vi "User Manual.vi"() -> ()   [LabVIEW 2020, in "Exaprom PDF.lvlib"]
uses:
  <userlib>/labview-PDF-writer-master/Exaprom PDF.lvlib
  <userlib>/labview-PDF-writer-master/Controls/Page Controls/Page setup.ctl
  <userlib>/labview-PDF-writer-master/Controls/Page Controls/Page size.ctl
  <userlib>/labview-PDF-writer-master/Controls/Page Controls/Page Orientation.ctl
  <userlib>/labview-PDF-writer-master/Controls/Page Controls/Page Layout Custom.ctl
  <userlib>/labview-PDF-writer-master/Controls/Page Controls/Page margins.ctl
  <userlib>/labview-PDF-writer-master/Controls/Font Controls/Font complete cluster.ctl
  <userlib>/labview-PDF-writer-master/Controls/Font Controls/Font size.ctl
  <userlib>/labview-PDF-writer-master/Controls/Font Controls/Font color.ctl
  <userlib>/labview-PDF-writer-master/Controls/Font Controls/Type and encoding.ctl
  <userlib>/labview-PDF-writer-master/Controls/Text Controls/Unicode/Type and run direction.ctl
  <userlib>/labview-PDF-writer-master/Controls/Initialization Controls/Defaut Paragraphe and Line Spacing.ctl
  <userlib>/labview-PDF-writer-master/Controls/Text Controls/Texte alignement.ctl
  <userlib>/labview-PDF-writer-master/Controls/Text Controls/Line spacing.ctl
  <userlib>/labview-PDF-writer-master/Controls/Table Controls/Table properties.ctl
  <userlib>/labview-PDF-writer-master/Controls/Table Controls/Table position.ctl
  <userlib>/labview-PDF-writer-master/Controls/Initialization Controls/PDF Details.ctl
  <userlib>/labview-PDF-writer-master/Controls/Header, Footer and Watermark Controls/Header or Footer  Image cluster.ctl
  <userlib>/labview-PDF-writer-master/Controls/Table Controls/Cell Alignment 20px.ctl
  <userlib>/labview-PDF-writer-master/Controls/Header, Footer and Watermark Controls/Header or Footer  Page # cluster.ctl
  <userlib>/labview-PDF-writer-master/Controls/Header, Footer and Watermark Controls/Page number.ctl
  <userlib>/labview-PDF-writer-master/Controls/Font Controls/Font complete cluster horizontal.ctl
  <userlib>/labview-PDF-writer-master/Controls/Header, Footer and Watermark Controls/Header or Footer Line cluster.ctl
  <userlib>/labview-PDF-writer-master/Controls/Header, Footer and Watermark Controls/Header Footer Line.ctl
  <userlib>/labview-PDF-writer-master/Controls/Header, Footer and Watermark Controls/Header or Footer  Text cluster.ctl
  <userlib>/labview-PDF-writer-master/Controls/Initialization Controls/Captions.ctl
  <userlib>/labview-PDF-writer-master/Controls/Initialization Controls/Image or Table Caption.ctl
  <userlib>/labview-PDF-writer-master/Controls/Initialization Controls/Unit.ctl
  <userlib>/labview-PDF-writer-master/Controls/Text Controls/Text and hyperlink [ ].ctl
  <userlib>/labview-PDF-writer-master/Controls/Text Controls/Text from String of File and hyperlink.ctl
  <userlib>/labview-PDF-writer-master/Controls/Text Controls/Paragraph indentation.ctl
  <userlib>/labview-PDF-writer-master/Controls/Image Controls/Image alignment and position.ctl
  <userlib>/labview-PDF-writer-master/Controls/Image Controls/Image aligment.ctl
  <userlib>/labview-PDF-writer-master/Controls/Image Controls/Image border.ctl
  <userlib>/labview-PDF-writer-master/Controls/Table Controls/Row Predefined borders cluster.ctl
  <userlib>/labview-PDF-writer-master/Controls/Table Controls/Row Predefined borders.ctl
  <userlib>/labview-PDF-writer-master/Controls/Image Controls/Image Scale.ctl
  <userlib>/labview-PDF-writer-master/Controls/Table Controls/Cell Font, type, Alignment and LS V2.ctl
  <userlib>/labview-PDF-writer-master/Controls/Table Controls/Cell Type, Alignment and LS.ctl
  <userlib>/labview-PDF-writer-master/Controls/Table Controls/Text vertical arrangement.ctl
  <userlib>/labview-PDF-writer-master/Controls/Table Controls/Row Back Ground color Datas.ctl
  <userlib>/labview-PDF-writer-master/Controls/Header, Footer and Watermark Controls/Watermark Text Cluster.ctl
  <userlib>/labview-PDF-writer-master/Controls/Header, Footer and Watermark Controls/Watermark Position.ctl
  <userlib>/labview-PDF-writer-master/Controls/Header, Footer and Watermark Controls/Header footer horiz alignment.ctl
  <userlib>/labview-PDF-writer-master/Controls/Header, Footer and Watermark Controls/Watermark Image Cluster.ctl
  <userlib>/labview-PDF-writer-master/Controls/Table Controls/Simplified Table Row Borders [ ].ctl
  <userlib>/labview-PDF-writer-master/Controls/Table Controls/Simplified Table Row Borders.ctl
  <userlib>/labview-PDF-writer-master/Controls/Table Controls/Border and BG Color [ ].ctl
  <userlib>/labview-PDF-writer-master/Controls/Table Controls/Border and BG Color.ctl
  <userlib>/labview-PDF-writer-master/Controls/Table Controls/Cell Border 20 px.ctl
  <userlib>/labview-PDF-writer-master/Controls/Concatenate Controls/PDF file to concatenate.ctl
  <userlib>/labview-PDF-writer-master/Controls/Table Controls/Table Appearance and Font Row [ ].ctl
  <userlib>/labview-PDF-writer-master/Controls/Table Controls/One Row Appearance.ctl
  <userlib>/labview-PDF-writer-master/Controls/Table Controls/Row from to.ctl
  <userlib>/labview-PDF-writer-master/Controls/Table Controls/Cell, Alignment, LS and Font - hide Vmerge.ctl
  <userlib>/labview-PDF-writer-master/Controls/Table Controls/Cell Appearance.ctl
  <userlib>/labview-PDF-writer-master/Controls/Table Controls/Merge Horizontal.ctl
  <userlib>/labview-PDF-writer-master/Controls/Table Controls/Merge Vertical.ctl
  <userlib>/labview-PDF-writer-master/Controls/Initialization Controls/File Permission Parameters.ctl
  <userlib>/labview-PDF-writer-master/Controls/Initialization Controls/At the opening.ctl
  <vilib>/Utility/miscctls.llb/LVPointTypeDef.ctl
  <userlib>/labview-PDF-writer-master/Controls/Header, Footer and Watermark Controls/Header or Footer.ctl
  <userlib>/labview-PDF-writer-master/Controls/Chapter Controls/Chapter.ctl
  <userlib>/labview-PDF-writer-master/Controls/Image Controls/Image Size Block Diagram.ctl
  <userlib>/labview-PDF-writer-master/VIs/Low level/Header, Footer and Watermark Low level/Append Text HF.vi
  <userlib>/labview-PDF-writer-master/VIs/Low level/Header, Footer and Watermark Low level/AppendLine seperator.vi
  <userlib>/labview-PDF-writer-master/VIs/Low level/Header, Footer and Watermark Low level/Append Image HF.vi
  <userlib>/labview-PDF-writer-master/VIs/Low level/Header, Footer and Watermark Low level/Append Page number HF.vi
  <userlib>/labview-PDF-writer-master/VIs/Low level/Header, Footer and Watermark Low level/Append Watermark Image.vi
  <userlib>/labview-PDF-writer-master/VIs/Low level/Header, Footer and Watermark Low level/Append Watermark Text.vi
  <userlib>/labview-PDF-writer-master/VIs/Text/Append Paragraph with Link [ ].vi
  <userlib>/labview-PDF-writer-master/VIs/Text/Append Paragraph.vi
  <userlib>/labview-PDF-writer-master/VIs/Text/Append Phrase.vi
  <userlib>/labview-PDF-writer-master/LV Class/PDF Report Class/PDF Report Class.lvclass
panel:
  out "Tab Control":T1(tab)=enum."Table 5"
  in  "Page Setup":T2={"Page Size"=1, "Orientation"=enum."Portrait", "Custom Size"={"Width"=0.0, "Height"=0.0}, "Margins"={"Left"=1.0, "Right"=1.0, "Top"=1.0, "Bottom"=1.0}} caption="页面设置" {"Page Size" items=["Custom", "LETTER", "NOTE", "LEGAL", "TABLOID", "EXECUTIVE", "POSTCARD", "A0", "A1", "A2", "A3", "A4", "A5", "A6", "A7", "A8", "A9", "A10", "B0", "B1", "B2", "B3", "B4", "B5", "B6", "B7", "B8", "B9", "B10", "ARCH_E", "ARCH_D", "ARCH_C", "ARCH_B", "ARCH_A", "FLSA", "FLSE", "HALFLETTER", "_11X17", "ID_1", "ID_2", "ID_3", "LEDGER", "CROWN_QUARTO", "LARGE_CROWN_QUARTO", "DEMY_QUARTO", "ROYAL_QUARTO", "CROWN_OCTAVO", "LARGE_CROWN_OCTAVO", "DEMY_OCTAVO", "ROYAL_OCTAVO", "SMALL_PAPERBACK", "PENGUIN_SMALL_PAPERBACK", "PENGUIN_LARGE_PAPERBACK"]}
  in  "Default Paragraph":T7={" Aligment"=enum."JUSTIFY", "Line spacing"=enum."1.0"} caption="默认段落"
  out "error out":errorcluster
  in  "PDF Details":T10={"Title"="Exaprom PDF 2.0的用户手册", "Author"="三多", "Subject"="这个示例展示了如何使用工具箱Exaprom PDF 2.0创建PDF报告。", "Keywords"="关键词.", "Creator"="Exaprom PDF 2.0"} caption="PDF 详情"
  in  "File or Directory path":path=path "C:/Users/10643/Desktop/123.pdf"
  out "PDF 输出路径":path=path "C:/Users/10643/Desktop/123_22112416.pdf"
  in  "默认字体":T11={"Name"="Arial", "Size"=12.0, "Color"=0, "Style"={"Bold"=FALSE, "Italic"=FALSE, "Underline"=FALSE, "Strikeout"=FALSE}, "Type"={"Type&direction"=enum."ASCII", "Embedded"=FALSE, "Encoding"="gb2312"}}
  in  "Captions":T16={"Figure"={"Caption"="Figure ", "Separator"=":  ", "Position"=enum."Below"}, "Table"={"Caption"="Table ", "Separator"=":  ", "Position"=enum."Above"}, "Font"={"Name"="", "Size"=-1.0, "Color"=0, "Style"={"Bold"=FALSE, "Italic"=FALSE, "Underline"=FALSE, "Strikeout"=FALSE}, "Type"={"Type&direction"=enum."Select", "Embedded"=FALSE, "Encoding"=""}}} caption="标题"
  in  "Unit (默认 = 英寸)":T18 caption="单位 (默认 = 英寸)"
  in  "Overwrite?":bool=TRUE
  out "Progress":u8(slide)=20 scale=0.0..20.0
  in  "Permissions":T19={"User Password"="", "Owner Password"="", "Printing"=enum."Don't Allow Printing", "Allow Modify Contents"=FALSE, "Allow Copy"=FALSE, "Allow Modify Annotations"=FALSE, "Allow Fill In "=FALSE, "Allow Screen Readers"=FALSE, "Allow Assembly"=FALSE} caption="权限"
  in  "At the opening":T20={"Page"=0, "Show Bookmarks"=TRUE} caption="PDF显示方式(自动适应 高，宽显示)" {"Page" items=["Single Page - Fit Page"=1, "Single Page - Fit Width"=0]}
  out "秒":u32=2
  in  "Watermark":enum16{"none", "Image", "Text"}(ring) caption="选择水印方式"
  in  "Footer Page #":T21={"Start at page"=3, "Start with #"=1, "Cell Alignment"=6, "Page #"={"Text 1"="页", "Text 2"="到", "Text 3"="页"}, "Font"={"Name"="Arial", "Size"=10.0, "Color"=0, "Style"={"Bold"=FALSE, "Italic"=FALSE, "Underline"=FALSE, "Strikeout"=FALSE}, "Type"={"Type&direction"=enum."ASCII", "Embedded"=FALSE, "Encoding"=""}}} caption="页码 #"
  in  "Footer Line":T25={"H/F Line"=enum."Horizontal line", "Thickness (point)"=0.75, " Colour"=7171459} caption="页脚线"
  in  "Header Line":T25={"H/F Line"=enum."Horizontal line", "Thickness (point)"=0.75, " Colour"=7171459} caption="页眉线"
  in  "Header Text":T27={"Start at page"=3, "Cell Alignment"=5, "Line spacing"=enum."Select", "Text"="Exaprom PDF 2.0 LabVIEW工具箱\n(with <a>iTextSharp</a> 4.1.6)", "Font complete"={"Name"="", "Size"=14.0, "Color"=0, "Style"={"Bold"=TRUE, "Italic"=FALSE, "Underline"=FALSE, "Strikeout"=FALSE}, "Type"={"Type&direction"=enum."Select", "Embedded"=FALSE, "Encoding"=""}}, "Link"="http://"} caption="标题内容"
  in  "Footer Text":T27={"Start at page"=3, "Cell Alignment"=4, "Line spacing"=enum."Select", "Text"="WWW.OK.SHOW", "Font complete"={"Name"="Segoe Script", "Size"=8.0, "Color"=16711680, "Style"={"Bold"=TRUE, "Italic"=TRUE, "Underline"=FALSE, "Strikeout"=FALSE}, "Type"={"Type&direction"=enum."Select", "Embedded"=FALSE, "Encoding"=""}}, "Link"="http://WWW.OK.SHOW"} caption="页脚文本"
  in  "Watermark Image":T28={"Image path"=path "C:/Program Files (x86)/National Instruments/LabVIEW 2020/user.lib/labview-PDF-writer-master/Examples/Images/Logo Exaprom.jpg", "Opacity (%)"=10.0, "Postion"={"Position"=enum."Center (text section)", "X"=0.0, "Y"=0.0}, "Automatic"=TRUE, "Scale(%)"=100.0, "Rotate(°)"=0.0} caption="水印图像"
  in  "Watermark Text":T30={"Text "="WWW.OK.SHOW", "Opacity (%)"=5.0, "Position"={"Position"=enum."Center (text section)", "X"=0.0, "Y"=0.0}, "Automatic"=TRUE, "Font"={"Font Name"="", "Size"=-1.0, "Color"=0}, "Alignment"=enum."Center", "Rotate(°)"=0.0} caption="水印文本"
  in  "Footer Image":T32={"Start at page"=3, "Cell Alignment"=5, "Path"=path "C:/Program Files (x86)/National Instruments/LabVIEW 2020/user.lib/labview-PDF-writer-master/Examples/Images/Logo Exaprom.jpg", "Image (%)"=15.0, "Link"="http://WWW.OK.SHOW"} caption="页脚图像"
  in  "Text FP1 [ ]":T33=[{"Text"={"Text"="\nExaprom PDF 2.0工具包  \n\n \n\n用户手册 \n\n", "Path"=path "", "Font complete"={"Name"="Arial", "Size"=32.0, "Color"=0, "Style"={"Bold"=TRUE, "Italic"=FALSE, "Underline"=FALSE, "Strikeout"=FALSE}, "Type"={"Type&direction"=enum."ASCII", "Embedded"=FALSE, "Encoding"=""}}}, "Link"={"Hyperlink"="", "Font complete"={"Name"="", "Size"=-1.0, "Color"=255, "Style"={"Bold"=FALSE, "Italic"=TRUE, "Underline"=FALSE, "Strikeout"=FALSE}, "Type"={"Type&direction"=enum."Select", "Embedded"=FALSE, "Encoding"=""}}}, "Paragraphe"={" Aligment"=enum."CENTER", "Line spacing"=enum."Select"}, "Indentation"={"Left"=0.0, "Right"=0.0}}, {"Text"={"Text"="\nPDF Report with iTextSharp 4.1.6\nfor LabVIEW", "Path"=path "", "Font complete"={"Name"="Arial", "Size"=24.0, "Color"=0, "Style"={"Bold"=TRUE, "Italic"=FALSE, "Underline"=FALSE, "Strikeout"=FALSE}, "Type"={"Type&direction"=enum."Select", "Embedded"=FALSE, "Encoding"=""}}}, "Link"={"Hyperlink"="", "Font complete"={"Name"="", "Size"=-1.0, "Color"=255, "Style"={"Bold"=FALSE, "Italic"=TRUE, "Underline"=FALSE, "Strikeout"=FALSE}, "Type"={"Type&direction"=enum."Select", "Embedded"=FALSE, "Encoding"=""}}}, "Paragraphe"={" Aligment"=enum."CENTER", "Line spacing"=enum."Select"}, "Indentation"={"Left"=0.0, "Right"=0.0}}, {"Text"={"Text"="\n\n\n\nby\n\nJean-Marc Simard \n三多（修复汉化)\nQQ：1064331064\n\n\n\n七月-08日-二〇二二年", "Path"=path "", "Font complete"={"Name"="Arial", "Size"=24.0, "Color"=0, "Style"={"Bold"=FALSE, "Italic"=FALSE, "Underline"=FALSE, "Strikeout"=FALSE}, "Type"={"Type&direction"=enum."Select", "Embedded"=FALSE, "Encoding"=""}}}, "Link"={"Hyperlink"="", "Font complete"={"Name"="", "Size"=-1.0, "Color"=255, "Style"={"Bold"=FALSE, "Italic"=TRUE, "Underline"=FALSE, "Strikeout"=FALSE}, "Type"={"Type&direction"=enum."Select", "Embedded"=FALSE, "Encoding"=""}}}, "Paragraphe"={" Aligment"=enum."CENTER", "Line spacing"=enum."Select"}, "Indentation"={"Left"=0.0, "Right"=0.0}}]
  in  "Image FP1":path=path "C:/Program Files/National Instruments/LabVIEW 2009/vi.lib/Exaprom PDF/Examples/Images/Logo Exaprom.jpg"
  in  "TOC Title":string="\n目录\n\n\n"
  in  "TOC Title Font":T11={"Name"="", "Size"=14.0, "Color"=0, "Style"={"Bold"=TRUE, "Italic"=FALSE, "Underline"=FALSE, "Strikeout"=FALSE}, "Type"={"Type&direction"=enum."ASCII", "Embedded"=FALSE, "Encoding"=""}} caption="TOC标题字体"
  in  "TOC Chapter and section Font":T11={"Name"="", "Size"=-1.0, "Color"=0, "Style"={"Bold"=FALSE, "Italic"=FALSE, "Underline"=FALSE, "Strikeout"=FALSE}, "Type"={"Type&direction"=enum."ASCII", "Embedded"=FALSE, "Encoding"=""}} caption="TOC章和节字体"
  in  "Text C8":string="\n虽然这个工具包并没有打算取代文字处理程序，但是作为一个例子，我们使用这个PDF工具包制作了这个文档。VI“用户手册”。vi”在面板“Exaprom PDF 2.0”中可用。"
  in  "Texte C2 [ ]":T33=[{"Text"={"Text"="\n我开发了这个PDF报告生成工具包，因为我希望能够在LabVIEW上生成PDF报告，而不需要购买许可证。 最终的选择是开源的iTextSharp 4.1.6库(<a>Mozilla Public License Version 1.1</a>)。 我开发了一系列VIs，使我可以直接生成PDF报告，而不需要购买商业产品。 选择的许可: \n", "Path"=path "", "Font complete"={"Name"="", "Size"=-1.0, "Color"=0, "Style"={"Bold"=FALSE, "Italic"=FALSE, "Underline"=FALSE, "Strikeout"=FALSE}, "Type"={"Type&direction"=enum."Select", "Embedded"=FALSE, "Encoding"=""}}}, "Link"={"Hyperlink"="http://www.mozilla.org/MPL/MPL-1.1.html", "Font complete"={"Name"="", "Size"=-1.0, "Color"=255, "Style"={"Bold"=FALSE, "Italic"=TRUE, "Underline"=FALSE, "Strikeout"=FALSE}, "Type"={"Type&direction"=enum."Select", "Embedded"=FALSE, "Encoding"=""}}}, "Paragraphe"={" Aligment"=enum."Select", "Line spacing"=enum."Select"}, "Indentation"={"Left"=0.0, "Right"=0.0}}, {"Text"={"Text"="\n<a>BSD(伯克利软件发布许可)</a>允许专有使用，并且对于在该许可下发布的软件可以并入专有产品。 基于该软件作品可以在专有许可下发布或作为封闭源代码软件。”\n", "Path"=path "", "Font complete"={"Name"="", "Size"=-1.0, "Color"=0, "Style"={"Bold"=FALSE, "Italic"=FALSE, "Underline"=FALSE, "Strikeout"=FALSE}, "Type"={"Type&direction"=enum."Select", "Embedded"=FALSE, "Encoding"=""}}}, "Link"={"Hyperlink"="http://fr.wikipedia.org/wiki/Licence_BSD", "Font complete"={"Name"="", "Size"=-1.0, "Color"=255, "Style"={"Bold"=FALSE, "Italic"=TRUE, "Underline"=FALSE, "Strikeout"=FALSE}, "Type"={"Type&direction"=enum."Select", "Embedded"=FALSE, "Encoding"=""}}}, "Paragraphe"={" Aligment"=enum."Select", "Line spacing"=enum."Select"}, "Indentation"={"Left"=0.5, "Right"=0.5}}, {"Text"={"Text"="\n简单地说，你可以对这些VIs做你想做的。\n\n更新的版本，<a>iTextSharp 5。X<a>，在Affero通用公共许可证下，在不披露您自己的应用程序源代码的情况下，涉及iText软件的活动是不免费的。\n\n\n", "Path"=path "", "Font complete"={"Name"="", "Size"=-1.0, "Color"=0, "Style"={"Bold"=FALSE, "Italic"=FALSE, "Underline"=FALSE, "Strikeout"=FALSE}, "Type"={"Type&direction"=enum."Select", "Embedded"=FALSE, "Encoding"=""}}}, "Link"={"Hyperlink"="http://itextpdf.com/terms-of-use/", "Font complete"={"Name"="", "Size"=-1.0, "Color"=255, "Style"={"Bold"=FALSE, "Italic"=TRUE, "Underline"=FALSE, "Strikeout"=FALSE}, "Type"={"Type&direction"=enum."Select", "Embedded"=FALSE, "Encoding"=""}}}, "Paragraphe"={" Aligment"=enum."Select", "Line spacing"=enum."Select"}, "Indentation"={"Left"=0.0, "Right"=0.0}}]
  in  "Texte D2 [ ]":T33=[{"Text"={"Text"="\n\nPDF报告的制作可分为四个步骤:\n\n1)创建报告(PDF文件和默认参数)\n2)添加页眉、页脚和水印(全部可选)\n3)撰写PDF报告，包括添加文本元素、图片(文件、\n控制和前面板)和桌子;\n4)关闭PDF报告\n\n在第5章中，我们回顾了创建PDF报告所需的不同VI。\n\n", "Path"=path "", "Font complete"={"Name"="", "Size"=-1.0, "Color"=0, "Style"={"Bold"=FALSE, "Italic"=FALSE, "Underline"=FALSE, "Strikeout"=FALSE}, "Type"={"Type&direction"=enum."Select", "Embedded"=FALSE, "Encoding"=""}}}, "Link"={"Hyperlink"="", "Font complete"={"Name"="", "Size"=-1.0, "Color"=255, "Style"={"Bold"=FALSE, "Italic"=TRUE, "Underline"=FALSE, "Strikeout"=FALSE}, "Type"={"Type&direction"=enum."Select", "Embedded"=FALSE, "Encoding"=""}}}, "Paragraphe"={" Aligment"=enum."Select", "Line spacing"=enum."Select"}, "Indentation"={"Left"=0.0, "Right"=0.0}}]
  in  "Text C6":string="重启LabVIEW后，面板“Exaprom PDF 2.0”将出现。\n\n"
  in  "Text C1":string="产品介绍"
  in  "Text C3":string="产品介绍"
  in  "Texte C4 [ ]":T33=[{"Text"={"Text"="\n解压“ExapromPDF2.0.ZIP”之后，您将得到一个文件夹和一个文件\n\n     1)\tExaprom PDF文件夹;\n     2)\t还有exaprompdf.mnu文件。\n\n\n", "Path"=path "", "Font complete"={"Name"="", "Size"=-1.0, "Color"=0, "Style"={"Bold"=FALSE, "Italic"=FALSE, "Underline"=FALSE, "Strikeout"=FALSE}, "Type"={"Type&direction"=enum."Select", "Embedded"=FALSE, "Encoding"=""}}}, "Link"={"Hyperlink"="", "Font complete"={"Name"="", "Size"=-1.0, "Color"=16777222, "Style"={"Bold"=TRUE, "Italic"=FALSE, "Underline"=FALSE, "Strikeout"=FALSE}, "Type"={"Type&direction"=enum."Select", "Embedded"=FALSE, "Encoding"=""}}}, "Paragraphe"={" Aligment"=enum."LEFT", "Line spacing"=enum."Select"}, "Indentation"={"Left"=0.0, "Right"=0.0}}]
  in  "Text C5":string="\n\n“Exaprom PDF”文件夹必须放在(参见图2):\n\nC:\\Program Files\\National Instruments\\LabVIEW Version\\vi.lib\\\n\n"
  in  "Text C7":string="\nexaprompdf文件”.Mnu \"必须放在(见图3):\n\nC:\\Program Files\\National Instruments\\LabVIEW Version\\\n                                                                                     menus\\Categories\\Programming\\"
  in  "Text D1":string="PDF报告(简化)"
  in  "Texte E2 [ ]":T33=[{"Text"={"Text"="\n\n用于生成PDF报告的库是iTextSharp。\n\n本库使用点(72点= 1英寸= 25.4毫米)，但您将使用您选择的单位(英寸或毫米-章节5.4)，除非单位“点”被明确指出。字体是个例外:单位就是点。\n\n页面的原点在左下角(见下图)。\n\n文本框是减去页边距(下图中的蓝色矩形)的页面。\n\n\n", "Path"=path "", "Font complete"={"Name"="", "Size"=-1.0, "Color"=0, "Style"={"Bold"=FALSE, "Italic"=FALSE, "Underline"=FALSE, "Strikeout"=FALSE}, "Type"={"Type&direction"=enum."Select", "Embedded"=FALSE, "Encoding"=""}}}, "Link"={"Hyperlink"="", "Font complete"={"Name"="", "Size"=-1.0, "Color"=255, "Style"={"Bold"=FALSE, "Italic"=TRUE, "Underline"=FALSE, "Strikeout"=FALSE}, "Type"={"Type&direction"=enum."Select", "Embedded"=FALSE, "Encoding"=""}}}, "Paragraphe"={" Aligment"=enum."Select", "Line spacing"=enum."Select"}, "Indentation"={"Left"=0.0, "Right"=0.0}}]
  in  "Text E1":string="一般"
  in  "Text F2":string="“文本”面板"
  in  "Text F1":string="不同的调色板"
  in  "Texte F3 [ ]":T33=[{"Text"={"Text"="\n\n您可以访问目录中包含的字体C: \\ Windows \\ Fonts (你应该检查版权). 此外，你还有iTextSharp自动提供的字体:Courier, Helvetica, Symbol, Times-Roman和ZapfDingbats。\n\n当创建PDF报告时，我们指定默认字体为Arial 12点(粗体、斜体、下划线和删除线= F)，类型和方向= ASCII，字符编码= CP1252(拉丁字母)。该信息存储在LV类“PDF报告”中。文本面板中所有VI的字体参数为:\n\n- Name =空字符串;\n- Size = -1;\n-粗体，斜体，下划线和删除线= F;\n-类型&方向=选择;\n- E(内嵌)= F;\n- Encoding =空字符串。\n\n当字体名称为空时，将使用默认字体的名称。当字体大小的值为-1时，则使用默认的字体大小。当Type&direction的值设置为Select时，将使用默认字体的Type&direction。当Encoding的值为空时，将使用默认字体的Encoding。\n", "Path"=path "", "Font complete"={"Name"="", "Size"=-1.0, "Color"=0, "Style"={"Bold"=FALSE, "Italic"=FALSE, "Underline"=FALSE, "Strikeout"=FALSE}, "Type"={"Type&direction"=enum."Select", "Embedded"=FALSE, "Encoding"=""}}}, "Link"={"Hyperlink"="", "Font complete"={"Name"="", "Size"=-1.0, "Color"=255, "Style"={"Bold"=FALSE, "Italic"=TRUE, "Underline"=FALSE, "Strikeout"=FALSE}, "Type"={"Type&direction"=enum."Select", "Embedded"=FALSE, "Encoding"=""}}}, "Paragraphe"={" Aligment"=enum."Select", "Line spacing"=enum."Select"}, "Indentation"={"Left"=0.0, "Right"=0.0}}]
  in  "Text F6":string="在创建PDF报告时，我们指定默认对齐方式为“JUSTIFY”，默认行间距为1.0。该信息也存储在LV类“PDF报告”中。\n\n当对齐方式设置为“选择”时，将使用默认对齐方式。当间距保留为“选择”时，使用默认的行间距。\n\n"
  in  "Text F8 [ ]":T33=[{"Text"={"Text"="此标签允许您像 <img src=\"Arrow\"/> 一样插入图像“Arrow.jpg”。 要插入带有链接 <a><img src=\"Logo\"/></a> 的图像“Logo E.jpg”，您应该使用“Append Paragraph & Link [ ].vi”。 所有这些段落都以换行符自动终止。\n\n", "Path"=path "", "Font complete"={"Name"="", "Size"=-1.0, "Color"=0, "Style"={"Bold"=FALSE, "Italic"=FALSE, "Underline"=FALSE, "Strikeout"=FALSE}, "Type"={"Type&direction"=enum."Select", "Embedded"=FALSE, "Encoding"=""}}}, "Link"={"Hyperlink"="http://www.exaprom.com/", "Font complete"={"Name"="", "Size"=-1.0, "Color"=255, "Style"={"Bold"=FALSE, "Italic"=TRUE, "Underline"=FALSE, "Strikeout"=FALSE}, "Type"={"Type&direction"=enum."Select", "Embedded"=FALSE, "Encoding"=""}}}, "Paragraphe"={" Aligment"=enum."Select", "Line spacing"=enum."Select"}, "Indentation"={"Left"=0.0, "Right"=0.0}}, {"Text"={"Text"="第三个，“Append Phrase.vi”（数字“4”），添加了一个短语，但没有换行符和左对齐。 此外，除了“Append Phrase.vi”之外，还可以有段落缩进（左右）。\n", "Path"=path "", "Font complete"={"Name"="", "Size"=-1.0, "Color"=0, "Style"={"Bold"=FALSE, "Italic"=FALSE, "Underline"=FALSE, "Strikeout"=FALSE}, "Type"={"Type&direction"=enum."Select", "Embedded"=FALSE, "Encoding"=""}}}, "Link"={"Hyperlink"="", "Font complete"={"Name"="", "Size"=-1.0, "Color"=255, "Style"={"Bold"=FALSE, "Italic"=TRUE, "Underline"=FALSE, "Strikeout"=FALSE}, "Type"={"Type&direction"=enum."Select", "Embedded"=FALSE, "Encoding"=""}}}, "Paragraphe"={" Aligment"=enum."Select", "Line spacing"=enum."Select"}, "Indentation"={"Left"=0.0, "Right"=0.0}}]
  in  "Text F7":string="有三个VIs添加文本，他们被分组在VI“追加文本多态”。Vi”(上图中的数字“1”)。\n\n第一个是“附加段落”。Vi“(数字“2”)，可以将文本添加为段落，文本将自动以换行结束。\n\n第二个或“附加段落&链接[]”。Vi\"(数字\"3\")，添加了一个段落序列，该序列具有特殊性，可以将链接(http://www.mywebsite.com/ ou mailto:name@example.com)与文本关联，放置在标签< a> </ a>之间。 \n\n此外，\"Append Paragraph. vi”和Append Paragraph & Link [ ].  Vi\"以在带有标签的段落中插入图像 <img src=\"Image name\"/>.\n"
  in  "Text F5":string="\n字符编码可以是ASCII或Unicode (UTF-16)。写入方向(仅适用于Unicode)为:\n\n- UTF-16 \"UTF-16字符，从左到右书写\";\n——utf - 16(默认)“使用默认运行方向”;\nutf - 16 (LTR)使用从左到右的双向重新排序\n运行方向”;\nutf - 16 (RTL)“使用从右到左优先级的双向重新排序\n运行方向”。\n\n"
  in  "Text F4":string="集群字体可以是垂直的，也可以是水平的。\n"
  in  "Text G4":string="\n可用的选择是：\n1) 绝对值 (X, Y)，单位为 mm；\n2) 左;\n3) 中心；\n4) 对；\n5) 左 (TextWrap)\n6) 右 (TextWrap)。\n“左（TextWrap）”表示图像放在左边，文本放在右边。 “右（TextWrap）”表示图片放在右边，文字放在左边。 缩进仅适用于“TextWrap”，它是我们在图像和文本之间留下的水平空间。 我们也可以选择给图片加边框。\n"
  in  "Texte G3 [ ]":T33=[{"Text"={"Text"="\n图像调色板有 4 个 VI：\n\n          1）“附加控制图像.vi”；\n          2）“附加前面板Image.vi”。\n          3）“附加框图Image.vi”；\n          4）“附加图像文件.vi”。\n\n下图我们有图片属性的控件（这个图片已经添加了“Append Control Image.vi）。我们可以缩小或放大图片的大小（比例百分比）。如果图片大于 文本区域（页面大小减去边距），大小将自动调整以适应。", "Path"=path "", "Font complete"={"Name"="", "Size"=-1.0, "Color"=0, "Style"={"Bold"=FALSE, "Italic"=FALSE, "Underline"=FALSE, "Strikeout"=FALSE}, "Type"={"Type&direction"=enum."Select", "Embedded"=FALSE, "Encoding"=""}}}, "Link"={"Hyperlink"="", "Font complete"={"Name"="", "Size"=-1.0, "Color"=255, "Style"={"Bold"=FALSE, "Italic"=TRUE, "Underline"=FALSE, "Strikeout"=FALSE}, "Type"={"Type&direction"=enum."Select", "Embedded"=FALSE, "Encoding"=""}}}, "Paragraphe"={" Aligment"=enum."Select", "Line spacing"=enum."Select"}, "Indentation"={"Left"=0.0, "Right"=0.0}}, {"Text"={"Text"="\n我们可以选择图像的水平位置，只要我们没有添加标题，因为在这种情况下，它总是水平居中。", "Path"=path "", "Font complete"={"Name"="", "Size"=-1.0, "Color"=0, "Style"={"Bold"=FALSE, "Italic"=FALSE, "Underline"=FALSE, "Strikeout"=FALSE}, "Type"={"Type&direction"=enum."Select", "Embedded"=FALSE, "Encoding"=""}}}, "Link"={"Hyperlink"="", "Font complete"={"Name"="", "Size"=-1.0, "Color"=255, "Style"={"Bold"=FALSE, "Italic"=TRUE, "Underline"=FALSE, "Strikeout"=FALSE}, "Type"={"Type&direction"=enum."Select", "Embedded"=FALSE, "Encoding"=""}}}, "Paragraphe"={" Aligment"=enum."Select", "Line spacing"=enum."Select"}, "Indentation"={"Left"=0.0, "Right"=0.0}}]
  in  "Texte G2 [ ]":T33=[{"Text"={"Text"="\n放置在 PDF 中的图像可以缩小或放大，但这只是一个视图问题：它们将始终占据 PDF 文件中的相同空间。\n", "Path"=path "", "Font complete"={"Name"="", "Size"=-1.0, "Color"=0, "Style"={"Bold"=FALSE, "Italic"=FALSE, "Underline"=FALSE, "Strikeout"=FALSE}, "Type"={"Type&direction"=enum."Select", "Embedded"=FALSE, "Encoding"=""}}}, "Link"={"Hyperlink"="", "Font complete"={"Name"="", "Size"=-1.0, "Color"=255, "Style"={"Bold"=FALSE, "Italic"=TRUE, "Underline"=FALSE, "Strikeout"=FALSE}, "Type"={"Type&direction"=enum."Select", "Embedded"=FALSE, "Encoding"=""}}}, "Paragraphe"={" Aligment"=enum."Select", "Line spacing"=enum."Select"}, "Indentation"={"Left"=0.0, "Right"=0.0}}]
  in  "Text G1":string="“图像”调色板"
  in  "Text H3":string="要创建一个表，有六个变量，包括五个可选：\n\n               1）表格columnWidth [ ]（可选）；\n               2）重复标题列（可选）\n               3) 列标题 2D [ ]（可选）；\n               4) 行标题 1D [ ]（可选）；\n               5) 文本数据 2D [ ]（必填）；\n               6) 要添加的图像 [ ]（可选）。\n\n第一个指定每列的宽度。如果表格有多个页面，则第二个提供了在每个新页面上重复列标题的可能性。第三是列标题。第四个是行标题。第五个是文本数据，最后一个允许您在表格单元格中插入图像。应该注意的是，一个单元格可以包含文本或图像，但不能同时包含两者。\n\n列数由“Column Headers 2D [ ]”、“Row Headers 1D”和“Text Data 2D [ ]”连接后的列数定义。\n\n如果变量“Table columnWidht [ ]”未连接，则每列的宽度将相同，等于页面宽度（减去边距）除以列数（表 2 与第 21 页的表 3 ）。如果变量“Table columnWidht []”的元素多于列数，则仅使用第一个元素。如果变量“Table columnWidht [ ]”的元素少于列数，则将添加 25 mm 的列。\n\n如果表格的总宽度大于文本区域的宽度，则每列的宽度将按比例缩小，使表格的宽度等于文本区域的宽度。\n\n和图片一样，如果我们没有添加任何标题，我们可以选择水平位置，因为在这种情况下，表格总是水平居中的。"
  in  "Texte H2 [ ]":T33=[{"Text"={"Text"="\n添加表格分两步完成：首先，使用“Create Table.vi”创建表格，然后使用“Append Table.vi”或“Append Customized Table.vi”添加表格。\n\n", "Path"=path "", "Font complete"={"Name"="", "Size"=-1.0, "Color"=0, "Style"={"Bold"=FALSE, "Italic"=FALSE, "Underline"=FALSE, "Strikeout"=FALSE}, "Type"={"Type&direction"=enum."Select", "Embedded"=FALSE, "Encoding"=""}}}, "Link"={"Hyperlink"="", "Font complete"={"Name"="", "Size"=-1.0, "Color"=255, "Style"={"Bold"=FALSE, "Italic"=TRUE, "Underline"=FALSE, "Strikeout"=FALSE}, "Type"={"Type&direction"=enum."Select", "Embedded"=FALSE, "Encoding"=""}}}, "Paragraphe"={" Aligment"=enum."Select", "Line spacing"=enum."Select"}, "Indentation"={"Left"=0.0, "Right"=0.0}}]
  in  "Text H7 [ ]":T33=[{"Text"={"Text"="变量“Costum Borders”逐列定义每个单元格的边框类型。 在 iTextSharp 中，有 16 个选项，从没有线到四边都有线。 我们还可以定义每个单元格的背景颜色。\n\n变量 <img src=\"Row1\"/> 用于逐行格式化表格。 值 -2 表示倒数第二行。 例如，<img src=\"Row2\"/> i 表示将格式应用于第 0 行到倒数第二行。 值 -1 表示最后一行。 例如，<img src=\"Row3\"/> 表示格式应用于最后一行。\n\n", "Path"=path "", "Font complete"={"Name"="", "Size"=-1.0, "Color"=0, "Style"={"Bold"=FALSE, "Italic"=FALSE, "Underline"=FALSE, "Strikeout"=FALSE}, "Type"={"Type&direction"=enum."Select", "Embedded"=FALSE, "Encoding"=""}}}, "Link"={"Hyperlink"="", "Font complete"={"Name"="", "Size"=-1.0, "Color"=255, "Style"={"Bold"=FALSE, "Italic"=TRUE, "Underline"=FALSE, "Strikeout"=FALSE}, "Type"={"Type&direction"=enum."Select", "Embedded"=FALSE, "Encoding"=""}}}, "Paragraphe"={" Aligment"=enum."Select", "Line spacing"=enum."Select"}, "Indentation"={"Left"=0.0, "Right"=0.0}}]
  in  "Texte H4 [ ]":T33=[{"Text"={"Text"="\n如果表格的总宽度大于文本区域的宽度，则每列的宽度将按比例缩小，使表格的宽度等于文本区域的宽度。\n\n和图片一样，如果我们没有添加任何标题，我们可以选择水平位置，因为在这种情况下，表格总是水平居中的。\n", "Path"=path "", "Font complete"={"Name"="", "Size"=-1.0, "Color"=0, "Style"={"Bold"=FALSE, "Italic"=FALSE, "Underline"=FALSE, "Strikeout"=FALSE}, "Type"={"Type&direction"=enum."Select", "Embedded"=FALSE, "Encoding"=""}}}, "Link"={"Hyperlink"="", "Font complete"={"Name"="", "Size"=-1.0, "Color"=255, "Style"={"Bold"=FALSE, "Italic"=TRUE, "Underline"=FALSE, "Strikeout"=FALSE}, "Type"={"Type&direction"=enum."Select", "Embedded"=FALSE, "Encoding"=""}}}, "Paragraphe"={" Aligment"=enum."Select", "Line spacing"=enum."Select"}, "Indentation"={"Left"=0.0, "Right"=0.0}}, {"Text"={"Text"="\n使用“Column Headers 2D [ ]”、“Row Headers 1D [ ]”和“Text Data 2D [ ]”生成的最终表格如下图所示。\n\n", "Path"=path "", "Font complete"={"Name"="", "Size"=-1.0, "Color"=0, "Style"={"Bold"=FALSE, "Italic"=FALSE, "Underline"=FALSE, "Strikeout"=FALSE}, "Type"={"Type&direction"=enum."Select", "Embedded"=FALSE, "Encoding"=""}}}, "Link"={"Hyperlink"="", "Font complete"={"Name"="", "Size"=-1.0, "Color"=255, "Style"={"Bold"=FALSE, "Italic"=TRUE, "Underline"=FALSE, "Strikeout"=FALSE}, "Type"={"Type&direction"=enum."Select", "Embedded"=FALSE, "Encoding"=""}}}, "Paragraphe"={" Aligment"=enum."Select", "Line spacing"=enum."Select"}, "Indentation"={"Left"=0.0, "Right"=0.0}}]
  in  "Text H8":string="我们还可以使用“Append Customized Table.vi”附加一个表格。 它不是很直观，但您有更多的灵活性，例如水平合并（见表 5）。\n"
  in  "Text H5":string="当我们使用“Append Table.vi”将表格添加到文档中时，如果我们排除“PDF Table”，则有八个变量（都是可选的）：\n                1) 行背景颜色\n                2) 预定义边界；\n                3) 列标题格式；\n                4) 表属性；\n                5) 字幕；\n                6) 行头格式；\n                7) 数据格式；\n                8) 自定义表格边框。\n\n第一个提供了在每个 X 行添加背景颜色的可能性。 第二个提供了可用边框类型的选择：预定义和自定义。 如果选择自定义类型，则必须使用变量“自定义表格边框”来定义表格单元格的边框。\n\n"
  in  "Text H6":string="第三，第六和第七分别是列标题，行标题和数据的单元格格式。"
  in  "Text H1":string="“表”调色板"
  in  "Texte I6 [ ]":T33=[{"Text"={"Text"="\nix) 打开生成的PDF文件\n\nPDF 文件的打开方式。\n\n", "Path"=path "", "Font complete"={"Name"="", "Size"=-1.0, "Color"=0, "Style"={"Bold"=FALSE, "Italic"=FALSE, "Underline"=FALSE, "Strikeout"=FALSE}, "Type"={"Type&direction"=enum."Select", "Embedded"=FALSE, "Encoding"=""}}}, "Link"={"Hyperlink"="", "Font complete"={"Name"="", "Size"=-1.0, "Color"=255, "Style"={"Bold"=FALSE, "Italic"=TRUE, "Underline"=FALSE, "Strikeout"=FALSE}, "Type"={"Type&direction"=enum."Select", "Embedded"=FALSE, "Encoding"=""}}}, "Paragraphe"={" Aligment"=enum."Select", "Line spacing"=enum."Select"}, "Indentation"={"Left"=0.0, "Right"=0.0}}, {"Text"={"Text"="b) 使用“Close PDF.vi”关闭 PDF 报告", "Path"=path "", "Font complete"={"Name"="", "Size"=-1.0, "Color"=0, "Style"={"Bold"=TRUE, "Italic"=FALSE, "Underline"=FALSE, "Strikeout"=FALSE}, "Type"={"Type&direction"=enum."Select", "Embedded"=FALSE, "Encoding"=""}}}, "Link"={"Hyperlink"="", "Font complete"={"Name"="", "Size"=-1.0, "Color"=255, "Style"={"Bold"=FALSE, "Italic"=TRUE, "Underline"=FALSE, "Strikeout"=FALSE}, "Type"={"Type&direction"=enum."Select", "Embedded"=FALSE, "Encoding"=""}}}, "Paragraphe"={" Aligment"=enum."Select", "Line spacing"=enum."Select"}, "Indentation"={"Left"=0.0, "Right"=0.0}}, {"Text"={"Text"="\n该VI用于完成报告PDF的编写。 他关闭了编写 PDF 文件所需的各种参考，它会写入页眉、页脚和水印（如果需要）并关闭 PDF。\n\n", "Path"=path "", "Font complete"={"Name"="", "Size"=-1.0, "Color"=0, "Style"={"Bold"=FALSE, "Italic"=FALSE, "Underline"=FALSE, "Strikeout"=FALSE}, "Type"={"Type&direction"=enum."Select", "Embedded"=FALSE, "Encoding"=""}}}, "Link"={"Hyperlink"="", "Font complete"={"Name"="", "Size"=-1.0, "Color"=255, "Style"={"Bold"=FALSE, "Italic"=TRUE, "Underline"=FALSE, "Strikeout"=FALSE}, "Type"={"Type&direction"=enum."Select", "Embedded"=FALSE, "Encoding"=""}}}, "Paragraphe"={" Aligment"=enum."Select", "Line spacing"=enum."Select"}, "Indentation"={"Left"=0.0, "Right"=0.0}}, {"Text"={"Text"="c) 使用“Append New Page.vi”添加分页符", "Path"=path "", "Font complete"={"Name"="", "Size"=-1.0, "Color"=0, "Style"={"Bold"=TRUE, "Italic"=FALSE, "Underline"=FALSE, "Strikeout"=FALSE}, "Type"={"Type&direction"=enum."Select", "Embedded"=FALSE, "Encoding"=""}}}, "Link"={"Hyperlink"="", "Font complete"={"Name"="", "Size"=-1.0, "Color"=255, "Style"={"Bold"=FALSE, "Italic"=TRUE, "Underline"=FALSE, "Strikeout"=FALSE}, "Type"={"Type&direction"=enum."Select", "Embedded"=FALSE, "Encoding"=""}}}, "Paragraphe"={" Aligment"=enum."Select", "Line spacing"=enum."Select"}, "Indentation"={"Left"=0.0, "Right"=0.0}}, {"Text"={"Text"="\n该 VI 在 PDF 文档中添加分页符。\n\n", "Path"=path "", "Font complete"={"Name"="", "Size"=-1.0, "Color"=0, "Style"={"Bold"=FALSE, "Italic"=FALSE, "Underline"=FALSE, "Strikeout"=FALSE}, "Type"={"Type&direction"=enum."Select", "Embedded"=FALSE, "Encoding"=""}}}, "Link"={"Hyperlink"="", "Font complete"={"Name"="", "Size"=-1.0, "Color"=255, "Style"={"Bold"=FALSE, "Italic"=TRUE, "Underline"=FALSE, "Strikeout"=FALSE}, "Type"={"Type&direction"=enum."Select", "Embedded"=FALSE, "Encoding"=""}}}, "Paragraphe"={" Aligment"=enum."Select", "Line spacing"=enum."Select"}, "Indentation"={"Left"=0.0, "Right"=0.0}}, {"Text"={"Text"="d) 通过使用“Page Set Size.vi”更改页面属性来添加分节符（新页面）", "Path"=path "", "Font complete"={"Name"="", "Size"=-1.0, "Color"=0, "Style"={"Bold"=TRUE, "Italic"=FALSE, "Underline"=FALSE, "Strikeout"=FALSE}, "Type"={"Type&direction"=enum."Select", "Embedded"=FALSE, "Encoding"=""}}}, "Link"={"Hyperlink"="", "Font complete"={"Name"="", "Size"=-1.0, "Color"=255, "Style"={"Bold"=FALSE, "Italic"=TRUE, "Underline"=FALSE, "Strikeout"=FALSE}, "Type"={"Type&direction"=enum."Select", "Embedded"=FALSE, "Encoding"=""}}}, "Paragraphe"={" Aligment"=enum."Select", "Line spacing"=enum."Select"}, "Indentation"={"Left"=0.0, "Right"=0.0}}, {"Text"={"Text"="\n该 VI 在 PDF 文档中添加分页符，并可以更改新页面的属性。 只要您不使用“Set Page Size.vi”，这些新属性就适用于所有新页面。\n\n", "Path"=path "", "Font complete"={"Name"="", "Size"=-1.0, "Color"=0, "Style"={"Bold"=FALSE, "Italic"=FALSE, "Underline"=FALSE, "Strikeout"=FALSE}, "Type"={"Type&direction"=enum."Select", "Embedded"=FALSE, "Encoding"=""}}}, "Link"={"Hyperlink"="", "Font complete"={"Name"="", "Size"=-1.0, "Color"=255, "Style"={"Bold"=FALSE, "Italic"=TRUE, "Underline"=FALSE, "Strikeout"=FALSE}, "Type"={"Type&direction"=enum."Select", "Embedded"=FALSE, "Encoding"=""}}}, "Paragraphe"={" Aligment"=enum."Select", "Line spacing"=enum."Select"}, "Indentation"={"Left"=0.0, "Right"=0.0}}, {"Text"={"Text"="e) 使用“Set Default Font.vi”更改默认字体", "Path"=path "", "Font complete"={"Name"="", "Size"=-1.0, "Color"=0, "Style"={"Bold"=TRUE, "Italic"=FALSE, "Underline"=FALSE, "Strikeout"=FALSE}, "Type"={"Type&direction"=enum."Select", "Embedded"=FALSE, "Encoding"=""}}}, "Link"={"Hyperlink"="", "Font complete"={"Name"="", "Size"=-1.0, "Color"=255, "Style"={"Bold"=FALSE, "Italic"=TRUE, "Underline"=FALSE, "Strikeout"=FALSE}, "Type"={"Type&direction"=enum."Select", "Embedded"=FALSE, "Encoding"=""}}}, "Paragraphe"={" Aligment"=enum."Select", "Line spacing"=enum."Select"}, "Indentation"={"Left"=0.0, "Right"=0.0}}, {"Text"={"Text"="\n该 VI 更改默认字体。\n\n", "Path"=path "", "Font complete"={"Name"="", "Size"=-1.0, "Color"=0, "Style"={"Bold"=FALSE, "Italic"=FALSE, "Underline"=FALSE, "Strikeout"=FALSE}, "Type"={"Type&direction"=enum."Select", "Embedded"=FALSE, "Encoding"=""}}}, "Link"={"Hyperlink"="", "Font complete"={"Name"="", "Size"=-1.0, "Color"=255, "Style"={"Bold"=FALSE, "Italic"=TRUE, "Underline"=FALSE, "Strikeout"=FALSE}, "Type"={"Type&direction"=enum."Select", "Embedded"=FALSE, "Encoding"=""}}}, "Paragraphe"={" Aligment"=enum."Select", "Line spacing"=enum."Select"}, "Indentation"={"Left"=0.0, "Right"=0.0}}, {"Text"={"Text"="f) 使用“Print PDF.vi”打印 PDF 报告", "Path"=path "", "Font complete"={"Name"="", "Size"=-1.0, "Color"=0, "Style"={"Bold"=TRUE, "Italic"=FALSE, "Underline"=FALSE, "Strikeout"=FALSE}, "Type"={"Type&direction"=enum."Select", "Embedded"=FALSE, "Encoding"=""}}}, "Link"={"Hyperlink"="", "Font complete"={"Name"="", "Size"=-1.0, "Color"=255, "Style"={"Bold"=FALSE, "Italic"=TRUE, "Underline"=FALSE, "Strikeout"=FALSE}, "Type"={"Type&direction"=enum."Select", "Embedded"=FALSE, "Encoding"=""}}}, "Paragraphe"={" Aligment"=enum."Select", "Line spacing"=enum."Select"}, "Indentation"={"Left"=0.0, "Right"=0.0}}, {"Text"={"Text"="\n该 VI 不基于 iTextSharp 库。\n", "Path"=path "", "Font complete"={"Name"="", "Size"=-1.0, "Color"=0, "Style"={"Bold"=FALSE, "Italic"=FALSE, "Underline"=FALSE, "Strikeout"=FALSE}, "Type"={"Type&direction"=enum."Select", "Embedded"=FALSE, "Encoding"=""}}}, "Link"={"Hyperlink"="", "Font complete"={"Name"="", "Size"=-1.0, "Color"=255, "Style"={"Bold"=FALSE, "Italic"=TRUE, "Underline"=FALSE, "Strikeout"=FALSE}, "Type"={"Type&direction"=enum."Select", "Embedded"=FALSE, "Encoding"=""}}}, "Paragraphe"={" Aligment"=enum."Select", "Line spacing"=enum."Select"}, "Indentation"={"Left"=0.0, "Right"=0.0}}]
  in  "Texte I4":string="\n\ni) 字幕的通用名称\n\n您可以为图形标题和表格指定通用名称。如果您在 Figure.Caption \"Figure\" 和 Figure.Separator \":\" 中写入，那么对于您添加标题的每张（或多张图片），它将被写入 PDF 文档：“图 1：图 1 的标题” 、“图2：图2的说明文字”等。编号是自动的。\nii) 单位（默认 = mm）\n\nPDF 报告中使用的基本单位（毫米或英寸）\n\niii) 文件路径或目录\n\n如果只指定目录，程序运行时会出现一个对话框，询问要使用的文件名。\n\niv) 默认字体\n\n这是在未指定其他字体时文档中使用的字体（名称、颜色、大小和样式）。字体名称是一个字符串。可用的字体是那些出现在目录“C:\\Windows\\Fonts”中的字体。如果您指定的字体不可用或拼写错误，则将替换为“Helvetica”字体。\n\nv) 行距和文本对齐\n \n您可以选择行距 1.0、1.5 和 2.0。文本对齐方式可以是：居中、两端对齐、左对齐或右对齐。\n\nvi) 页面设置\n\n您可以选择页面大小（默认或非默认）、方向和边距。如果选择的格式是“自定义”，那么您必须指定宽度 X（毫米或英寸）和高度 Y（毫米或英寸）。此格式将在文档中使用，因为您不会更改页面大小。\n\nvii) PDF 的元数据（PDF 详细信息）\n\n这是您在查看您创建的 PDF 文件中的属性时看到的元数据（文件>>属性和描述选项卡）。\n\n"
  in  "Texte I3 [ ]":T33=[{"Text"={"Text"="a) 使用“New PDF.vi”创建新的 PDF 报告", "Path"=path "", "Font complete"={"Name"="", "Size"=-1.0, "Color"=0, "Style"={"Bold"=TRUE, "Italic"=FALSE, "Underline"=FALSE, "Strikeout"=FALSE}, "Type"={"Type&direction"=enum."Select", "Embedded"=FALSE, "Encoding"=""}}}, "Link"={"Hyperlink"="", "Font complete"={"Name"="", "Size"=-1.0, "Color"=255, "Style"={"Bold"=FALSE, "Italic"=TRUE, "Underline"=FALSE, "Strikeout"=FALSE}, "Type"={"Type&direction"=enum."Select", "Embedded"=FALSE, "Encoding"=""}}}, "Paragraphe"={" Aligment"=enum."Select", "Line spacing"=enum."Select"}, "Indentation"={"Left"=0.0, "Right"=0.0}}, {"Text"={"Text"="\n第一步是创建一个新的 PDF 报告。 PDF 报告中的变量是：\n\n           i) 图表标题的通用名称；\n           ii) 使用的单位；\n           iii) 要使用的目录或文件名（完整路径）；\n           iv) 文档的默认字体；\n           v) 文档的行距和默认对齐方式；\n           vi) 页面的格式；\n           vii) 有关创建的 PDF 文件的元数据；\n           viii) 文件权限；\n           ix) 打开生成的PDF文件\n", "Path"=path "", "Font complete"={"Name"="", "Size"=-1.0, "Color"=0, "Style"={"Bold"=FALSE, "Italic"=FALSE, "Underline"=FALSE, "Strikeout"=FALSE}, "Type"={"Type&direction"=enum."Select", "Embedded"=FALSE, "Encoding"=""}}}, "Link"={"Hyperlink"="", "Font complete"={"Name"="", "Size"=-1.0, "Color"=255, "Style"={"Bold"=FALSE, "Italic"=TRUE, "Underline"=FALSE, "Strikeout"=FALSE}, "Type"={"Type&direction"=enum."Select", "Embedded"=FALSE, "Encoding"=""}}}, "Paragraphe"={" Aligment"=enum."Select", "Line spacing"=enum."Select"}, "Indentation"={"Left"=0.0, "Right"=0.0}}]
  in  "Texte I2 [ ]":T33=[{"Text"={"Text"="\n文档调色板由 6 个 VI 组成：\n\na) 新的 PDF.vi；\nb) 关闭 PDF.vi；\nc) 追加新页面.vi；\nd) 设置页面大小.vi；\ne) 设置默认字体.vi；\nf) 打印 PDF.vi。", "Path"=path "", "Font complete"={"Name"="", "Size"=-1.0, "Color"=0, "Style"={"Bold"=FALSE, "Italic"=FALSE, "Underline"=FALSE, "Strikeout"=FALSE}, "Type"={"Type&direction"=enum."Select", "Embedded"=FALSE, "Encoding"=""}}}, "Link"={"Hyperlink"="", "Font complete"={"Name"="", "Size"=-1.0, "Color"=255, "Style"={"Bold"=FALSE, "Italic"=TRUE, "Underline"=FALSE, "Strikeout"=FALSE}, "Type"={"Type&direction"=enum."Select", "Embedded"=FALSE, "Encoding"=""}}}, "Paragraphe"={" Aligment"=enum."Select", "Line spacing"=enum."Select"}, "Indentation"={"Left"=0.0, "Right"=0.0}}]
  in  "Texte I5":string="viii) 文件权限\n\n在下表中，您拥有可以使用所有者密码设置的文件权限。 用户密码用于打开文件。\n\n"
  in  "Text I1":string="“文档”调色板"
  in  "Texte J2 [ ]":T33=[{"Text"={"Text"="\n页眉、页脚和水印可以在创建报告期间的任何位置添加，因为它们在末尾写有“关闭 PDF.vi”。 为清楚起见，我们在创建新 PDF 报告后立即放置它们。\n\n页眉或页脚是一行最多三列等宽的表格。 添加到页眉或页脚（文本、图像或页码）的元素数量给出了表格的列数。\n\n页眉（或页脚）的总宽度是文本区域（页面宽度减去左边距和右边距）。 页眉（或页脚）的高度是页边距（顶部或底部）减去 10 毫米 (0.394\")。页眉或页脚垂直居中。", "Path"=path "", "Font complete"={"Name"="", "Size"=-1.0, "Color"=0, "Style"={"Bold"=FALSE, "Italic"=FALSE, "Underline"=FALSE, "Strikeout"=FALSE}, "Type"={"Type&direction"=enum."Select", "Embedded"=FALSE, "Encoding"=""}}}, "Link"={"Hyperlink"="", "Font complete"={"Name"="", "Size"=-1.0, "Color"=255, "Style"={"Bold"=FALSE, "Italic"=TRUE, "Underline"=FALSE, "Strikeout"=FALSE}, "Type"={"Type&direction"=enum."Select", "Embedded"=FALSE, "Encoding"=""}}}, "Paragraphe"={" Aligment"=enum."Select", "Line spacing"=enum."Select"}, "Indentation"={"Left"=0.0, "Right"=0.0}}]
  in  "Texte J4 [ ]":T33=[{"Text"={"Text"="标头", "Path"=path "", "Font complete"={"Name"="", "Size"=-1.0, "Color"=0, "Style"={"Bold"=TRUE, "Italic"=FALSE, "Underline"=FALSE, "Strikeout"=FALSE}, "Type"={"Type&direction"=enum."Select", "Embedded"=FALSE, "Encoding"=""}}}, "Link"={"Hyperlink"="", "Font complete"={"Name"="", "Size"=-1.0, "Color"=255, "Style"={"Bold"=FALSE, "Italic"=TRUE, "Underline"=FALSE, "Strikeout"=FALSE}, "Type"={"Type&direction"=enum."Select", "Embedded"=FALSE, "Encoding"=""}}}, "Paragraphe"={" Aligment"=enum."Select", "Line spacing"=enum."Select"}, "Indentation"={"Left"=0.0, "Right"=0.0}}, {"Text"={"Text"="\n在上图中，我们看到我们向标头添加了一个块。 因此，我们将有一个由单列组成的表。 如果我们查看控件“Header Text”，我们可以看到变量如下：\n    \n     - 首页;\n     - 文本（相关文本：LabVIEW 的 PDF 报告生成工具包...）；\n     - 链接（超链接可选 - http://itextpdf.com/）；\n     - 垂直和水平对齐（选择“CENTER-top”）；\n     - 字体（Arial，14 磅粗体）。\n\n此外，我们可以添加一条水平线将页眉或页脚与文本分开。\n\n", "Path"=path "", "Font complete"={"Name"="", "Size"=-1.0, "Color"=0, "Style"={"Bold"=FALSE, "Italic"=FALSE, "Underline"=FALSE, "Strikeout"=FALSE}, "Type"={"Type&direction"=enum."Select", "Embedded"=FALSE, "Encoding"=""}}}, "Link"={"Hyperlink"="", "Font complete"={"Name"="", "Size"=-1.0, "Color"=255, "Style"={"Bold"=FALSE, "Italic"=TRUE, "Underline"=FALSE, "Strikeout"=FALSE}, "Type"={"Type&direction"=enum."Select", "Embedded"=FALSE, "Encoding"=""}}}, "Paragraphe"={" Aligment"=enum."Select", "Line spacing"=enum."Select"}, "Indentation"={"Left"=0.0, "Right"=0.0}}]
  in  "Texte J5 [ ]":T33=[{"Text"={"Text"=" \n页脚Footer", "Path"=path "", "Font complete"={"Name"="", "Size"=-1.0, "Color"=0, "Style"={"Bold"=TRUE, "Italic"=FALSE, "Underline"=FALSE, "Strikeout"=FALSE}, "Type"={"Type&direction"=enum."Select", "Embedded"=FALSE, "Encoding"=""}}}, "Link"={"Hyperlink"="", "Font complete"={"Name"="", "Size"=-1.0, "Color"=255, "Style"={"Bold"=FALSE, "Italic"=TRUE, "Underline"=FALSE, "Strikeout"=FALSE}, "Type"={"Type&direction"=enum."Select", "Embedded"=FALSE, "Encoding"=""}}}, "Paragraphe"={" Aligment"=enum."Select", "Line spacing"=enum."Select"}, "Indentation"={"Left"=0.0, "Right"=0.0}}, {"Text"={"Text"="\n我们在页脚中添加了三个块。 因此，我们将有一个由三列组成的表。 块的添加是从左到右完成的：\n\n     - 第一个块，“文本”块位于左侧；\n     - 第二块，块“图像”位于中心；\n     - 最后一个块，“Page #”块位于右侧。\n\n在所有情况下，我们都需要指定此块在哪个页面开始出现（以及垂直和水平对齐方式）。 超链接始终是可选的。 如果图像太大而无法容纳提供的空间，则会自动缩小尺寸。\n\n", "Path"=path "", "Font complete"={"Name"="", "Size"=-1.0, "Color"=0, "Style"={"Bold"=FALSE, "Italic"=FALSE, "Underline"=FALSE, "Strikeout"=FALSE}, "Type"={"Type&direction"=enum."Select", "Embedded"=FALSE, "Encoding"=""}}}, "Link"={"Hyperlink"="", "Font complete"={"Name"="", "Size"=-1.0, "Color"=255, "Style"={"Bold"=FALSE, "Italic"=TRUE, "Underline"=FALSE, "Strikeout"=FALSE}, "Type"={"Type&direction"=enum."Select", "Embedded"=FALSE, "Encoding"=""}}}, "Paragraphe"={" Aligment"=enum."Select", "Line spacing"=enum."Select"}, "Indentation"={"Left"=0.0, "Right"=0.0}}]
  in  "Texte J6 [ ]":T33=[{"Text"={"Text"=" \n水印\n\n", "Path"=path "", "Font complete"={"Name"="", "Size"=-1.0, "Color"=0, "Style"={"Bold"=TRUE, "Italic"=FALSE, "Underline"=FALSE, "Strikeout"=FALSE}, "Type"={"Type&direction"=enum."Select", "Embedded"=FALSE, "Encoding"=""}}}, "Link"={"Hyperlink"="", "Font complete"={"Name"="", "Size"=-1.0, "Color"=255, "Style"={"Bold"=FALSE, "Italic"=TRUE, "Underline"=FALSE, "Strikeout"=FALSE}, "Type"={"Type&direction"=enum."Select", "Embedded"=FALSE, "Encoding"=""}}}, "Paragraphe"={" Aligment"=enum."Select", "Line spacing"=enum."Select"}, "Indentation"={"Left"=0.0, "Right"=0.0}}, {"Text"={"Text"="\n集群水印中的第一个元素是集群名称“General”，它包括：\n\n    - 类型（文本、文本自动和图像）；\n     - 不透明度 (%)；\n     - 旋转角度（旋转（？）\n     - 位置（绝对、页面中心和文本部分中心）；\n     - 绝对位置（X（毫米或英寸）和 Y（毫米或英寸））。\n\n\n该类型定义了我们添加的元素（文本、自动文本和图像）。 在“文本自动”的情况下，自动计算旋转角度，使文本位于区域（整个页面或文本区域）的对角线上，字体大小最大化。\n\n由于水印位于前景中，因此您必须指定其不透明度。 当您选择“文本”或“图片”时，我们可以指定文本框或图像的旋转。\n\n“绝对”位置仅适用于“文本”或“图片”类型。 选择此位置后，点 (0,0) 就是页面的左下角。\n\n\n", "Path"=path "", "Font complete"={"Name"="", "Size"=-1.0, "Color"=0, "Style"={"Bold"=FALSE, "Italic"=FALSE, "Underline"=FALSE, "Strikeout"=FALSE}, "Type"={"Type&direction"=enum."Select", "Embedded"=FALSE, "Encoding"=""}}}, "Link"={"Hyperlink"="", "Font complete"={"Name"="", "Size"=-1.0, "Color"=255, "Style"={"Bold"=FALSE, "Italic"=TRUE, "Underline"=FALSE, "Strikeout"=FALSE}, "Type"={"Type&direction"=enum."Select", "Embedded"=FALSE, "Encoding"=""}}}, "Paragraphe"={" Aligment"=enum."Select", "Line spacing"=enum."Select"}, "Indentation"={"Left"=0.0, "Right"=0.0}}]
  in  "Texte J3":string="\n\n页眉或页脚块使用“Header or Footer polymorphic.vi”添加，水印使用“Append Watermark.vi”添加。\n"
  in  "TexteJ7":string="\n对于水印，无法更改字体样式（粗体、斜体、下划线和删除线），并且 水印（Watermark） 仅支持 ASCII 字符。\n"
  in  "Text J1":string="The \"Header, Footer and Watermark\" palette"
  in  "Texte K2 [ ]":T33=[{"Text"={"Text"="\n\n您可以使用“将 PDF 文件附加到 PDF Report.vi”在 PDF 报告中附加 PDF 文件。 您必须注意报告是否有页眉或页脚，因为它是作为精确副本添加的（页脚和页眉可能会覆盖您添加的文本的一部分）。 该 VI 添加了本手册的最后一页。 我还包括一个独立的 VI 来连接 PDF 文件。\n\n", "Path"=path "", "Font complete"={"Name"="", "Size"=-1.0, "Color"=0, "Style"={"Bold"=FALSE, "Italic"=FALSE, "Underline"=FALSE, "Strikeout"=FALSE}, "Type"={"Type&direction"=enum."Select", "Embedded"=FALSE, "Encoding"=""}}}, "Link"={"Hyperlink"="", "Font complete"={"Name"="", "Size"=-1.0, "Color"=255, "Style"={"Bold"=FALSE, "Italic"=TRUE, "Underline"=FALSE, "Strikeout"=FALSE}, "Type"={"Type&direction"=enum."Select", "Embedded"=FALSE, "Encoding"=""}}}, "Paragraphe"={" Aligment"=enum."Select", "Line spacing"=enum."Select"}, "Indentation"={"Left"=0.0, "Right"=0.0}}]
  in  "Texte K3 [ ]":T33=[{"Text"={"Text"="使用的范围的一般语法如下所示：[!][o][odd][e][even]start-end。 您可以使用逗号分隔多个页面范围。 这 ！ 修饰符从已选择的页面中删除页面。 范围变化是递增的——数字在范围出现时被添加或删除。 开头或结尾可以省略。 如果两者都省略，则至少需要 o（奇数；选择所有奇数页）或 e（偶数；选择所有偶数页）：\n\n", "Path"=path "", "Font complete"={"Name"="", "Size"=-1.0, "Color"=0, "Style"={"Bold"=FALSE, "Italic"=FALSE, "Underline"=FALSE, "Strikeout"=FALSE}, "Type"={"Type&direction"=enum."Select", "Embedded"=FALSE, "Encoding"=""}}}, "Link"={"Hyperlink"="", "Font complete"={"Name"="", "Size"=-1.0, "Color"=255, "Style"={"Bold"=FALSE, "Italic"=TRUE, "Underline"=FALSE, "Strikeout"=FALSE}, "Type"={"Type&direction"=enum."Select", "Embedded"=FALSE, "Encoding"=""}}}, "Paragraphe"={" Aligment"=enum."Select", "Line spacing"=enum."Select"}, "Indentation"={"Left"=0.0, "Right"=0.0}}, {"Text"={"Text"="\"all\" : 完整的 PDF 文档\n“o”：选择所有奇数页\n“e”：选择所有偶数页\n“1-4、6-8、!7”：选择第 1、2、3、4、6 和 8 页（“！”排除第 7 页）\n\n", "Path"=path "", "Font complete"={"Name"="", "Size"=-1.0, "Color"=0, "Style"={"Bold"=FALSE, "Italic"=FALSE, "Underline"=FALSE, "Strikeout"=FALSE}, "Type"={"Type&direction"=enum."Select", "Embedded"=FALSE, "Encoding"=""}}}, "Link"={"Hyperlink"="", "Font complete"={"Name"="", "Size"=-1.0, "Color"=255, "Style"={"Bold"=FALSE, "Italic"=TRUE, "Underline"=FALSE, "Strikeout"=FALSE}, "Type"={"Type&direction"=enum."Select", "Embedded"=FALSE, "Encoding"=""}}}, "Paragraphe"={" Aligment"=enum."Select", "Line spacing"=enum."Select"}, "Indentation"={"Left"=1.0, "Right"=0.0}}, {"Text"={"Text"="如果 PDF 文件未受保护，则密码 = 空字符串。 如果 PDF 文件受保护，您需要提供：\n\n", "Path"=path "", "Font complete"={"Name"="", "Size"=-1.0, "Color"=0, "Style"={"Bold"=FALSE, "Italic"=FALSE, "Underline"=FALSE, "Strikeout"=FALSE}, "Type"={"Type&direction"=enum."Select", "Embedded"=FALSE, "Encoding"=""}}}, "Link"={"Hyperlink"="", "Font complete"={"Name"="", "Size"=-1.0, "Color"=255, "Style"={"Bold"=FALSE, "Italic"=TRUE, "Underline"=FALSE, "Strikeout"=FALSE}, "Type"={"Type&direction"=enum."Select", "Embedded"=FALSE, "Encoding"=""}}}, "Paragraphe"={" Aligment"=enum."Select", "Line spacing"=enum."Select"}, "Indentation"={"Left"=0.0, "Right"=0.0}}, {"Text"={"Text"="- 所有者密码（如果受用户和所有者密码保护）；\n- 所有者密码（如果仅使用所有者密码进行保护）；\n- 用户密码（如果仅使用用户密码进行保护）。\n", "Path"=path "", "Font complete"={"Name"="", "Size"=-1.0, "Color"=0, "Style"={"Bold"=FALSE, "Italic"=FALSE, "Underline"=FALSE, "Strikeout"=FALSE}, "Type"={"Type&direction"=enum."Select", "Embedded"=FALSE, "Encoding"=""}}}, "Link"={"Hyperlink"="", "Font complete"={"Name"="", "Size"=-1.0, "Color"=255, "Style"={"Bold"=FALSE, "Italic"=TRUE, "Underline"=FALSE, "Strikeout"=FALSE}, "Type"={"Type&direction"=enum."Select", "Embedded"=FALSE, "Encoding"=""}}}, "Paragraphe"={" Aligment"=enum."Select", "Line spacing"=enum."Select"}, "Indentation"={"Left"=1.0, "Right"=0.0}}]
  in  "Text k1":string="“连接”调色板"
  in  "Text L1":string="“目录”调色板"
  in  "Text L2":string="\n您可以添加自动编号书签 (Append Chapter bookmark.vi)，也可以添加目录 (Append a Table of Contents.vi)。\n"
  in  "Text L3":string="\n\nAppend Chapter bookmark.vi 使用 UTF-16 字符，就像您在本手册中看到的那样。\n"
  in  "Text L4":string="\n您还可以使用“Append a Table of Contents.vi”添加目录。 然后使用您设置的书签（使用“Append Chapter bookmark.vi”）生成目录。 如果您左键单击目录的文本，您将跳转到 ASCII 文本的相应部分，但不会跳转到 UTF-16 文本。\n"
  in  "Text M1":string="“工具”面板"
  in  "Text M2":string="这个调色板中的所有VIs都是独立的。\n\n前两个VIs(“读取Unicode文件。vi\"和\"Get Available Font Encoding [].vi\")将在下一节讨论。\n\n第三个VI“更改AcroField值(字符串)。vi\"允许更改PDF表单的AcroField(字符串)的值。\n\n第四VI“阅读AcroFields。vi\"允许读取PDF表单中的AcroFields列表。\n\n\n"
  in  "Texte N4 [ ]":T33=[{"Text"={"Text"="\n你可以访问字符U+0000到U+FFFF(在Windows的“字符映射”中是什么)。我知道两个方法来写Unicode文本在LabVIEW字符串:\n\n", "Path"=path "", "Font complete"={"Name"="", "Size"=-1.0, "Color"=0, "Style"={"Bold"=FALSE, "Italic"=FALSE, "Underline"=FALSE, "Strikeout"=FALSE}, "Type"={"Type&direction"=enum."Select", "Embedded"=FALSE, "Encoding"=""}}}, "Link"={"Hyperlink"="", "Font complete"={"Name"="", "Size"=-1.0, "Color"=255, "Style"={"Bold"=FALSE, "Italic"=TRUE, "Underline"=FALSE, "Strikeout"=FALSE}, "Type"={"Type&direction"=enum."Select", "Embedded"=FALSE, "Encoding"=""}}}, "Paragraphe"={" Aligment"=enum."Select", "Line spacing"=enum."Select"}, "Indentation"={"Left"=0.0, "Right"=0.0}}, {"Text"={"Text"="1) 通过在 LabVIEW.ini 中添加以下设置“UseUnicode=True”启用 Unicode 支持（参见“<a>在 LabVIEW 中使用 Unicode 的技巧和工具列表</a>”）并直接在字符串控件中写入 .\n2) 读取一个 Unicode 文本文件并将其复制到一个字符串中。", "Path"=path "", "Font complete"={"Name"="", "Size"=-1.0, "Color"=0, "Style"={"Bold"=FALSE, "Italic"=FALSE, "Underline"=FALSE, "Strikeout"=FALSE}, "Type"={"Type&direction"=enum."Select", "Embedded"=FALSE, "Encoding"=""}}}, "Link"={"Hyperlink"="https://decibel.ni.com/content/docs/DOC-10153", "Font complete"={"Name"="", "Size"=-1.0, "Color"=255, "Style"={"Bold"=FALSE, "Italic"=TRUE, "Underline"=FALSE, "Strikeout"=FALSE}, "Type"={"Type&direction"=enum."Select", "Embedded"=FALSE, "Encoding"=""}}}, "Paragraphe"={" Aligment"=enum."Select", "Line spacing"=enum."Select"}, "Indentation"={"Left"=0.75, "Right"=0.0}}, {"Text"={"Text"="\n我不再使用第一种方法，因为我经常遇到意外的 LabVIEW 崩溃或发生奇怪的事情（如 JackDunaway 在 <a>post 657</a> 中报告的）。 如果我想使用 Unicode，我会在记事本中编写文本，然后使用编码 Unicode 保存。\n", "Path"=path "", "Font complete"={"Name"="", "Size"=-1.0, "Color"=0, "Style"={"Bold"=FALSE, "Italic"=FALSE, "Underline"=FALSE, "Strikeout"=FALSE}, "Type"={"Type&direction"=enum."Select", "Embedded"=FALSE, "Encoding"=""}}}, "Link"={"Hyperlink"="http://forums.ni.com/t5/BreakPoint/Rube-Goldberg-Code/m-p/1106596#M11877", "Font complete"={"Name"="", "Size"=-1.0, "Color"=255, "Style"={"Bold"=FALSE, "Italic"=TRUE, "Underline"=FALSE, "Strikeout"=FALSE}, "Type"={"Type&direction"=enum."Select", "Embedded"=FALSE, "Encoding"=""}}}, "Paragraphe"={" Aligment"=enum."Select", "Line spacing"=enum."Select"}, "Indentation"={"Left"=0.0, "Right"=0.0}}]
  in  "Text N1":string="U\u0000n\u0000i\u0000c\u0000o\u0000d\u0000e\u0000 \u0000U\u0000T\u0000F\u0000-\u00001\u00006\u0000 \u0000(\u0000B\u0000a\u0000s\u0000i\u0000c\u0000 \u0000M\u0000u\u0000l\u0000t\u0000i\u0000l\u0000i\u0000n\u0000g\u0000u\u0000a\u0000l\u0000 \u0000P\u0000l\u0000a\u0000n\u0000e\u0000)\u0000 \u0000i\u0000n\u0000 \u0000P\u0000D\u0000F\u0000 \u0000R\u0000e\u0000p\u0000o\u0000r\u0000t\u0000 \u0000(\u0000.\u0004=\u00048\u0004:\u0004>\u00044\u0004)\u0000"
  in  "Font N1":T11={"Name"="Arial Unicode MS", "Size"=-1.0, "Color"=0, "Style"={"Bold"=TRUE, "Italic"=FALSE, "Underline"=FALSE, "Strikeout"=FALSE}, "Type"={"Type&direction"=enum."UTF-16", "Embedded"=FALSE, "Encoding"="CP1251"}}
  in  "Text N10":string="\n如果您想知道字体支持的不同编码，可以使用“Get Available font encoding[]”。Vi”(您至少需要知道一种受支持的编码)。\n\n"
  in  "Text N8":string="\n以下是PDF报告中的字符串，字体= \"Arial Unicode MS\"，粗体= True，编码= CP1251(西里尔字母)和类型= Unicode:\n"
  in  "Text N6":string="这是保存在记事本(作为Unicode)的原始文本。\n"
  in  "Text N5":string="然后我用“读取Unicode文件”读取文件。vi\"(在工具面板)和我复制文本从“复制从这个字符串”在PDF报告的字符串。\n\n因为我们没有启用Unicode支持，而且我们不想激活这种支持，那么您在正常显示中看到的显示是不正确的，但字符串中的六边形值是正确的。"
  in  "Text N9":string
  in  "Text N7":string="\n以下是PDF报告字符串中复制的文本。\n"
  in  "Text N3":string="如何写Unicode文本在一个字符串"
  in  "Text N11":string="哪个VIs支持Unicode"
  in  "Text N2":string="\n警告:LabVIEW官方不支持Unicode。\n\n"
  in  "Text O2 [ ]":T33=[{"Text"={"Text"="\n\n\nError 1172\n\n", "Path"=path "", "Font complete"={"Name"="", "Size"=-1.0, "Color"=0, "Style"={"Bold"=TRUE, "Italic"=FALSE, "Underline"=FALSE, "Strikeout"=FALSE}, "Type"={"Type&direction"=enum."Select", "Embedded"=FALSE, "Encoding"=""}}}, "Link"={"Hyperlink"="", "Font complete"={"Name"="", "Size"=-1.0, "Color"=255, "Style"={"Bold"=FALSE, "Italic"=TRUE, "Underline"=FALSE, "Strikeout"=FALSE}, "Type"={"Type&direction"=enum."Select", "Embedded"=FALSE, "Encoding"=""}}}, "Paragraphe"={" Aligment"=enum."Select", "Line spacing"=enum."Select"}, "Indentation"={"Left"=0.0, "Right"=0.0}}, {"Text"={"Text"="如果构建的应用程序在网络驱动器上运行，请查看:<a>运行LabVIEW VIs或从网络驱动器使用。net程序集的可执行文件</a>这段文字在手册的下一页。", "Path"=path "", "Font complete"={"Name"="", "Size"=-1.0, "Color"=0, "Style"={"Bold"=FALSE, "Italic"=FALSE, "Underline"=FALSE, "Strikeout"=FALSE}, "Type"={"Type&direction"=enum."Select", "Embedded"=FALSE, "Encoding"=""}}}, "Link"={"Hyperlink"="http://digital.ni.com/public.nsf/allkb/F326A891E72073B486256EEC0006E019", "Font complete"={"Name"="", "Size"=-1.0, "Color"=255, "Style"={"Bold"=FALSE, "Italic"=TRUE, "Underline"=FALSE, "Strikeout"=FALSE}, "Type"={"Type&direction"=enum."Select", "Embedded"=FALSE, "Encoding"=""}}}, "Paragraphe"={" Aligment"=enum."Select", "Line spacing"=enum."Select"}, "Indentation"={"Left"=0.0, "Right"=0.0}}, {"Text"={"Text"="\n\n\n对于构建的应用程序：\n\n", "Path"=path "", "Font complete"={"Name"="", "Size"=-1.0, "Color"=0, "Style"={"Bold"=TRUE, "Italic"=FALSE, "Underline"=FALSE, "Strikeout"=FALSE}, "Type"={"Type&direction"=enum."Select", "Embedded"=FALSE, "Encoding"=""}}}, "Link"={"Hyperlink"="", "Font complete"={"Name"="", "Size"=-1.0, "Color"=255, "Style"={"Bold"=FALSE, "Italic"=TRUE, "Underline"=FALSE, "Strikeout"=FALSE}, "Type"={"Type&direction"=enum."Select", "Embedded"=FALSE, "Encoding"=""}}}, "Paragraphe"={" Aligment"=enum."Select", "Line spacing"=enum."Select"}, "Indentation"={"Left"=0.0, "Right"=0.0}}, {"Text"={"Text"="“Properties>>Source Files>>Always included” add “itextsharp.dll”\n\niTextSharp.dll Î»ÓÚ£º\n\nC:\\Program Files\\National Instruments\\LabVIEW XXXX\\vi.lib\\Exaprom PDF\\DLL\\itextsharp.dll", "Path"=path "", "Font complete"={"Name"="", "Size"=-1.0, "Color"=0, "Style"={"Bold"=FALSE, "Italic"=FALSE, "Underline"=FALSE, "Strikeout"=FALSE}, "Type"={"Type&direction"=enum."Select", "Embedded"=FALSE, "Encoding"=""}}}, "Link"={"Hyperlink"="", "Font complete"={"Name"="", "Size"=-1.0, "Color"=255, "Style"={"Bold"=FALSE, "Italic"=TRUE, "Underline"=FALSE, "Strikeout"=FALSE}, "Type"={"Type&direction"=enum."Select", "Embedded"=FALSE, "Encoding"=""}}}, "Paragraphe"={" Aligment"=enum."LEFT", "Line spacing"=enum."Select"}, "Indentation"={"Left"=0.0, "Right"=0.0}}]
  in  "PDF Files  to concatenate and pages":T36={"Path"=path "C:/Program Files (x86)/National Instruments/LabVIEW 2020/user.lib/labview-PDF-writer-master/Examples/Images/Running LabVIEW VIs or Executables That Use .NET Assemblies From a Network Drive.pdf", "Pages"="all", "Password"=""}
  in  "Text O1":string="编译应用程序时出错1172"
  in  "Image F4":cluster{"Nom":path, "Légende":string}={"Nom"=path "C:/Program Files/National Instruments/LabVIEW 2009/vi.lib/Exaprom PDF/Examples/Images/Palette Text/Palette Text.jpg", "Légende"="Text palette and the VI \"Append Text polymorphic.vi\""}
  in  "Image H8":cluster{"Nom":path, "Légende":string}={"Nom"=path "C:/Program Files/National Instruments/LabVIEW 2009/vi.lib/Exaprom PDF/Examples/Images/Palette Table/Custom Borders.jpg", "Légende"="Custom borders"}
  in  "Image C2":cluster{"Nom":path, "Légende":string}={"Nom"=path "C:/Program Files/National Instruments/LabVIEW 2009/vi.lib/Exaprom PDF/Examples/Images/Installation/Folder programming.jpg", "Légende"="Folder \"Exaprom PDF\""}
  in  "Image F5":cluster{"Nom":path, "Légende":string}={"Nom"=path "C:/Program Files/National Instruments/LabVIEW 2009/vi.lib/Exaprom PDF/Examples/Images/Palette Text/Controls Text poly.jpg", "Légende"="The main variables for the different VIs of \"Append Text polymorphic.vi\""}
  in  "Image G1":cluster{"Nom":path, "Légende":string}={"Nom"=path "C:/Program Files/National Instruments/LabVIEW 2009/vi.lib/Exaprom PDF/Examples/Images/Palette Images/Palette Image.jpg", "Légende"="The VIs to insert images in PDF documents (this image was\nadded with \"Append Image.vi\")"}
  in  "Image H1":cluster{"Nom":path, "Légende":string}={"Nom"=path "C:/Program Files/National Instruments/LabVIEW 2009/vi.lib/Exaprom PDF/Examples/Images/Palette Table/Palette Table.jpg", "Légende"="The three VIs to create a table"}
  in  "Image H2":cluster{"Nom":path, "Légende":string}={"Nom"=path "C:/Program Files/National Instruments/LabVIEW 2009/vi.lib/Exaprom PDF/Examples/Images/Palette Table/Create table B.jpg", "Légende"="Table creation"}
  in  "Image H3":cluster{"Nom":path, "Légende":string}={"Nom"=path "C:/Program Files/National Instruments/LabVIEW 2009/vi.lib/Exaprom PDF/Examples/Images/Palette Table/Create Table VI.jpg", "Légende"="Create Table.vi and default values"}
  in  "Image D1":cluster{"Nom":path, "Légende":string}={"Nom"=path "C:/Program Files/National Instruments/LabVIEW 2009/vi.lib/Exaprom PDF/Examples/Images/Simplified Report block diagram V2.jpg", "Légende"="\"Bloc Diagram\" of a simplified PDF Report"}
  in  "Image E1":cluster{"Nom":path, "Légende":string}={"Nom"=path "C:/Program Files/National Instruments/LabVIEW 2009/vi.lib/Exaprom PDF/Examples/Images/Page Layout V2.jpg", "Légende"="Text zone and origin"}
  in  "Image G2":string="Font Panel Image (this image was added with  \"Append Front Panel Image.vi\")"
  in  "Image H6":cluster{"Nom":path, "Légende":string}={"Nom"=path "C:/Program Files/National Instruments/LabVIEW 2009/vi.lib/Exaprom PDF/Examples/Images/Palette Table/Predefined borders.jpg", "Légende"="Choice of table borders (the default is framed)."}
  in  "Image H5":cluster{"Nom":path, "Légende":string}={"Nom"=path "C:/Program Files/National Instruments/LabVIEW 2009/vi.lib/Exaprom PDF/Examples/Images/Palette Table/Append Table VI.jpg", "Légende"="Append Table.vi and default values"}
  in  "Image G3":string="Block Diagram Image (this image was added with \"Append Block Diagram Image.vi\")"
  in  "Add block diagram":bool=TRUE caption="Add block \ndiagram image"
  in  "Image C3":cluster{"Nom":path, "Légende":string}={"Nom"=path "C:/Program Files/National Instruments/LabVIEW 2009/vi.lib/Exaprom PDF/Examples/Images/Installation/Folder menu.jpg", "Légende"="File \"exaprompdf.mnu\""}
  in  "Image C4":cluster{"Nom":path, "Légende":string}={"Nom"=path "C:/Program Files/National Instruments/LabVIEW 2009/vi.lib/Exaprom PDF/Examples/Images/Installation/Palette Exaprom.jpg", "Légende"="Palette \"PDF Exaprom\""}
  in  "Image F2":cluster{"Nom":path, "Légende":string}={"Nom"=path "C:/Program Files/National Instruments/LabVIEW 2009/vi.lib/Exaprom PDF/Examples/Images/Palette Text/Controls Text Types.jpg", "Légende"="Text Types (ASCII or Unicode) and writing directions"}
  in  "Image H7":cluster{"Nom":path, "Légende":string}={"Nom"=path "C:/Program Files/National Instruments/LabVIEW 2009/vi.lib/Exaprom PDF/Examples/Images/Palette Table/Table Standard Format.jpg", "Légende"="Cell format for the column headers, the row headers and the data "}
  in  "Image H9":cluster{"Nom":path, "Légende":string}={"Nom"=path "C:/Program Files/National Instruments/LabVIEW 2009/vi.lib/Exaprom PDF/Examples/Images/Palette Table/Append Customized VI.jpg", "Légende"="Append Customized Table.vi and default values"}
  in  "Image H10":cluster{"Nom":path, "Légende":string}={"Nom"=path "C:/Program Files/National Instruments/LabVIEW 2009/vi.lib/Exaprom PDF/Examples/Images/Palette Table/Control for Append Customized Table VI.jpg", "Légende"="Specific control for \"Append Customized Table.vi\" at the right bottom"}
  in  "Cluster of images controls":T40={"Scale (%)"=55.0, "Position"={"Alignment"=enum."Left (textwrap)", "X "=0.0, "Y"=0.0, "Indentation"=0.1}, "Border"={"Show?"=TRUE, "Thickness (point)"=5.0, "Color"=3418879}}
  in  "Image H11":cluster{"Nom":path, "Légende":string}={"Nom"=path "C:/Program Files/National Instruments/LabVIEW 2009/vi.lib/Exaprom PDF/Examples/Images/Palette Table/Block Diagram Tableaux 2 et 3.jpg", "Légende"="Block diagram for table 2 and 3"}
  in  "Image H12":cluster{"Nom":path, "Légende":string}={"Nom"=path "C:/Program Files/National Instruments/LabVIEW 2009/vi.lib/Exaprom PDF/Examples/Images/Palette Table/Block Diagram Tableau 4.jpg", "Légende"="Block diagram for table 4"}
  in  "Image H13":cluster{"Nom":path, "Légende":string}={"Nom"=path "C:/Program Files/National Instruments/LabVIEW 2009/vi.lib/Exaprom PDF/Examples/Images/Palette Table/Block Diagram Tableau 5.jpg", "Légende"="Block diagram for table 5"}
  in  "Image C1":cluster{"Nom":path, "Légende":string}={"Nom"=path "C:/Program Files/National Instruments/LabVIEW 2009/vi.lib/Exaprom PDF/Examples/Images/Installation/Unzip ExapromPDF 2.jpg", "Légende"="Folder \"Exaprom PD2.0\" unzipped"}
  in  "Image F3":cluster{"Nom":path, "Légende":string}={"Nom"=path "C:/Program Files/National Instruments/LabVIEW 2009/vi.lib/Exaprom PDF/Examples/Images/Palette Text/Default Paragraph.jpg", "Légende"="Alignment and line spacing"}
  in  "Image F1":cluster{"Nom":path, "Légende":string}={"Nom"=path "C:/Program Files/National Instruments/LabVIEW 2009/vi.lib/Exaprom PDF/Examples/Images/Palette Text/Font V and H clusters.jpg", "Légende"="Vertical and horizontal cluster font"}
  in  "Image H4":cluster{"Nom":path, "Légende":string}={"Nom"=path "C:/Program Files/National Instruments/LabVIEW 2009/vi.lib/Exaprom PDF/Examples/Images/Palette Table/Final table.jpg", "Légende"="Final table generated"}
  in  "Image L1":cluster{"Nom":path, "Légende":string}={"Nom"=path "C:/Program Files/National Instruments/LabVIEW 2009/vi.lib/Exaprom PDF/Examples/Images/TOC Palette/TOC palette.jpg", "Légende"="VIs of \"Table of Contents\" palette"}
  in  "Image J10":string="Text Watermark control"
  in  "Image J9":string="Image Watermark control"
  in  "Image J4":cluster{"Nom":path, "Légende":string}={"Nom"=path "C:/Program Files/National Instruments/LabVIEW 2009/vi.lib/Exaprom PDF/Examples/Images/Palette Header Footer Watermark/Header2.jpg", "Légende"="Horizontal line and block Text of the Header"}
  in  "Image J3":cluster{"Nom":path, "Légende":string}={"Nom"=path "C:/Program Files/National Instruments/LabVIEW 2009/vi.lib/Exaprom PDF/Examples/Images/Palette Header Footer Watermark/Block Diagram H F and W.jpg", "Légende"="Block Diagram for Header, Footer and Watermark"}
  in  "Image J2":cluster{"Nom":path, "Légende":string}={"Nom"=path "C:/Program Files/National Instruments/LabVIEW 2009/vi.lib/Exaprom PDF/Examples/Images/Palette Header Footer Watermark/Palette Header, Footer et Watermark.jpg", "Légende"="Header, Footer and Watermark palette"}
  in  "Image J1":cluster{"Nom":path, "Légende":string}={"Nom"=path "C:/Program Files/National Instruments/LabVIEW 2009/vi.lib/Exaprom PDF/Examples/Images/Palette Header Footer Watermark/Header footer V2.jpg", "Légende"="Header and footer"}
  in  "Image I2":cluster{"Nom":path, "Légende":string}={"Nom"=path "C:/Program Files/National Instruments/LabVIEW 2009/vi.lib/Exaprom PDF/Examples/Images/Palette Document/New PDF VI variables.jpg", "Légende"="Variables for a new PDF report"}
  in  "Image I3":cluster{"Nom":path, "Légende":string}={"Nom"=path "C:/Program Files/National Instruments/LabVIEW 2009/vi.lib/Exaprom PDF/Examples/Images/Palette Document/New PDF VI.jpg", "Légende"="New PDF.vi and his default values"}
  in  "Image I4":cluster{"Nom":path, "Légende":string}={"Nom"=path "C:/Program Files/National Instruments/LabVIEW 2009/vi.lib/Exaprom PDF/Examples/Images/Palette Document/Metadatas.jpg", "Légende"="Metada (PDF Details)"}
  in  "Image I1":cluster{"Nom":path, "Légende":string}={"Nom"=path "C:/Program Files/National Instruments/LabVIEW 2009/vi.lib/Exaprom PDF/Examples/Images/Palette Document/Palette Document.jpg", "Légende"="VIs of \"Document\" palette"}
  in  "Image J5":cluster{"Nom":path, "Légende":string}={"Nom"=path "C:/Program Files/National Instruments/LabVIEW 2009/vi.lib/Exaprom PDF/Examples/Images/Palette Header Footer Watermark/Footer Text.jpg", "Légende"="Footer Text block"}
  in  "Image J6":cluster{"Nom":path, "Légende":string}={"Nom"=path "C:/Program Files/National Instruments/LabVIEW 2009/vi.lib/Exaprom PDF/Examples/Images/Palette Header Footer Watermark/Footer Image.jpg", "Légende"="Footer Image block"}
  in  "Image J7":cluster{"Nom":path, "Légende":string}={"Nom"=path "C:/Program Files/National Instruments/LabVIEW 2009/vi.lib/Exaprom PDF/Examples/Images/Palette Header Footer Watermark/Footer Page#.jpg", "Légende"="Footer Page number block"}
  in  "Image J8":cluster{"Nom":path, "Légende":string}={"Nom"=path "C:/Program Files/National Instruments/LabVIEW 2009/vi.lib/Exaprom PDF/Examples/Images/Palette Header Footer Watermark/Two footers.jpg", "Légende"="Change the order of VIs"}
  in  "Image K1":cluster{"Nom":path, "Légende":string}={"Nom"=path "C:/Program Files/National Instruments/LabVIEW 2009/vi.lib/Exaprom PDF/Examples/Images/Palette Concatenate/Palette Concatenate.jpg", "Légende"="VIs of \"Concatenate\" palette"}
  in  "Image N1":cluster{"Nom":path, "Légende":string}={"Nom"=path "C:/Program Files/National Instruments/LabVIEW 2009/vi.lib/Exaprom PDF/Examples/Images/Unicode/Cyrillic 0410 to 042F.jpg", "Légende"="Notepad and Unicode"}
  in  "Image N2":cluster{"Nom":path, "Légende":string}={"Nom"=path "C:/Program Files/National Instruments/LabVIEW 2009/vi.lib/Exaprom PDF/Examples/Images/Unicode/Read Unicode File VI.jpg", "Légende"="Copy the text from \"Read Unicode File.vi\" and paste in  the string of the PDF Report"}
  in  "Image N3":cluster{"Nom":path, "Légende":string}={"Nom"=path "C:/Program Files/National Instruments/LabVIEW 2009/vi.lib/Exaprom PDF/Examples/Images/Unicode/Unicode string in Notepad.jpg", "Légende"="Original text in Notepad"}
  in  "Image N4":string="String in the PDF Report (not shown correctly, but the hexagonal values from the string are correct)"
  in  "Image N5":cluster{"Nom":path, "Légende":string}={"Nom"=path "C:/Program Files/National Instruments/LabVIEW 2009/vi.lib/Exaprom PDF/Examples/Images/Unicode/Get Available Font Encoding VI.jpg", "Légende"="Get Availaible Font Encoding [ ].vi for \"Arial Unicode MS\" (ARIALUNI.TTF)"}
  in  "Image K2":string="Variable of \"Append PDF file to PDF Report .vi\""
  in  "Image M1":cluster{"Nom":path, "Légende":string}={"Nom"=path "C:/Program Files/National Instruments/LabVIEW 2009/vi.lib/Exaprom PDF/Examples/Images/Tools palette/Tools palette.jpg", "Légende"="VIs of \"Tools\" palette"}
  in  "Image L2":cluster{"Nom":path, "Légende":string}={"Nom"=path "C:/Program Files/National Instruments/LabVIEW 2009/vi.lib/Exaprom PDF/Examples/Images/TOC Palette/Append Bookmark VI.jpg", "Légende"="Append Chapter bookmark.vi"}
  in  "Image L3":cluster{"Nom":path, "Légende":string}={"Nom"=path "C:/Program Files/National Instruments/LabVIEW 2009/vi.lib/Exaprom PDF/Examples/Images/TOC Palette/User Manual Bookmark.jpg", "Légende"="Bookmarks ot this User Manual"}
  in  "Image L4":cluster{"Nom":path, "Légende":string}={"Nom"=path "C:/Program Files/National Instruments/LabVIEW 2009/vi.lib/Exaprom PDF/Examples/Images/TOC Palette/Append TOC VI.jpg", "Légende"="Append a Table of Contents.vi"}
  in  "Predefined Borders Table 1":T41={"Borders"=4, "Header"={"Thickness"=1.0, "Line"=0, "Background "=16777215}, "Data"={"Thickness"=0.5, "Line"=0, "Background "=16777215}}
  in  "Image to Add [ ]":T44(array[cluster])=[{"Image name"="Arrow", "Path"=path "C:/Program Files/National Instruments/LabVIEW 2009/vi.lib/Exaprom PDF/Examples/Images/Arrow.jpg", "Scale"=7.0}, {"Image name"="Default", "Path"=path "C:/Program Files/National Instruments/LabVIEW 2009/vi.lib/Exaprom PDF/Examples/Images/Palette Text/Default font.jpg", "Scale"=100.0}, {"Image name"="A", "Path"=path "C:/Program Files/National Instruments/LabVIEW 2009/vi.lib/Exaprom PDF/Examples/Images/Palette Text/Font A.jpg", "Scale"=100.0}, {"Image name"="B", "Path"=path "C:/Program Files/National Instruments/LabVIEW 2009/vi.lib/Exaprom PDF/Examples/Images/Palette Text/Font B.jpg", "Scale"=100.0}, {"Image name"="B1", "Path"=path "C:/Program Files/National Instruments/LabVIEW 2009/vi.lib/Exaprom PDF/Examples/Images/Palette Text/Font B1.jpg", "Scale"=100.0}, {"Image name"="C", "Path"=path "C:/Program Files/National Instruments/LabVIEW 2009/vi.lib/Exaprom PDF/Examples/Images/Palette Text/Font C.jpg", "Scale"=100.0}, {"Image name"="C1", "Path"=path "C:/Program Files/National Instruments/LabVIEW 2009/vi.lib/Exaprom PDF/Examples/Images/Palette Text/Font C1.jpg", "Scale"=100.0}, {"Image name"="D", "Path"=path "C:/Program Files/National Instruments/LabVIEW 2009/vi.lib/Exaprom PDF/Examples/Images/Palette Text/Font D.jpg", "Scale"=100.0}, {"Image name"="D1", "Path"=path "C:/Program Files/National Instruments/LabVIEW 2009/vi.lib/Exaprom PDF/Examples/Images/Palette Text/Font D1.jpg", "Scale"=100.0}, {"Image name"="E", "Path"=path "C:/Program Files/National Instruments/LabVIEW 2009/vi.lib/Exaprom PDF/Examples/Images/Palette Text/Font E.jpg", "Scale"=100.0}, {"Image name"="E1", "Path"=path "C:/Program Files/National Instruments/LabVIEW 2009/vi.lib/Exaprom PDF/Examples/Images/Palette Text/Font E1.jpg", "Scale"=100.0}, {"Image name"="Logo", "Path"=path "C:/Program Files/National Instruments/LabVIEW 2009/vi.lib/Exaprom PDF/Examples/Images/Logo Exaprom.jpg", "Scale"=15.0}, {"Image name"="Row1", "Path"=path "C:/Program Files/National Instruments/LabVIEW 2009/vi.lib/Exaprom PDF/Examples/Images/Palette Table/Row1.jpg", "Scale"=37.0}, {"Image name"="Row2", "Path"=path "C:/Program Files/National Instruments/LabVIEW 2009/vi.lib/Exaprom PDF/Examples/Images/Palette Table/Row2.jpg", "Scale"=37.0}, {"Image name"="Row3", "Path"=path "C:/Program Files/National Instruments/LabVIEW 2009/vi.lib/Exaprom PDF/Examples/Images/Palette Table/Row3.jpg", "Scale"=37.0}] {"Scale" format="%#_g %"}
  in  "Caption 1":string="如果“默认字体”是Arial 12点(粗体，下划线，斜体和删除线= false)，类型和方向= ASCII，嵌入式= F和编码= CP1252。"
  in  "Datas properties 1":T45={"Cell Type, Alignment and LS"={"Cell Alignment"=5, "Text rotation"=enum."None", "Line spacing"=enum."Select"}, "Font"={"Name"="", "Size"=0.0, "Color"=0, "Style"={"Bold"=FALSE, "Italic"=FALSE, "Underline"=FALSE, "Strikeout"=FALSE}, "Type"={"Type&direction"=enum."Select", "Embedded"=FALSE, "Encoding"=""}}}
  in  "Column Headers 2D [ ] - Table 1":string[][](array[string])=[["Wired to terminal", "", "在\nPDF报告", " ", "Wired to terminal", " ", "In the\nPDF Report"]]
  in  "Table columnWidth [ ] - Table 1":sgl[](array[numeric])=[1.0, 0.6, 1.0, 0.4, 1.0, 0.6, 1.0]
  in  "Table properties 1)":T48={"Table position"=1, "SpacingBefore (points)"=12.0, "SpacingAfter (points)"=12.0} {"Table position" items=["LEFT", "CENTER", "RIGHT"]}
  in  "Text Data 2D [ ] - Table 1":string[][](array[string])=[["nothing", "Arrow", "Default", "", "C", "Arrow", "C1"], ["A", "Arrow", "Default", "", "D", "Arrow", "D1"], ["B", "Arrow", "B1", "", "E", "Arrow", "E1"]]
  in  "Custom Table Borders 1":T50=[{"Row"={"#"=0, "to #"=0}, "Line"={"Thickness"=1.5, "Color"=0}, "Column Borders [ ]"=[{"Cell Border"=8, "BG"=16776704}, {"Cell Border"=4, "BG"=16776704}, {"Cell Border"=18, "BG"=16776704}, {"Cell Border"=0, "BG"=16777225}, {"Cell Border"=8, "BG"=16776704}, {"Cell Border"=4, "BG"=16776704}, {"Cell Border"=18, "BG"=16776704}]}, {"Row"={"#"=1, "to #"=-1}, "Line"={"Thickness"=0.75, "Color"=0}, "Column Borders [ ]"=[{"Cell Border"=2, "BG"=16777225}, {"Cell Border"=1, "BG"=16777225}, {"Cell Border"=17, "BG"=16777225}, {"Cell Border"=0, "BG"=16777225}, {"Cell Border"=2, "BG"=16777225}, {"Cell Border"=1, "BG"=16777225}, {"Cell Border"=17, "BG"=16777225}]}]
  in  "Table columnWidth [ ]  - Tables 3 and 4":sgl[](array[numeric])=[1.0, 1.4, 1.4, 1.4]
  in  "Column Headers 2D [ ] - Tables 2 to 4":string[][](array[string])=[["Time", "热电偶 1(℃)", "热电偶 2(℃)", "热电偶 3(℃)"]]
  in  "Text Data 2D [ ]  - Tables 2 to 4":string[][](array[string])=[["09:59:42", "214.8", "212.3", "216.1"], ["09:59:52", "215.0", "212.4", "217.8"], ["10:00:02", "215.0", "212.0", "217.7"], ["10:00:12", "214.1", "211.6", "217.2"], ["10:00:22", "214.2", "212.6", "217.3"], ["10:00:32", "214.6", "212.5", "217.8"], ["10:00:42", "214.6", "212.5", "217.8"], ["10:00:52", "214.8", "212.5", "216.3"], ["10:01:02", "215.6", "211.7", "216.7"], ["10:01:12", "214.6", "211.1", "218.0"]]
  in  "Table properties  - Tables 2 to 4":T48={"Table position"=1, "SpacingBefore (points)"=12.0, "SpacingAfter (points)"=12.0} {"Table position" items=["LEFT", "CENTER", "RIGHT"]}
  in  "Caption - Table 2":string="变量columnWidth[] \"未连接的表示例"
  in  "Caption - Table 3":string="使用变量columnWidth[] \"连线的表的示例"
  in  "Caption - Table 4":string="示例行背景颜色"
  in  "Row background color - Table 4":T55={"color"=14606046, "at each"=3}
  in  "Predefined Borders - Table 4":T41={"Borders"=2, "Header"={"Thickness"=1.0, "Line"=0, "Background "=15990711}, "Data"={"Thickness"=0.5, "Line"=0, "Background "=16777215}}
  in  "Datas format - Table 4":T45={"Cell Type, Alignment and LS"={"Cell Alignment"=5, "Text rotation"=enum."None", "Line spacing"=enum."Select"}, "Font"={"Name"="", "Size"=0.0, "Color"=0, "Style"={"Bold"=FALSE, "Italic"=FALSE, "Underline"=FALSE, "Strikeout"=FALSE}, "Type"={"Type&direction"=enum."Select", "Embedded"=FALSE, "Encoding"=""}}}
  in  "Column Header format - Table 4":T45={"Cell Type, Alignment and LS"={"Cell Alignment"=5, "Text rotation"=enum."None", "Line spacing"=enum."Select"}, "Font"={"Name"="", "Size"=0.0, "Color"=0, "Style"={"Bold"=FALSE, "Italic"=FALSE, "Underline"=FALSE, "Strikeout"=FALSE}, "Type"={"Type&direction"=enum."Select", "Embedded"=FALSE, "Encoding"=""}}}
  in  "Table columnWidth [ ] - Table 5":sgl[](array[numeric])=[0.75, 0.6, 0.6, 0.6, 0.6, 0.6, 0.6]
  in  "Column Headers 2D [ ] - Table 5":string[][](array[string])=[["", "熔炉 (℃)", "", "", "坩埚(℃)", "", ""], ["", "热电偶 1", "热电偶  2", "热电偶  3", "热电偶  4", "热电偶 5", "热电偶  6"]]
  in  "Text Data 2D [ ] - Table 5":string[][](array[string])=[["722.2", "753.0", "714.6", "647.7", "649.3", "644.9"], ["722.9", "751.2", "711.4", "646.4", "652.7", "646.9"], ["721.8", "753.0", "713.0", "645.3", "652.5", "645.4"], ["724.2", "750.9", "711.6", "648.9", "651.1", "644.0"], ["723.7", "752.4", "710.7", "648.4", "650.6", "645.3"], ["723.9", "753.8", "712.2", "645.3", "648.9", "646.8"], ["722.6", "754.1", "710.5", "645.7", "651.0", "645.8"], ["724.6", "751.2", "713.8", "648.8", "648.6", "644.4"], ["722.9", "750.7", "710.8", "645.7", "649.7", "647.2"], ["721.8", "755.0", "713.7", "646.8", "652.2", "644.5"], ["723.1", "752.5", "712.2", "646.9", "650.7", "645.5"]]
  in  "Table properties - Table 5":T48={"Table position"=1, "SpacingBefore (points)"=12.0, "SpacingAfter (points)"=12.0} {"Table position" items=["LEFT", "CENTER", "RIGHT"]}
  in  "Caption - Table 5":string="合并单元格示例"
  in  "Row Headers 1D [ ] - Table 5":string[](array[string])=["Test 1", "Test 2", "Test 3", "Test 4", "Test 5", "Test 6", "Test 7", "Test 8", "Test 9", "Test 10", "Mean"]
  in  "Row  [ ] - Table 5":T56=[{"Row"={"From #"=0, "to #"=0}, "Cell [ ]"=[{"Text"={"Cell Alignment"=5, "Text rotation"=enum."None", "Line spacing"=enum."Select"}, "Cell Appearance"={"Border"=0, "Thickness"=0.5, "Color"=0, "BG"=16777225}, "HMerge"={"From"=-1, "to"=-1}, "VMerge"={"From"=-1, "to"=-1}, "Font"={"Name"="Arial", "Size"=-1.0, "Color"=0, "Style"={"Bold"=FALSE, "Italic"=FALSE, "Underline"=FALSE, "Strikeout"=FALSE}, "Type"={"Type&direction"=enum."ASCII", "Embedded"=FALSE, "Encoding"=""}}}, {"Text"={"Cell Alignment"=5, "Text rotation"=enum."None", "Line spacing"=enum."Select"}, "Cell Appearance"={"Border"=8, "Thickness"=1.0, "Color"=0, "BG"=16777225}, "HMerge"={"From"=1, "to"=3}, "VMerge"={"From"=-1, "to"=-1}, "Font"={"Name"="Arial", "Size"=0.0, "Color"=0, "Style"={"Bold"=TRUE, "Italic"=FALSE, "Underline"=FALSE, "Strikeout"=FALSE}, "Type"={"Type&direction"=enum."ASCII", "Embedded"=FALSE, "Encoding"=""}}}, {"Text"={"Cell Alignment"=5, "Text rotation"=enum."None", "Line spacing"=enum."Select"}, "Cell Appearance"={"Border"=5, "Thickness"=1.0, "Color"=0, "BG"=16777225}, "HMerge"={"From"=4, "to"=6}, "VMerge"={"From"=-1, "to"=-1}, "Font"={"Name"="Arial", "Size"=0.0, "Color"=0, "Style"={"Bold"=TRUE, "Italic"=FALSE, "Underline"=FALSE, "Strikeout"=FALSE}, "Type"={"Type&direction"=enum."ASCII", "Embedded"=FALSE, "Encoding"=""}}}]}, {"Row"={"From #"=1, "to #"=1}, "Cell [ ]"=[{"Text"={"Cell Alignment"=5, "Text rotation"=enum."None", "Line spacing"=enum."Select"}, "Cell Appearance"={"Border"=0, "Thickness"=1.0, "Color"=0, "BG"=16777225}, "HMerge"={"From"=-1, "to"=-1}, "VMerge"={"From"=-1, "to"=-1}, "Font"={"Name"="Arial", "Size"=-1.0, "Color"=0, "Style"={"Bold"=FALSE, "Italic"=FALSE, "Underline"=FALSE, "Strikeout"=FALSE}, "Type"={"Type&direction"=enum."Select", "Embedded"=FALSE, "Encoding"=""}}}, {"Text"={"Cell Alignment"=5, "Text rotation"=enum."Clockwise", "Line spacing"=enum."Select"}, "Cell Appearance"={"Border"=2, "Thickness"=1.0, "Color"=0, "BG"=16777225}, "HMerge"={"From"=-1, "to"=-1}, "VMerge"={"From"=-1, "to"=-1}, "Font"={"Name"="Arial", "Size"=0.0, "Color"=0, "Style"={"Bold"=TRUE, "Italic"=FALSE, "Underline"=FALSE, "Strikeout"=FALSE}, "Type"={"Type&direction"=enum."Select", "Embedded"=FALSE, "Encoding"=""}}}, {"Text"={"Cell Alignment"=5, "Text rotation"=enum."Clockwise", "Line spacing"=enum."Select"}, "Cell Appearance"={"Border"=2, "Thickness"=1.0, "Color"=0, "BG"=16777225}, "HMerge"={"From"=-1, "to"=-1}, "VMerge"={"From"=-1, "to"=-1}, "Font"={"Name"="Arial", "Size"=0.0, "Color"=0, "Style"={"Bold"=TRUE, "Italic"=FALSE, "Underline"=FALSE, "Strikeout"=FALSE}, "Type"={"Type&direction"=enum."Select", "Embedded"=FALSE, "Encoding"=""}}}, {"Text"={"Cell Alignment"=5, "Text rotation"=enum."Clockwise", "Line spacing"=enum."Select"}, "Cell Appearance"={"Border"=2, "Thickness"=1.0, "Color"=0, "BG"=16777225}, "HMerge"={"From"=-1, "to"=-1}, "VMerge"={"From"=-1, "to"=-1}, "Font"={"Name"="Arial", "Size"=0.0, "Color"=0, "Style"={"Bold"=TRUE, "Italic"=FALSE, "Underline"=FALSE, "Strikeout"=FALSE}, "Type"={"Type&direction"=enum."Select", "Embedded"=FALSE, "Encoding"=""}}}, {"Text"={"Cell Alignment"=5, "Text rotation"=enum."Clockwise", "Line spacing"=enum."Select"}, "Cell Appearance"={"Border"=2, "Thickness"=1.0, "Color"=0, "BG"=16777225}, "HMerge"={"From"=-1, "to"=-1}, "VMerge"={"From"=-1, "to"=-1}, "Font"={"Name"="Arial", "Size"=0.0, "Color"=0, "Style"={"Bold"=TRUE, "Italic"=FALSE, "Underline"=FALSE, "Strikeout"=FALSE}, "Type"={"Type&direction"=enum."Select", "Embedded"=FALSE, "Encoding"=""}}}, {"Text"={"Cell Alignment"=5, "Text rotation"=enum."Clockwise", "Line spacing"=enum."Select"}, "Cell Appearance"={"Border"=2, "Thickness"=1.0, "Color"=0, "BG"=16777225}, "HMerge"={"From"=-1, "to"=-1}, "VMerge"={"From"=-1, "to"=-1}, "Font"={"Name"="Arial", "Size"=0.0, "Color"=0, "Style"={"Bold"=TRUE, "Italic"=FALSE, "Underline"=FALSE, "Strikeout"=FALSE}, "Type"={"Type&direction"=enum."Select", "Embedded"=FALSE, "Encoding"=""}}}, {"Text"={"Cell Alignment"=5, "Text rotation"=enum."Clockwise", "Line spacing"=enum."Select"}, "Cell Appearance"={"Border"=3, "Thickness"=1.0, "Color"=0, "BG"=16777225}, "HMerge"={"From"=-1, "to"=-1}, "VMerge"={"From"=-1, "to"=-1}, "Font"={"Name"="Arial", "Size"=0.0, "Color"=0, "Style"={"Bold"=TRUE, "Italic"=FALSE, "Underline"=FALSE, "Strikeout"=FALSE}, "Type"={"Type&direction"=enum."Select", "Embedded"=FALSE, "Encoding"=""}}}]}, {"Row"={"From #"=2, "to #"=-2}, "Cell [ ]"=[{"Text"={"Cell Alignment"=4, "Text rotation"=enum."None", "Line spacing"=enum."Select"}, "Cell Appearance"={"Border"=5, "Thickness"=0.5, "Color"=0, "BG"=16777225}, "HMerge"={"From"=-1, "to"=-1}, "VMerge"={"From"=-1, "to"=-1}, "Font"={"Name"="", "Size"=-1.0, "Color"=16777222, "Style"={"Bold"=FALSE, "Italic"=FALSE, "Underline"=FALSE, "Strikeout"=FALSE}, "Type"={"Type&direction"=enum."Select", "Embedded"=FALSE, "Encoding"=""}}}, {"Text"={"Cell Alignment"=1, "Text rotation"=enum."None", "Line spacing"=enum."Select"}, "Cell Appearance"={"Border"=17, "Thickness"=0.5, "Color"=0, "BG"=16777225}, "HMerge"={"From"=-1, "to"=-1}, "VMerge"={"From"=-1, "to"=-1}, "Font"={"Name"="", "Size"=0.0, "Color"=0, "Style"={"Bold"=FALSE, "Italic"=FALSE, "Underline"=FALSE, "Strikeout"=FALSE}, "Type"={"Type&direction"=enum."Select", "Embedded"=FALSE, "Encoding"=""}}}, {"Text"={"Cell Alignment"=5, "Text rotation"=enum."None", "Line spacing"=enum."Select"}, "Cell Appearance"={"Border"=17, "Thickness"=0.5, "Color"=0, "BG"=16777225}, "HMerge"={"From"=-1, "to"=-1}, "VMerge"={"From"=-1, "to"=-1}, "Font"={"Name"="", "Size"=0.0, "Color"=0, "Style"={"Bold"=FALSE, "Italic"=FALSE, "Underline"=FALSE, "Strikeout"=FALSE}, "Type"={"Type&direction"=enum."Select", "Embedded"=FALSE, "Encoding"=""}}}, {"Text"={"Cell Alignment"=9, "Text rotation"=enum."None", "Line spacing"=enum."Select"}, "Cell Appearance"={"Border"=17, "Thickness"=0.5, "Color"=0, "BG"=16777225}, "HMerge"={"From"=-1, "to"=-1}, "VMerge"={"From"=-1, "to"=-1}, "Font"={"Name"="", "Size"=0.0, "Color"=0, "Style"={"Bold"=FALSE, "Italic"=FALSE, "Underline"=FALSE, "Strikeout"=FALSE}, "Type"={"Type&direction"=enum."Select", "Embedded"=FALSE, "Encoding"=""}}}, {"Text"={"Cell Alignment"=5, "Text rotation"=enum."None", "Line spacing"=enum."Select"}, "Cell Appearance"={"Border"=17, "Thickness"=0.5, "Color"=0, "BG"=16777225}, "HMerge"={"From"=-1, "to"=-1}, "VMerge"={"From"=-1, "to"=-1}, "Font"={"Name"="", "Size"=0.0, "Color"=0, "Style"={"Bold"=FALSE, "Italic"=FALSE, "Underline"=FALSE, "Strikeout"=FALSE}, "Type"={"Type&direction"=enum."Select", "Embedded"=FALSE, "Encoding"=""}}}, {"Text"={"Cell Alignment"=5, "Text rotation"=enum."None", "Line spacing"=enum."Select"}, "Cell Appearance"={"Border"=17, "Thickness"=0.5, "Color"=0, "BG"=16777225}, "HMerge"={"From"=-1, "to"=-1}, "VMerge"={"From"=-1, "to"=-1}, "Font"={"Name"="", "Size"=0.0, "Color"=0, "Style"={"Bold"=FALSE, "Italic"=FALSE, "Underline"=FALSE, "Strikeout"=FALSE}, "Type"={"Type&direction"=enum."Select", "Embedded"=FALSE, "Encoding"=""}}}, {"Text"={"Cell Alignment"=5, "Text rotation"=enum."None", "Line spacing"=enum."Select"}, "Cell Appearance"={"Border"=17, "Thickness"=0.5, "Color"=0, "BG"=16777225}, "HMerge"={"From"=-1, "to"=-1}, "VMerge"={"From"=-1, "to"=-1}, "Font"={"Name"="", "Size"=0.0, "Color"=0, "Style"={"Bold"=FALSE, "Italic"=FALSE, "Underline"=FALSE, "Strikeout"=FALSE}, "Type"={"Type&direction"=enum."Select", "Embedded"=FALSE, "Encoding"=""}}}]}, {"Row"={"From #"=-1, "to #"=-1}, "Cell [ ]"=[{"Text"={"Cell Alignment"=5, "Text rotation"=enum."None", "Line spacing"=enum."Select"}, "Cell Appearance"={"Border"=5, "Thickness"=1.0, "Color"=0, "BG"=15000804}, "HMerge"={"From"=-1, "to"=-1}, "VMerge"={"From"=-1, "to"=-1}, "Font"={"Name"="", "Size"=-1.0, "Color"=16777222, "Style"={"Bold"=TRUE, "Italic"=FALSE, "Underline"=FALSE, "Strikeout"=FALSE}, "Type"={"Type&direction"=enum."Select", "Embedded"=FALSE, "Encoding"=""}}}, {"Text"={"Cell Alignment"=5, "Text rotation"=enum."None", "Line spacing"=enum."Select"}, "Cell Appearance"={"Border"=18, "Thickness"=1.0, "Color"=0, "BG"=15000804}, "HMerge"={"From"=-1, "to"=-1}, "VMerge"={"From"=-1, "to"=-1}, "Font"={"Name"="", "Size"=0.0, "Color"=0, "Style"={"Bold"=TRUE, "Italic"=FALSE, "Underline"=FALSE, "Strikeout"=FALSE}, "Type"={"Type&direction"=enum."Select", "Embedded"=FALSE, "Encoding"=""}}}, {"Text"={"Cell Alignment"=5, "Text rotation"=enum."None", "Line spacing"=enum."Select"}, "Cell Appearance"={"Border"=18, "Thickness"=1.0, "Color"=0, "BG"=15000804}, "HMerge"={"From"=-1, "to"=-1}, "VMerge"={"From"=-1, "to"=-1}, "Font"={"Name"="", "Size"=0.0, "Color"=0, "Style"={"Bold"=TRUE, "Italic"=FALSE, "Underline"=FALSE, "Strikeout"=FALSE}, "Type"={"Type&direction"=enum."Select", "Embedded"=FALSE, "Encoding"=""}}}, {"Text"={"Cell Alignment"=5, "Text rotation"=enum."None", "Line spacing"=enum."Select"}, "Cell Appearance"={"Border"=18, "Thickness"=1.0, "Color"=0, "BG"=15000804}, "HMerge"={"From"=-1, "to"=-1}, "VMerge"={"From"=-1, "to"=-1}, "Font"={"Name"="", "Size"=0.0, "Color"=0, "Style"={"Bold"=TRUE, "Italic"=FALSE, "Underline"=FALSE, "Strikeout"=FALSE}, "Type"={"Type&direction"=enum."Select", "Embedded"=FALSE, "Encoding"=""}}}, {"Text"={"Cell Alignment"=5, "Text rotation"=enum."None", "Line spacing"=enum."Select"}, "Cell Appearance"={"Border"=18, "Thickness"=1.0, "Color"=0, "BG"=15000804}, "HMerge"={"From"=-1, "to"=-1}, "VMerge"={"From"=-1, "to"=-1}, "Font"={"Name"="", "Size"=0.0, "Color"=0, "Style"={"Bold"=TRUE, "Italic"=FALSE, "Underline"=FALSE, "Strikeout"=FALSE}, "Type"={"Type&direction"=enum."Select", "Embedded"=FALSE, "Encoding"=""}}}, {"Text"={"Cell Alignment"=5, "Text rotation"=enum."None", "Line spacing"=enum."Select"}, "Cell Appearance"={"Border"=18, "Thickness"=1.0, "Color"=0, "BG"=15000804}, "HMerge"={"From"=-1, "to"=-1}, "VMerge"={"From"=-1, "to"=-1}, "Font"={"Name"="", "Size"=0.0, "Color"=0, "Style"={"Bold"=TRUE, "Italic"=FALSE, "Underline"=FALSE, "Strikeout"=FALSE}, "Type"={"Type&direction"=enum."Select", "Embedded"=FALSE, "Encoding"=""}}}, {"Text"={"Cell Alignment"=5, "Text rotation"=enum."None", "Line spacing"=enum."Select"}, "Cell Appearance"={"Border"=18, "Thickness"=1.0, "Color"=0, "BG"=15000804}, "HMerge"={"From"=-1, "to"=-1}, "VMerge"={"From"=-1, "to"=-1}, "Font"={"Name"="", "Size"=0.0, "Color"=0, "Style"={"Bold"=TRUE, "Italic"=FALSE, "Underline"=FALSE, "Strikeout"=FALSE}, "Type"={"Type&direction"=enum."Select", "Embedded"=FALSE, "Encoding"=""}}}]}]
  in  "Column Headers 2D [ ] - table 6":string[][](array[string])=[["Permission", "Bit position", "Meaning"]]
  in  "Text Data 2D [ ] - table 6":string[][](array[string])=[["3", "打印文档。 打印文档（可能不是最高质量级别，取决于是否也设置了第 12 位）。Print the document. Print the document (possibly not at the highest quality level, depending on whether bit 12 is also set). "], ["4", "通过第 6、9 和 11 位控制的操作以外的操作修改文档的内容。Modify the contents of the document by operations other than those controlled by bits 6, 9, and 11. "], ["5", "复制或以其他方式从文档中提取文本和图形，包括提取文本和图形（以支持残障用户的可访问性或用于其他目的）。 通过第 10 位控制之外的操作从文档中复制或提取文本和图形。Copy or otherwise extract text and graphics from the document, including extracting text and graphics (in support of accessibility to users with disabilities or for other purposes). Copy or otherwise extract text and graphics from the document by operations other than that controlled by bit 10. "], ["6", "添加或修改文本注释，填写交互式表单域，如果还设置了第 4 位，则创建或修改交互式表单域（包括签名域）。Add or modify text annotations, fill in interactive form fields, and, if bit 4 is also set, create or modify interactive form fields (including signature fields). "], ["9", "填写现有的交互式表单字段（包括签名字段），即使第 6 位已清除。Fill in existing interactive form fields (including signature fields), even if bit 6 is clear. "], ["10", "提取文本和图形（以支持残障用户的可访问性或用于其他目的）。Extract text and graphics (in support of accessibility to users with disabilities or for other purposes). "], ["11", "组合文档（插入、旋转或删除页面并创建书签或缩略图图像），即使位 4 已清除。Assemble the document (insert, rotate, or delete pages and create bookmarks or thumbnail images), even if bit 4 is clear. "], ["12", "将文档打印成可以生成 PDF 内容的忠实数字副本的表示形式。 当该位清零（且位 3 已设置）时，打印仅限于外观的低级表示，质量可能会下降。Print the document to a representation from which a faithful digital copy of the PDF content could be generated. When this bit is clear (and bit 3 is set), printing is limited to a low-level representation of the appearance, possibly of degraded quality. "]]
  in  "Row Headers 1D [ ] - table 6":string[](array[string])=["Allow Degradated Printing", "Allow Modify Contents", "Allow Copy", "Allow Modify Annotations", "Allow Fill In", "Allow Screen Readers", "Allow Assembly", "Allow Printing"]
  in  "Table columnWidth [ ] - table 6":sgl[](array[numeric])=[1.9, 0.7, 3.9]
  in  "Row  [ ] - table 6":T56=[{"Row"={"From #"=0, "to #"=0}, "Cell [ ]"=[{"Text"={"Cell Alignment"=5, "Text rotation"=enum."None", "Line spacing"=enum."Select"}, "Cell Appearance"={"Border"=5, "Thickness"=1.0, "Color"=0, "BG"=16777225}, "HMerge"={"From"=-1, "to"=-1}, "VMerge"={"From"=-1, "to"=-1}, "Font"={"Name"="", "Size"=0.0, "Color"=0, "Style"={"Bold"=FALSE, "Italic"=FALSE, "Underline"=FALSE, "Strikeout"=FALSE}, "Type"={"Type&direction"=enum."Select", "Embedded"=FALSE, "Encoding"=""}}}, {"Text"={"Cell Alignment"=5, "Text rotation"=enum."None", "Line spacing"=enum."Select"}, "Cell Appearance"={"Border"=18, "Thickness"=1.0, "Color"=0, "BG"=16777225}, "HMerge"={"From"=-1, "to"=-1}, "VMerge"={"From"=-1, "to"=-1}, "Font"={"Name"="", "Size"=0.0, "Color"=0, "Style"={"Bold"=FALSE, "Italic"=FALSE, "Underline"=FALSE, "Strikeout"=FALSE}, "Type"={"Type&direction"=enum."Select", "Embedded"=FALSE, "Encoding"=""}}}, {"Text"={"Cell Alignment"=5, "Text rotation"=enum."None", "Line spacing"=enum."Select"}, "Cell Appearance"={"Border"=18, "Thickness"=1.0, "Color"=0, "BG"=16777225}, "HMerge"={"From"=-1, "to"=-1}, "VMerge"={"From"=-1, "to"=-1}, "Font"={"Name"="", "Size"=0.0, "Color"=0, "Style"={"Bold"=FALSE, "Italic"=FALSE, "Underline"=FALSE, "Strikeout"=FALSE}, "Type"={"Type&direction"=enum."Select", "Embedded"=FALSE, "Encoding"=""}}}]}, {"Row"={"From #"=1, "to #"=-1}, "Cell [ ]"=[{"Text"={"Cell Alignment"=4, "Text rotation"=enum."None", "Line spacing"=enum."Select"}, "Cell Appearance"={"Border"=3, "Thickness"=0.5, "Color"=0, "BG"=16777225}, "HMerge"={"From"=-1, "to"=-1}, "VMerge"={"From"=-1, "to"=-1}, "Font"={"Name"="", "Size"=0.0, "Color"=0, "Style"={"Bold"=FALSE, "Italic"=FALSE, "Underline"=FALSE, "Strikeout"=FALSE}, "Type"={"Type&direction"=enum."Select", "Embedded"=FALSE, "Encoding"=""}}}, {"Text"={"Cell Alignment"=5, "Text rotation"=enum."None", "Line spacing"=enum."Select"}, "Cell Appearance"={"Border"=17, "Thickness"=0.5, "Color"=0, "BG"=16777225}, "HMerge"={"From"=-1, "to"=-1}, "VMerge"={"From"=-1, "to"=-1}, "Font"={"Name"="", "Size"=0.0, "Color"=0, "Style"={"Bold"=FALSE, "Italic"=FALSE, "Underline"=FALSE, "Strikeout"=FALSE}, "Type"={"Type&direction"=enum."Select", "Embedded"=FALSE, "Encoding"=""}}}, {"Text"={"Cell Alignment"=7, "Text rotation"=enum."None", "Line spacing"=enum."Select"}, "Cell Appearance"={"Border"=17, "Thickness"=0.5, "Color"=0, "BG"=16777225}, "HMerge"={"From"=-1, "to"=-1}, "VMerge"={"From"=-1, "to"=-1}, "Font"={"Name"="", "Size"=0.0, "Color"=0, "Style"={"Bold"=FALSE, "Italic"=FALSE, "Underline"=FALSE, "Strikeout"=FALSE}, "Type"={"Type&direction"=enum."Select", "Embedded"=FALSE, "Encoding"=""}}}]}]
  in  "Caption - table 6":string="来自“文档管理?便携文档格式?第1部分:PDF 1.7 (PDF 32000-1:2008，第61页)”的权限"
  in  "Row  [ ] - Table 7":T56
  in  "Table properties - Table 7":T48={"Table position"=1, "SpacingBefore (points)"=12.0, "SpacingAfter (points)"=12.0} {"Table position" items=["LEFT", "CENTER", "RIGHT"]}
  in  "Text Data 2D [ ] - Table 7":string[][](array[string])
  in  "Column Headers 2D [ ] - Table 7":string[][](array[string])=[["", "ASCII", "UTF-16", "UTF-16 (deault)", "UTF-16 (LTR)", "UTF-16 (RTL)"]]
  in  "Table columnWidth [ ] - Table 7":sgl[](array[numeric])=[3.0, 0.5, 0.5, 0.5, 0.5, 0.5]
  in  "Row Headers 1D [ ] - Table 7":string[](array[string])=["Text palette", "Append Phrase.vi", "Append Paragraph.vi", "Append Paragraph with Link [ ].vi", "Table palette", "Caption for table (not a VI)", "Append Table.vi", "Append Customized Table.vi", "Image palette", "Caption for image (not a VI)", "Header, Footer and Watermark palette", "Append Text HF.vi", "Append Page number HF.vi", "Append Watermark Text.vi", "Table of Contents palette", "Append Chapter bookmark.vi", "Append a Table of Contents.vi"]
  in  "Table properties - Table 8":T48={"Table position"=1, "SpacingBefore (points)"=12.0, "SpacingAfter (points)"=12.0} {"Table position" items=["LEFT", "CENTER", "RIGHT"]}
  in  "Text Data 2D [ ] - Table 8":string[][](array[string])=[["Not supported"], ["Not tested"], ["Tested"]]
  in  "Table columnWidth [ ] - Table 8":sgl[](array[numeric])=[0.5, 1.5]
  in  "Row  [ ] - Table 8":T56=[{"Row"={"From #"=0, "to #"=0}, "Cell [ ]"=[{"Text"={"Cell Alignment"=5, "Text rotation"=enum."None", "Line spacing"=enum."Select"}, "Cell Appearance"={"Border"=8, "Thickness"=0.5, "Color"=0, "BG"=15066597}, "HMerge"={"From"=-1, "to"=-1}, "VMerge"={"From"=-1, "to"=-1}, "Font"={"Name"="", "Size"=-1.0, "Color"=0, "Style"={"Bold"=FALSE, "Italic"=FALSE, "Underline"=FALSE, "Strikeout"=FALSE}, "Type"={"Type&direction"=enum."Select", "Embedded"=FALSE, "Encoding"=""}}}, {"Text"={"Cell Alignment"=4, "Text rotation"=enum."None", "Line spacing"=enum."Select"}, "Cell Appearance"={"Border"=5, "Thickness"=0.5, "Color"=0, "BG"=16777225}, "HMerge"={"From"=-1, "to"=-1}, "VMerge"={"From"=-1, "to"=-1}, "Font"={"Name"="", "Size"=-1.0, "Color"=0, "Style"={"Bold"=FALSE, "Italic"=FALSE, "Underline"=FALSE, "Strikeout"=FALSE}, "Type"={"Type&direction"=enum."Select", "Embedded"=FALSE, "Encoding"=""}}}]}, {"Row"={"From #"=1, "to #"=1}, "Cell [ ]"=[{"Text"={"Cell Alignment"=5, "Text rotation"=enum."None", "Line spacing"=enum."Select"}, "Cell Appearance"={"Border"=2, "Thickness"=0.5, "Color"=0, "BG"=10473471}, "HMerge"={"From"=-1, "to"=-1}, "VMerge"={"From"=-1, "to"=-1}, "Font"={"Name"="", "Size"=-1.0, "Color"=0, "Style"={"Bold"=FALSE, "Italic"=FALSE, "Underline"=FALSE, "Strikeout"=FALSE}, "Type"={"Type&direction"=enum."Select", "Embedded"=FALSE, "Encoding"=""}}}, {"Text"={"Cell Alignment"=4, "Text rotation"=enum."None", "Line spacing"=enum."Select"}, "Cell Appearance"={"Border"=3, "Thickness"=0.5, "Color"=0, "BG"=16777225}, "HMerge"={"From"=-1, "to"=-1}, "VMerge"={"From"=-1, "to"=-1}, "Font"={"Name"="", "Size"=-1.0, "Color"=0, "Style"={"Bold"=FALSE, "Italic"=FALSE, "Underline"=FALSE, "Strikeout"=FALSE}, "Type"={"Type&direction"=enum."Select", "Embedded"=FALSE, "Encoding"=""}}}]}, {"Row"={"From #"=2, "to #"=2}, "Cell [ ]"=[{"Text"={"Cell Alignment"=5, "Text rotation"=enum."None", "Line spacing"=enum."Select"}, "Cell Appearance"={"Border"=2, "Thickness"=0.5, "Color"=0, "BG"=16777224}, "HMerge"={"From"=-1, "to"=-1}, "VMerge"={"From"=-1, "to"=-1}, "Font"={"Name"="", "Size"=-1.0, "Color"=0, "Style"={"Bold"=FALSE, "Italic"=FALSE, "Underline"=FALSE, "Strikeout"=FALSE}, "Type"={"Type&direction"=enum."Select", "Embedded"=FALSE, "Encoding"=""}}}, {"Text"={"Cell Alignment"=4, "Text rotation"=enum."None", "Line spacing"=enum."Select"}, "Cell Appearance"={"Border"=3, "Thickness"=0.5, "Color"=0, "BG"=16777225}, "HMerge"={"From"=-1, "to"=-1}, "VMerge"={"From"=-1, "to"=-1}, "Font"={"Name"="", "Size"=-1.0, "Color"=0, "Style"={"Bold"=FALSE, "Italic"=FALSE, "Underline"=FALSE, "Strikeout"=FALSE}, "Type"={"Type&direction"=enum."Select", "Embedded"=FALSE, "Encoding"=""}}}]}]
  in  "Row Headers 1D [ ] - Table 8":string[](array[string])=[" ", "  ", " "]
  # "A"
  # "User Password(一般用户密码)"
  # "第二种，所有者密码（ownerpassword），是用来限制用户复制，编辑和打印PDF的密码。有了这种密码，别人虽然可以打开你的PDF，可是除了打开，就什么都不能做了"
  # "单页-适合页\n（推荐）单页-适合宽度"
  # "在运行时系统中不可用"
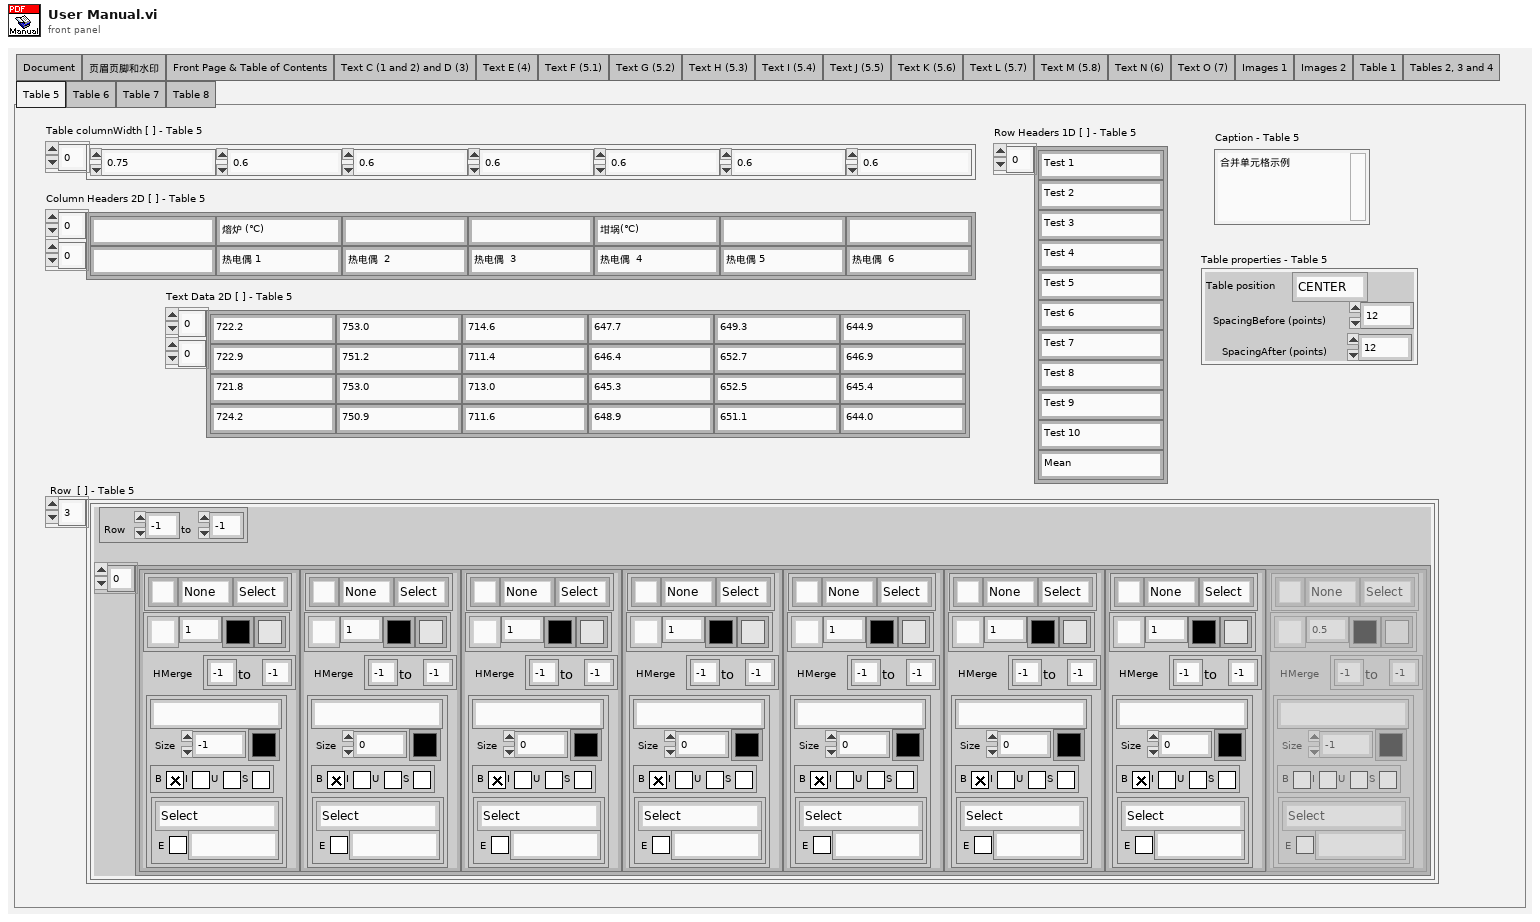
[diagram p1: front panel]
types:
  T1 = enum32{"Document", "页眉页脚和水印", "Front Page & Table of Contents", "Text C (1 and 2) and D (3)", "Text E (4)", "Text F (5.1)", "Text G (5.2)", "Text H (5.3)", "Text I (5.4)", "Text J (5.5)", "Text K (5.6)", "Text L (5.7)", "Text M (5.8)", "Text N (6)", "Text O (7)", "Images 1", "Images 2", "Table 1", "Tables 2, 3 and 4", "Table 5", "Table 6", "Table 7", "Table 8"}
  T2 = typedef "Exaprom PDF.lvlib/Page setup.ctl" = cluster{"Page Size":T3, "Orientation":T4, "Custom Size":T5, "Margins":T6}
  T3 = typedef "Exaprom PDF.lvlib/Page size.ctl" = i32
  T4 = typedef "Exaprom PDF.lvlib/Page Orientation.ctl" = enum16{"Portrait", "Landscape"}
  T5 = typedef "Exaprom PDF.lvlib/Page Layout Custom.ctl" = cluster{"Width":sgl, "Height":sgl}
  T6 = typedef "Exaprom PDF.lvlib/Page margins.ctl" = cluster{"Left":sgl, "Right":sgl, "Top":sgl, "Bottom":sgl}
  T7 = typedef "Exaprom PDF.lvlib/Defaut Paragraphe and Line Spacing.ctl" = cluster{" Aligment":T8, "Line spacing":T9}
  T8 = typedef "Exaprom PDF.lvlib/Texte alignement.ctl" = enum16{"Select", "CENTER", "JUSTIFY", "LEFT", "RIGHT"}
  T9 = typedef "Exaprom PDF.lvlib/Line spacing.ctl" = enum16{"Select", "1.0", "1.5", "2.0"}
  T10 = typedef "Exaprom PDF.lvlib/PDF Details.ctl" = cluster{"Title":string, "Author":string, "Subject":string, "Keywords":string, "Creator":string}
  T11 = typedef "Exaprom PDF.lvlib/Font complete cluster.ctl" = cluster{"Name":string, "Size":T12, "Color":T13, "Style":cluster{"Bold":bool, "Italic":bool, "Underline":bool, "Strikeout":bool}, "Type":T14}
  T12 = typedef "Exaprom PDF.lvlib/Font size.ctl" = sgl
  T13 = typedef "Exaprom PDF.lvlib/Font color.ctl" = u32
  T14 = typedef "Exaprom PDF.lvlib/Type and encoding.ctl" = cluster{"Type&direction":T15, "Embedded":bool, "Encoding":string}
  T15 = typedef "Exaprom PDF.lvlib/Type and run direction.ctl" = enum16{"Select", "ASCII", "UTF-16", "UTF-16 (default)", "UTF-16 (LTR)", "UTF-16 (RTL)"}
  T16 = typedef "Exaprom PDF.lvlib/Captions.ctl" = cluster{"Figure":T17, "Table":T17, "Font":T11}
  T17 = typedef "Exaprom PDF.lvlib/Image or Table Caption.ctl" = cluster{"Caption":string, "Separator":string, "Position":enum16{"Above", "Below"}}
  T18 = typedef "Exaprom PDF.lvlib/Unit.ctl" = enum16{"inch", "mm"}
  T19 = typedef "Exaprom PDF.lvlib/File Permission Parameters.ctl" = cluster{"User Password":string, "Owner Password":string, "Printing":enum16{"Allow Printing", "Allow Degraded Printing", "Don't Allow Printing"}, "Allow Modify Contents":bool, "Allow Copy":bool, "Allow Modify Annotations":bool, "Allow Fill In ":bool, "Allow Screen Readers":bool, "Allow Assembly":bool}
  T20 = typedef "Exaprom PDF.lvlib/At the opening.ctl" = cluster{"Page":u16, "Show Bookmarks":bool}
  T21 = typedef "Exaprom PDF.lvlib/Header or Footer  Page # cluster.ctl" = cluster{"Start at page":i32, "Start with #":i32, "Cell Alignment":T22, "Page #":T23, "Font":T24}
  T22 = typedef "Exaprom PDF.lvlib/Cell Alignment 20px.ctl" = u16
  T23 = typedef "Exaprom PDF.lvlib/Page number.ctl" = cluster{"Text 1":string, "Text 2":string, "Text 3":string}
  T24 = typedef "Exaprom PDF.lvlib/Font complete cluster horizontal.ctl" = cluster{"Name":string, "Size":T12, "Color":T13, "Style":cluster{"Bold":bool, "Italic":bool, "Underline":bool, "Strikeout":bool}, "Type":T14}
  T25 = typedef "Exaprom PDF.lvlib/Header or Footer Line cluster.ctl" = cluster{"H/F Line":T26, "Thickness (point)":sgl, " Colour":u32}
  T26 = typedef "Exaprom PDF.lvlib/Header Footer Line.ctl" = enum16{"No line", "Horizontal line"}
  T27 = typedef "Exaprom PDF.lvlib/Header or Footer  Text cluster.ctl" = cluster{"Start at page":i32, "Cell Alignment":T22, "Line spacing":T9, "Text":string, "Font complete":T24, "Link":string}
  T28 = typedef "Exaprom PDF.lvlib/Watermark Image Cluster.ctl" = cluster{"Image path":path, "Opacity (%)":sgl, "Postion":cluster{"Position":T29, "X":sgl, "Y":sgl}, "Automatic":bool, "Scale(%)":sgl, "Rotate(°)":sgl}
  T29 = typedef "Exaprom PDF.lvlib/Watermark Position.ctl" = enum16{"Absolute", "Center (page)", "Center (text section)"}
  T30 = typedef "Exaprom PDF.lvlib/Watermark Text Cluster.ctl" = cluster{"Text ":string, "Opacity (%)":sgl, "Position":cluster{"Position":T29, "X":sgl, "Y":sgl}, "Automatic":bool, "Font":cluster{"Font Name":string, "Size":T12, "Color":T13}, "Alignment":T31, "Rotate(°)":sgl}
  T31 = typedef "Exaprom PDF.lvlib/Header footer horiz alignment.ctl" = enum16{"Left", "Center", "Right"}
  T32 = typedef "Exaprom PDF.lvlib/Header or Footer  Image cluster.ctl" = cluster{"Start at page":i32, "Cell Alignment":T22, "Path":path, "Image (%)":sgl, "Link":string}
  T33 = typedef "Exaprom PDF.lvlib/Text and hyperlink [ ].ctl" = T34[]
  T34 = typedef "Exaprom PDF.lvlib/Text from String of File and hyperlink.ctl" = cluster{"Text":cluster{"Text":string, "Path":path, "Font complete":T24}, "Link":cluster{"Hyperlink":string, "Font complete":T24}, "Paragraphe":T7, "Indentation":T35}
  T35 = typedef "Exaprom PDF.lvlib/Paragraph indentation.ctl" = cluster{"Left":sgl, "Right":sgl}
  T36 = typedef "Exaprom PDF.lvlib/PDF file to concatenate.ctl" = cluster{"Path":path, "Pages":string, "Password":string}
  T37 = typedef "Exaprom PDF.lvlib/Image alignment and position.ctl" = cluster{"Alignment":T38, "X ":sgl, "Y":sgl, "Indentation":sgl}
  T38 = typedef "Exaprom PDF.lvlib/Image aligment.ctl" = enum16{"Absolute (X,Y)", "Left", "Center", "Right", "Left (textwrap)", "Right (textwrap)"}
  T39 = typedef "Exaprom PDF.lvlib/Image border.ctl" = cluster{"Show?":bool, "Thickness (point)":sgl, "Color":u32}
  T40 = cluster{"Scale (%)":sgl, "Position":T37, "Border":T39}
  T41 = typedef "Exaprom PDF.lvlib/Row Predefined borders cluster.ctl" = cluster{"Borders":T42, "Header":cluster{"Thickness":sgl, "Line":u32, "Background ":u32}, "Data":cluster{"Thickness":sgl, "Line":u32, "Background ":u32}}
  T42 = typedef "Exaprom PDF.lvlib/Row Predefined borders.ctl" = u16
  T43 = typedef "Exaprom PDF.lvlib/Image Scale.ctl" = sgl
  T44 = cluster{"Image name":string, "Path":path, "Scale":T43}[]
  T45 = typedef "Exaprom PDF.lvlib/Cell Font, type, Alignment and LS V2.ctl" = cluster{"Cell Type, Alignment and LS":T46, "Font":T11}
  T46 = typedef "Exaprom PDF.lvlib/Cell Type, Alignment and LS.ctl" = cluster{"Cell Alignment":T22, "Text rotation":T47, "Line spacing":T9}
  T47 = typedef "Exaprom PDF.lvlib/Text vertical arrangement.ctl" = enum16{"None", "Clockwise", "Counterclockwise"}
  T48 = typedef "Exaprom PDF.lvlib/Table properties.ctl" = cluster{"Table position":T49, "SpacingBefore (points)":sgl, "SpacingAfter (points)":sgl}
  T49 = typedef "Exaprom PDF.lvlib/Table position.ctl" = i32
  T50 = typedef "Exaprom PDF.lvlib/Simplified Table Row Borders [ ].ctl" = T51[]
  T51 = typedef "Exaprom PDF.lvlib/Simplified Table Row Borders.ctl" = cluster{"Row":cluster{"#":i16, "to #":i16}, "Line":cluster{"Thickness":sgl, "Color":u32}, "Column Borders [ ]":T52}
  T52 = typedef "Exaprom PDF.lvlib/Border and BG Color [ ].ctl" = T53[]
  T53 = typedef "Exaprom PDF.lvlib/Border and BG Color.ctl" = cluster{"Cell Border":T54, "BG":u32}
  T54 = typedef "Exaprom PDF.lvlib/Cell Border 20 px.ctl" = u16
  T55 = typedef "Exaprom PDF.lvlib/Row Back Ground color Datas.ctl" = cluster{"color":u32, "at each":i16}
  T56 = typedef "Exaprom PDF.lvlib/Table Appearance and Font Row [ ].ctl" = T57[]
  T57 = typedef "Exaprom PDF.lvlib/One Row Appearance.ctl" = cluster{"Row":T58, "Cell [ ]":T59[]}
  T58 = typedef "Exaprom PDF.lvlib/Row from to.ctl" = cluster{"From #":i16, "to #":i16}
  T59 = typedef "Exaprom PDF.lvlib/Cell, Alignment, LS and Font - hide Vmerge.ctl" = cluster{"Text":T46, "Cell Appearance":T60, "HMerge":T61, "VMerge":T62, "Font":T11}
  T60 = typedef "Exaprom PDF.lvlib/Cell Appearance.ctl" = cluster{"Border":T54, "Thickness":sgl, "Color":u32, "BG":u32}
  T61 = typedef "Exaprom PDF.lvlib/Merge Horizontal.ctl" = cluster{"From":i8, "to":i8}
  T62 = typedef "Exaprom PDF.lvlib/Merge Vertical.ctl" = cluster{"From":i8, "to":i8}
  T63 = typedef "LVPointTypeDef.ctl" = cluster{"Horizontal":i16, "Vertical":i16}
  T64 = enum16{"open", "replace", "create", "open or create", "replace or create", "replace or create with confirmation"}
  T65 = typedef "Exaprom PDF.lvlib/Chapter.ctl" = enum16{"Chapter - level 1", "Chapter - level 2", "Chapter - level 3", "Chapter - level 4"}
  T66 = typedef "Exaprom PDF.lvlib/Header or Footer.ctl" = enum16{"Header", "Footer"}
  T67 = typedef "Exaprom PDF.lvlib/Image Size Block Diagram.ctl" = cluster{"Maximum Width":i32, "Maximum Height":i32}
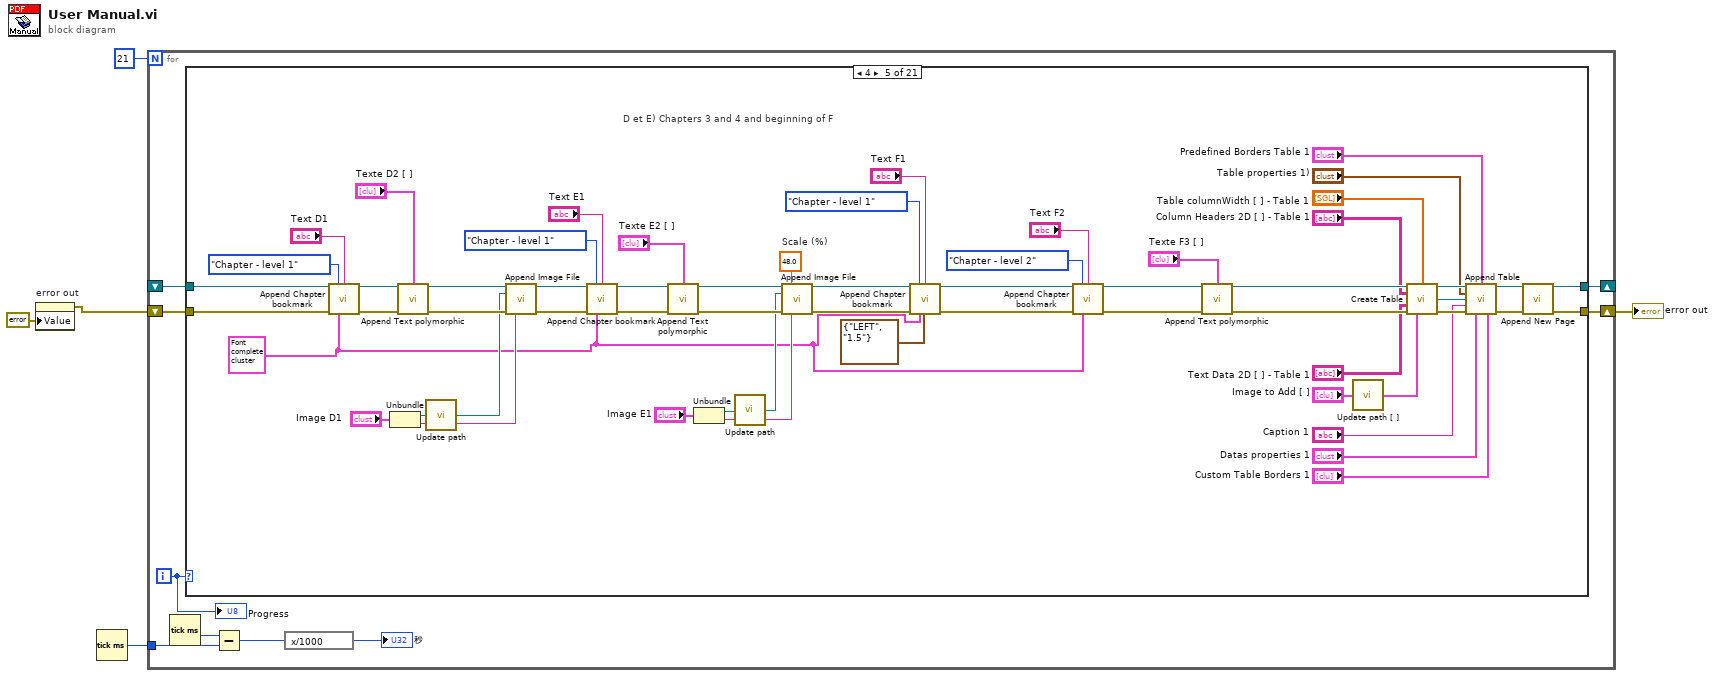
[diagram p0: block diagram]
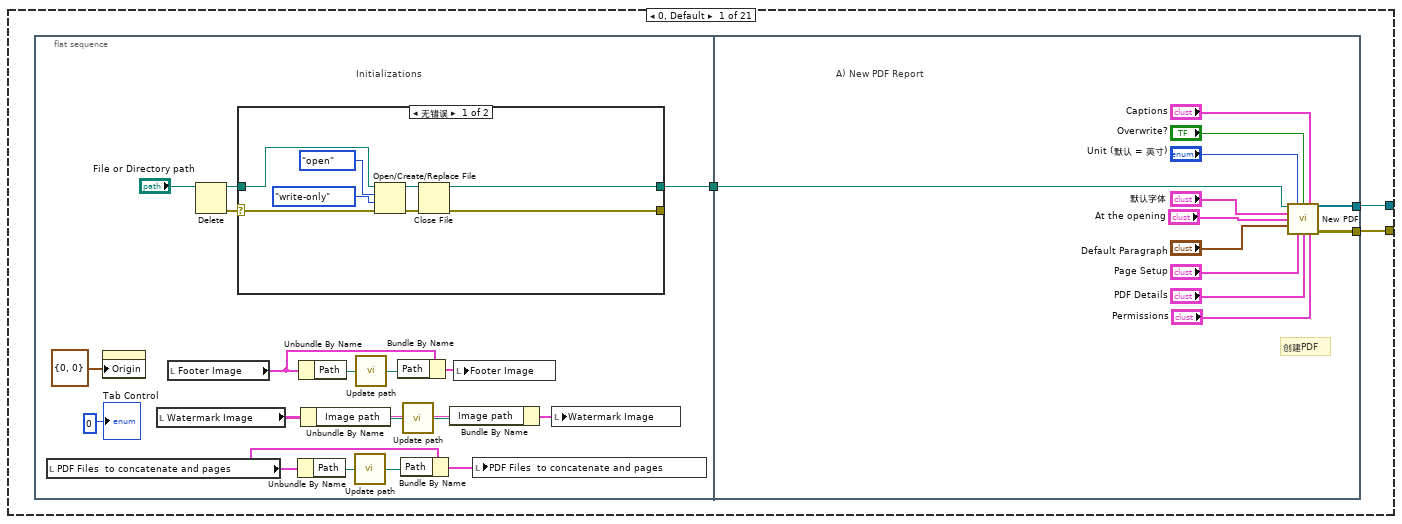
[diagram p2: hidden frame]
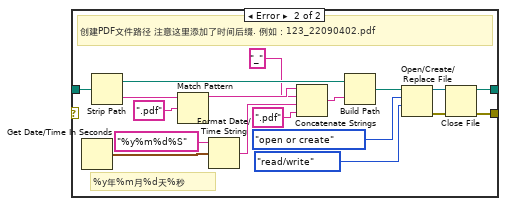
[diagram p3: hidden frame]
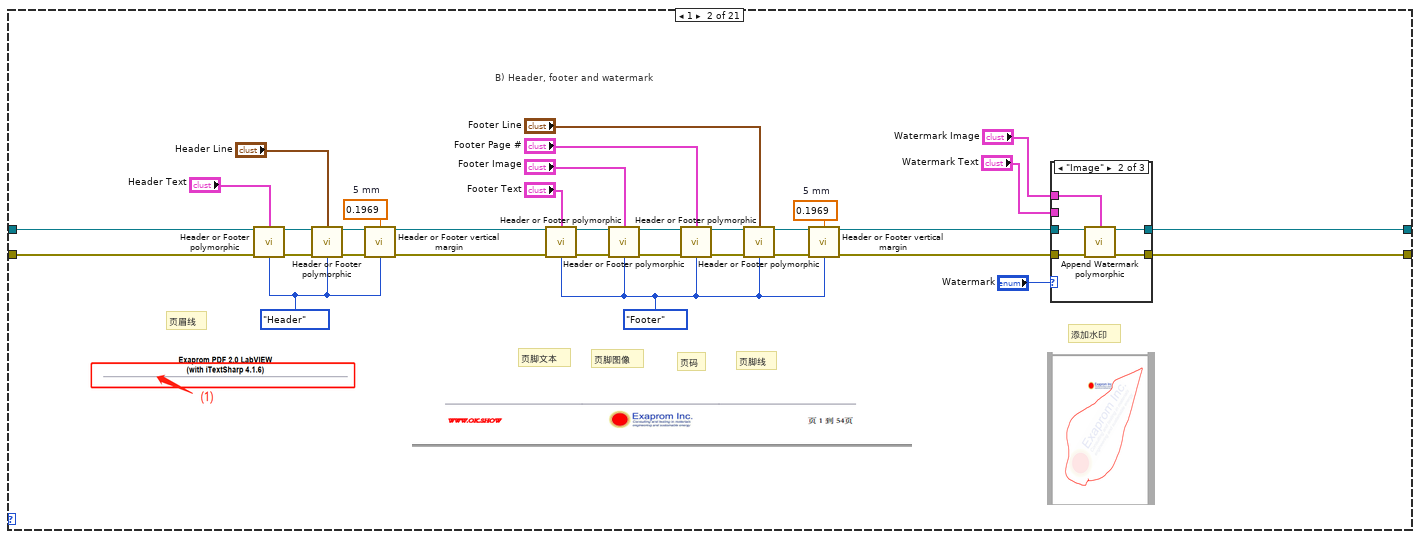
[diagram p4: hidden frame]
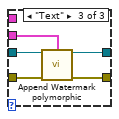
[diagram p6: hidden frame]
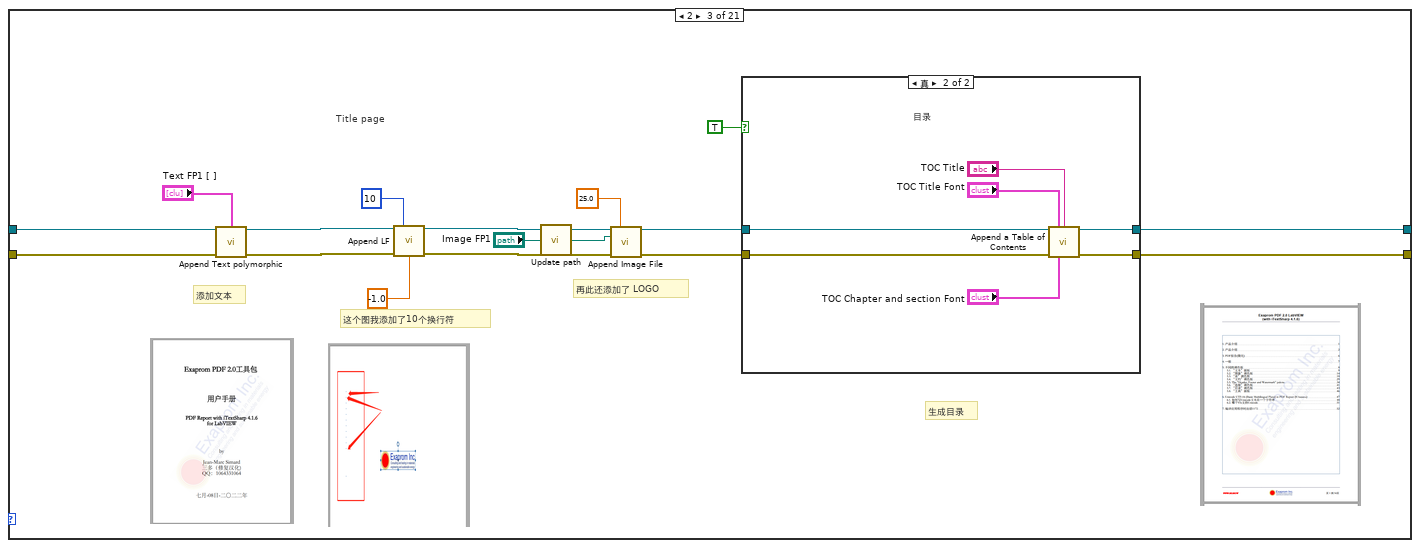
[diagram p7: hidden frame]
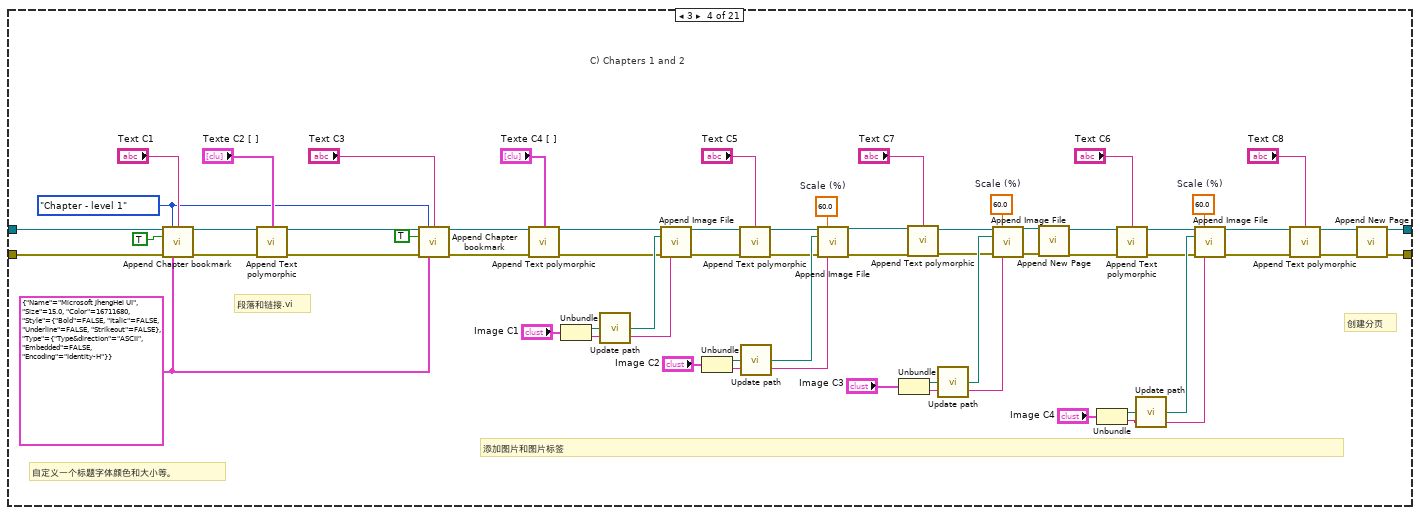
[diagram p9: hidden frame]
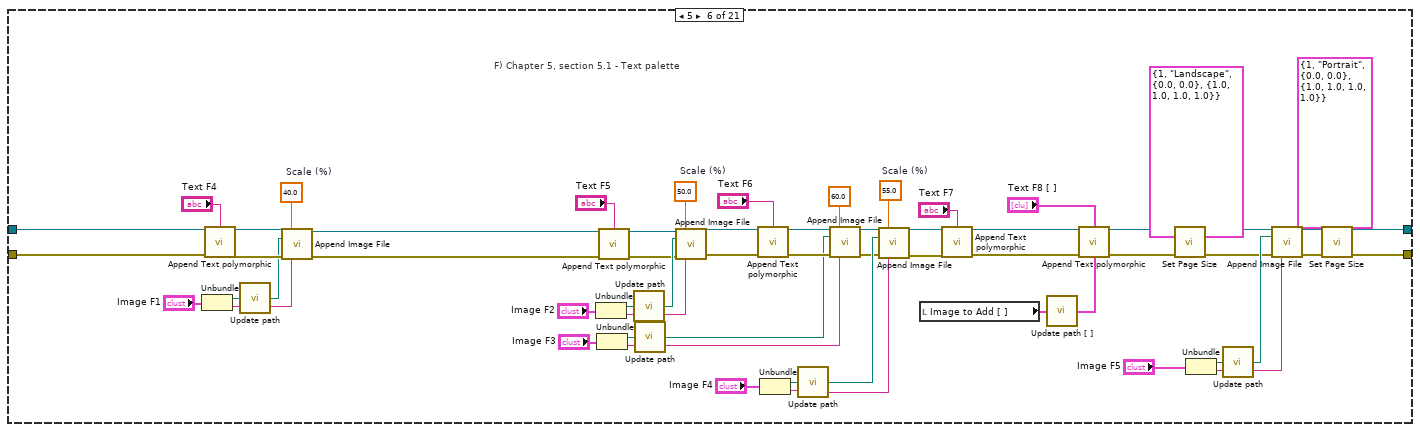
[diagram p10: hidden frame]
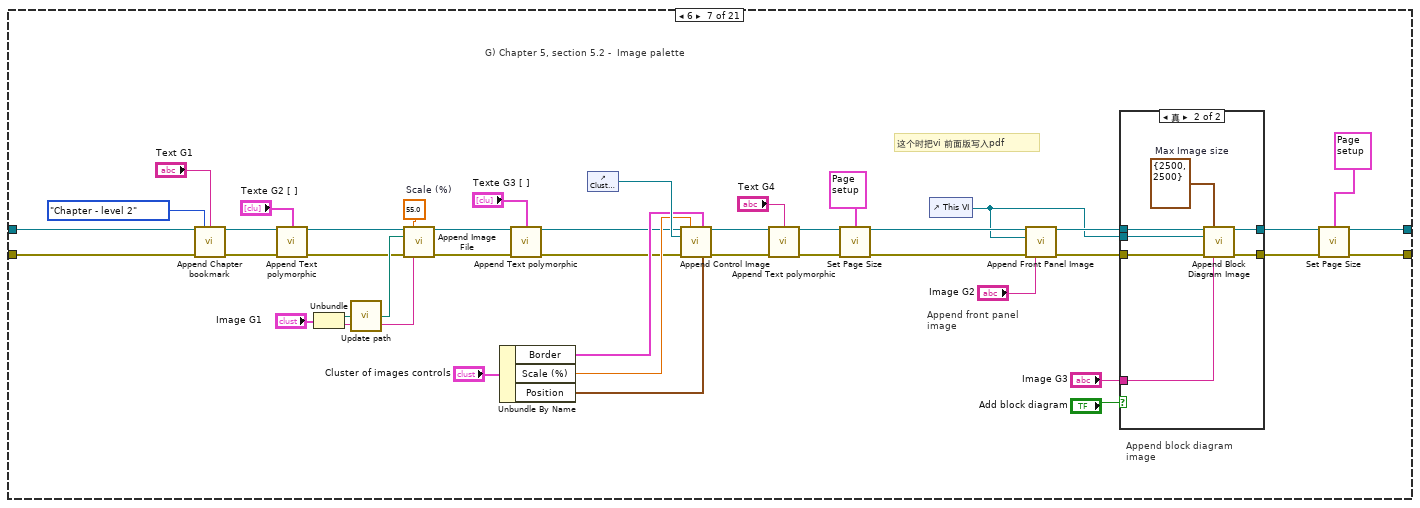
[diagram p11: hidden frame]
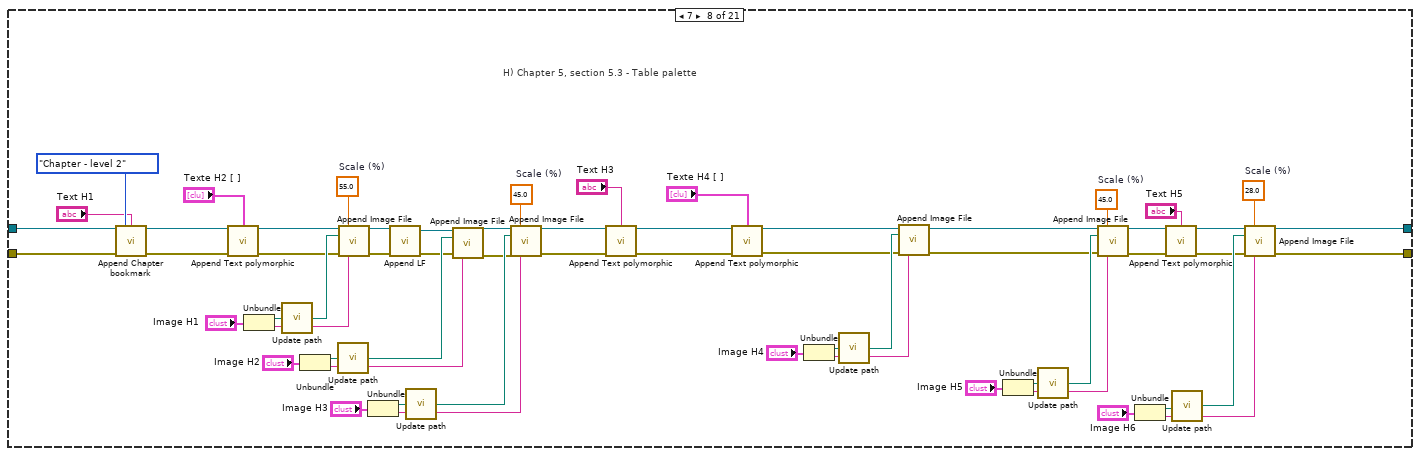
[diagram p13: hidden frame]
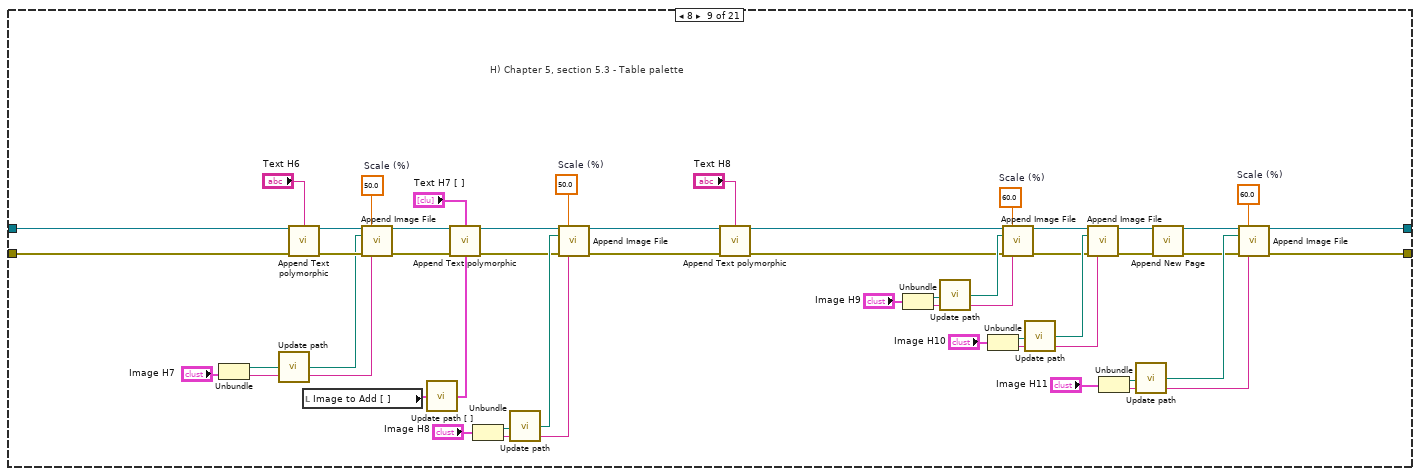
[diagram p14: hidden frame]
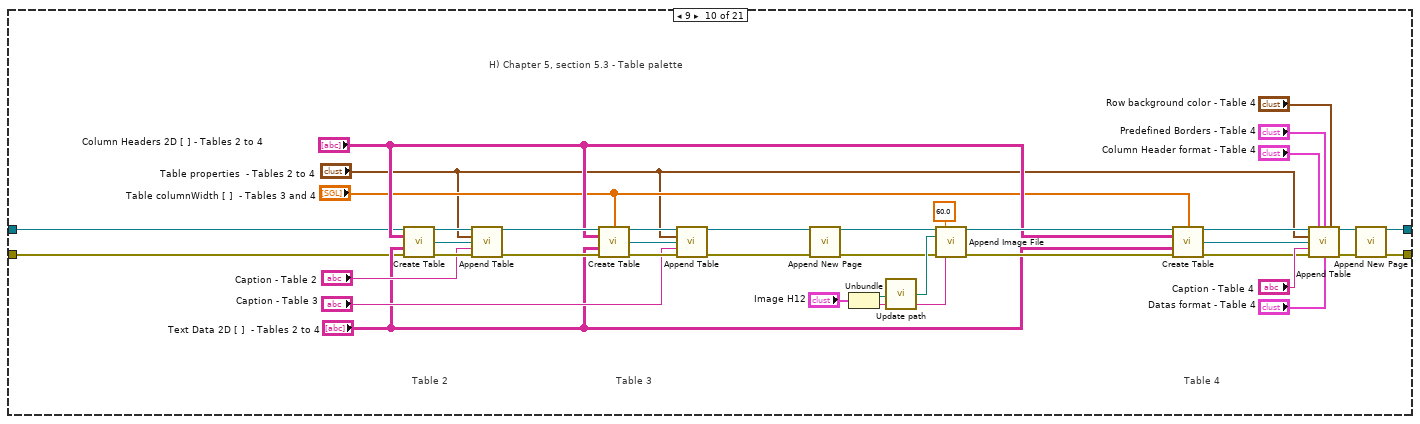
[diagram p15: hidden frame]
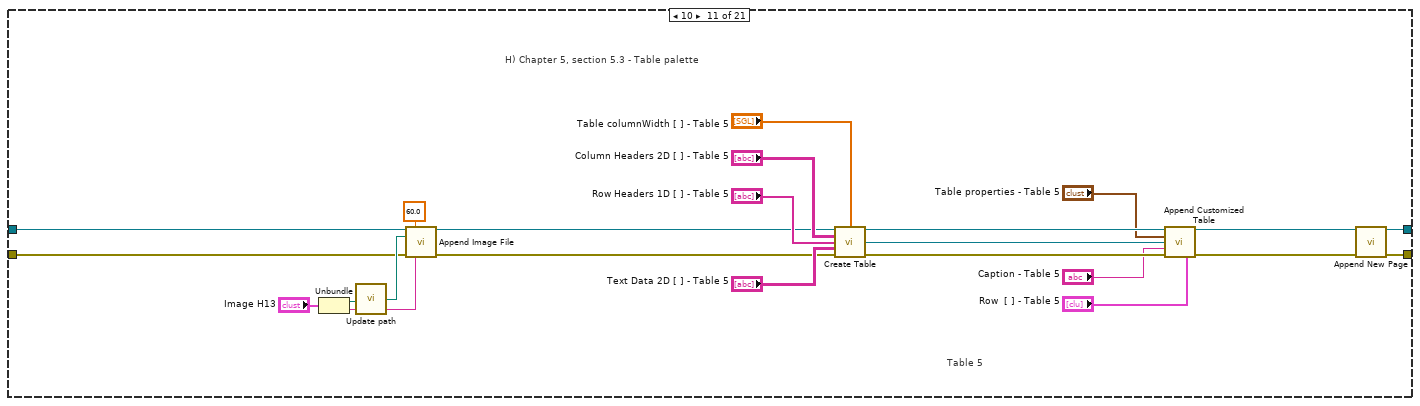
[diagram p16: hidden frame]
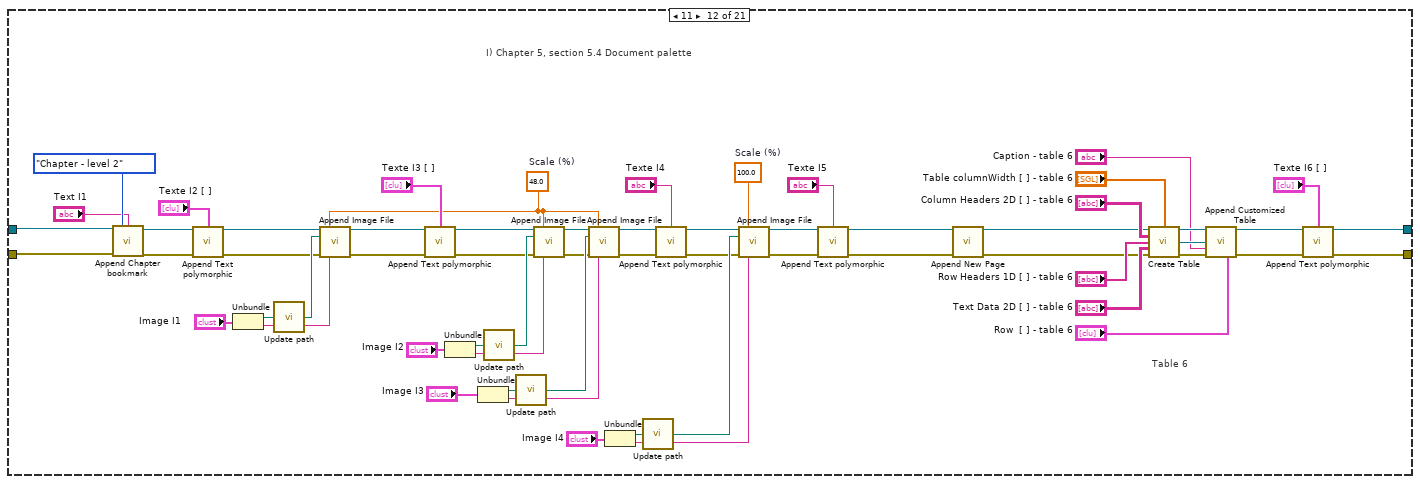
[diagram p17: hidden frame]
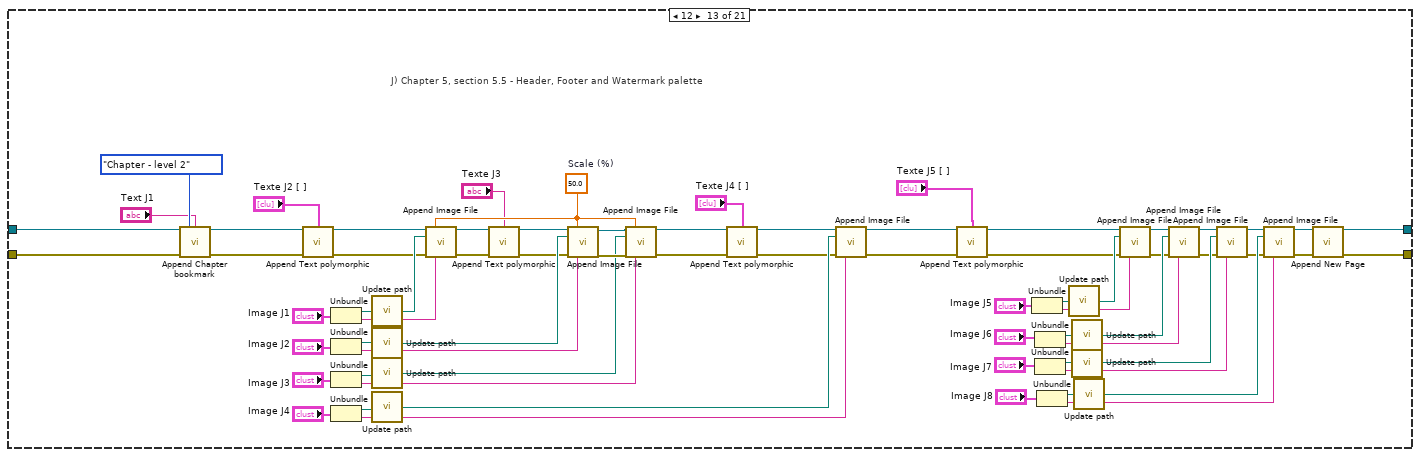
[diagram p18: hidden frame]
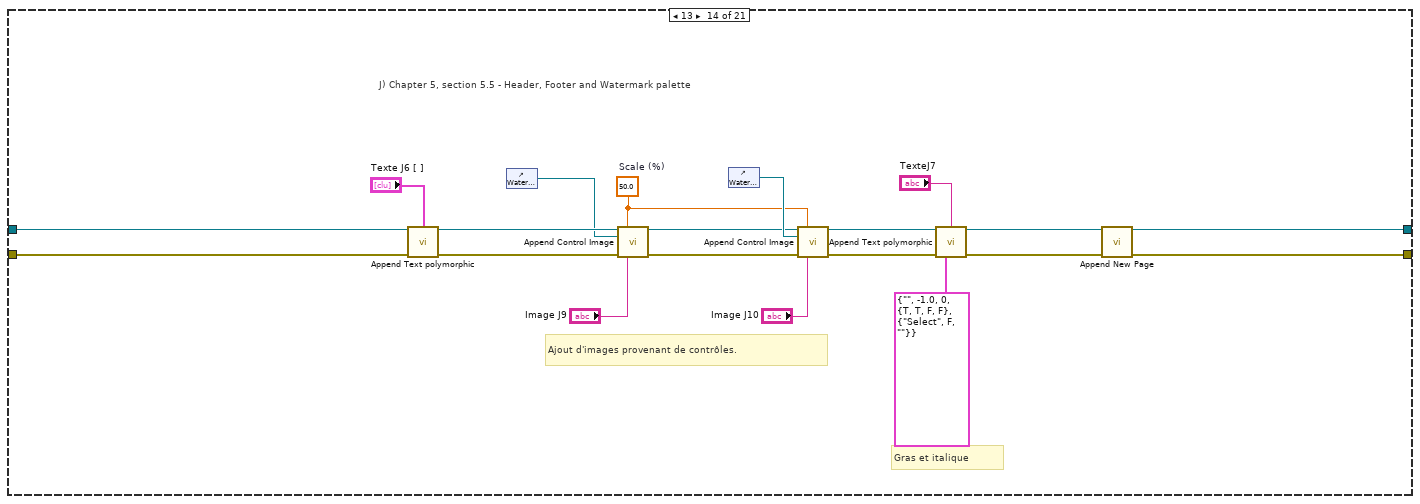
[diagram p19: hidden frame]
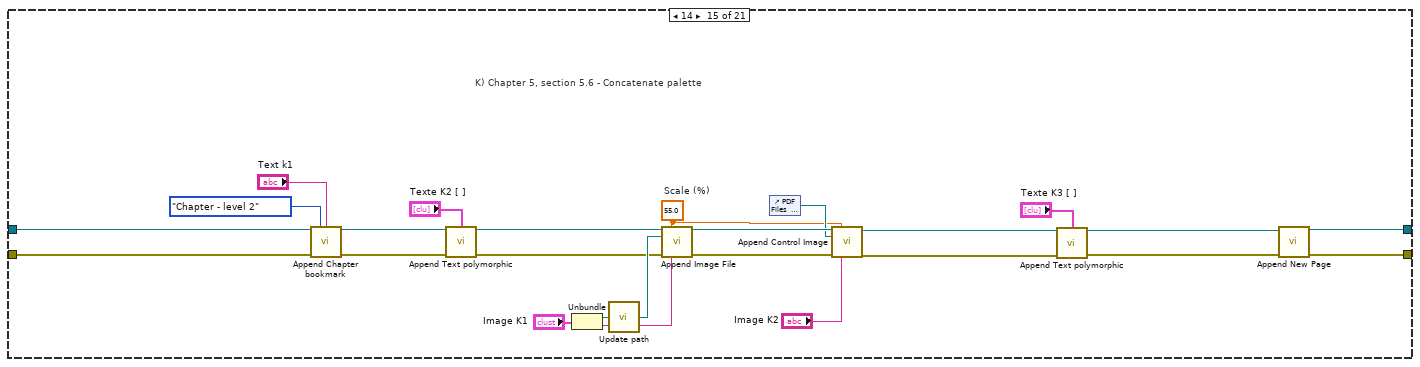
[diagram p20: hidden frame]
diagram:
  n1 = property on="error out" class="Clust (严格)"("Value"=errorcluster {"status"=FALSE, "code"=0, "source"=""} ("错误常量")) -> (error out=w1:errorcluster)  [unwired: 2 in, 1 out]
  n2 = Tick Count (ms)() -> (millisecond timer value=w3:u32)
  n3 = for {
    N: 21 -> [_]
    shift-right: [w13] -> _
    shift-left: _ -> [w12]
    shift-right: [w14] -> w5
    shift-left: w1 -> [w11]
    tunnel: w3 -> [w7]
    i -> [w10]
    n4 = Tick Count (ms)() -> (millisecond timer value=w8:u32)
    n5 = case shown="4" w10 {
      tunnel: [w17 w103 w123 w204 w208 w323 w330 w384 w467 w486 w546 w553 w614 w692 w709 w723 w768 w790 w838 w893 _] -> w13
      tunnel: [w16 w104 w124 w203 w207 w322 w331 w385 w466 w485 w545 w554 w613 w693 w708 w721 w766 w791 w839 w892 w894] -> w14
      tunnel: w12 -> [_ w106 w132 w205 w244 w267 w325 w386 w439 w488 w524 w547 w607 w695 w696 w762 w770 w793 w869 w883 w903]
      tunnel: w11 -> [_ w105 w133 w158 w243 w266 w324 w387 w438 w487 w525 w548 w608 w694 w697 w761 w771 w792 w870 w882 w904]
      frame 0, Default {
        n6 = flat-sequence {
          tunnel: [w19] -> w15
          tunnel: [w73] -> w17
          tunnel: [w72] -> w16
          tunnel: w15 -> [w62]
          frame #0 {
            # "Initializations"
            n7 = local read "PDF Files  to concatenate and pages"() -> (w26:T36)
            n8 = property on="Pane" class="Pane"("Origin"=T63 {"Horizontal"=0, "Vertical"=0}) -> ()  [unwired: 2 in, 2 out]
            n9 = local read "Watermark Image"() -> (w27:T28)
            n10 = local read "Footer Image"() -> (w34:T32)
            n11 = Delete(path (use dialog)="File or Directory path") -> (deleted path=w21:path, error out=w20:errorcluster)  [unwired: 4 in, 1 out]
            n12 = case shown="无错误" w20 {
              selector: w20 -> [w43 _]
              tunnel: [w39 w59] -> w19
              tunnel: [w38 w58] -> _
              tunnel: w21 -> [w37 w57]
              frame No Error {
                n13 = Open/Create/Replace File(file path (use dialog)=w37, error in=w43, operation (0:open)=T64."open" ("操作(0:open)"), access (0:read/write)=enum16{"read/write", "read-only", "write-only"}."write-only" ("权限(0:read/write)")) -> (refnum out=w40:refnum<file>, error out=w41:errorcluster)  [unwired: 2 in, 1 out]
                n14 = Close File(refnum=w40, error in=w41) -> (path=w39:path, error out=w38:errorcluster)
              }
              frame Error {
                # "%y年%m月%d天%秒"
                # "创建PDF文件路径 注意这里添加了时间后缀. 例如：123_22090402.pdf"
                n15 = Get Date/Time In Seconds() -> (seconds since 1Jan1904=w53:timestamp)
                n16 = Strip Path(path=w57) -> (stripped path=w55:path, name=w47:string)
                n17 = Match Pattern(string=w47, regular expression=".pdf" ("正则表达式")) -> (before substring=w45:string)  [unwired: 1 in, 3 out]
                n18 = Format Date/Time String(time format string (%c)="%y%m%d%S" ("时间格式字符串(%c)"), seconds (now)=w53) -> (date/time string=w51:string)  [unwired: 1 in]
                n19 = Concatenate Strings(w45, "_", w51, ".pdf" ("字符串")) -> (w46:string)
                n20 = Build Path(base path=w55, name or relative path=w46) -> (appended path=w56:path)
                n21 = Open/Create/Replace File(file path (use dialog)=w56, operation (0:open)=T64."open or create" ("操作(0:open)"), access (0:read/write)=enum16{"read/write", "read-only", "write-only"}."read/write" ("权限(0:read/write)")) -> (refnum out=w60:refnum<file>, error out=w61:errorcluster)  [unwired: 3 in, 1 out]
                n22 = Close File(refnum=w60, error in=w61) -> (path=w59:path, error out=w58:errorcluster)
              }
            }
            n23 = Unbundle By Name(w26) -> ("Path"=w24:path)
            n24 = Unbundle By Name(w34) -> ("Path"=w32:path)
            n25 = Unbundle By Name(w27) -> ("Image path"=w29:path)
            n26 = call <userlib>:"Update path.vi"("Path IN"=w24) -> ("Path OUT"=w25:path)  [unwired: 1 in, 2 out]
            n27 = call <userlib>:"Update path.vi"("Path IN"=w32) -> ("Path OUT"=w33:path)  [unwired: 1 in, 2 out]
            n28 = Bundle By Name(cluster=w34, "Path"=w33) -> (w31:T32)
            n29 = Bundle By Name(cluster=w26, "Path"=w25) -> (w23:T36)
            n30 = call <userlib>:"Update path.vi"("Path IN"=w29) -> ("Path OUT"=w28:path)  [unwired: 1 in, 2 out]
            n31 = Bundle By Name(cluster=w27, "Image path"=w28) -> (w30:T28)
            n32 = local write "Footer Image"(w31) -> ()
            n33 = local write "PDF Files  to concatenate and pages"(w23) -> ()
            n34 = local write "Watermark Image"(w30) -> ()
            "Tab Control" <- u32 0
          }
          frame #1 {
            # "创建PDF"
            # "A) New PDF Report"
            n35 = call <userlib>:"New PDF.vi"("PDF Path"=w62, "Unit (default = mm)"="Unit (默认 = 英寸)", "Overwrite?"="Overwrite?", "Captions"="Captions", "Default Font"="默认字体", "At the opening"="At the opening", "Default Paragraph"="Default Paragraph", "Page Setup"="Page Setup", "PDF Details"="PDF Details", "Permissions"="Permissions") -> ("PDF Report"=w73:refnum<class "PDF Report Class.lvclass">, "error out"=w72:errorcluster)  [unwired: 1 in, 3 out]
          }
        }
      }
      frame 1 {
        w102 = 0.1969  # 5 mm
        w101 = 0.1969  # 5 mm
        w100 = Header_or_Footer."Header" ("Position")
        w99 = Header_or_Footer."Footer" ("Position")
        # "添加水印"
        # "页脚线"
        # "页码"
        # "页脚图像"
        # "页脚文本"
        # "页眉线"
        # "B) Header, footer and watermark"
        n36 = call-poly <userlib>:"Header or Footer polymorphic.vi"("PDF Report IN"=w106, "Header or footer"="Header Text", "error in (no error)"=w105, "Position"=w100) -> ("PDF Report OUT"=w88:refnum<class "PDF Report Class.lvclass">, "error out"=w87:errorcluster)  [unwired: 10 out]
        n37 = call-poly <userlib>:"Header or Footer polymorphic.vi"("PDF Report IN"=w88, "H/F Line"="Header Line", "error in (no error)"=w87, "Position"=w100) -> ("PDF Report OUT"=w80:refnum<class "PDF Report Class.lvclass">, "error out"=w93:errorcluster)  [unwired: 1 in, 9 out]
        n38 = call <userlib>:"Header or Footer vertical margin.vi"("PDF Report IN"=w80, "Vertical margin"=w101, "error in (no error)"=w93, "Position"=w100) -> ("PDF Report OUT"=w92:refnum<class "PDF Report Class.lvclass">, "error out"=w96:errorcluster)  [unwired: 10 out]
        n39 = call-poly <userlib>:"Header or Footer polymorphic.vi"("PDF Report IN"=w92, "Header or footer"="Footer Text", "error in (no error)"=w96, "Position"=w99) -> ("PDF Report OUT"=w83:refnum<class "PDF Report Class.lvclass">, "error out"=w86:errorcluster)  [unwired: 10 out]
        n40 = call-poly <userlib>:"Header or Footer polymorphic.vi"("PDF Report IN"=w83, "Header or footer"="Footer Image", "error in (no error)"=w86, "Position"=w99) -> ("PDF Report OUT"=w82:refnum<class "PDF Report Class.lvclass">, "error out"=w85:errorcluster)  [unwired: 10 out]
        n41 = call-poly <userlib>:"Header or Footer polymorphic.vi"("PDF Report IN"=w82, "Header or footer"="Footer Page #", "error in (no error)"=w85, "Position"=w99) -> ("PDF Report OUT"=w81:refnum<class "PDF Report Class.lvclass">, "error out"=w84:errorcluster)  [unwired: 10 out]
        n42 = call-poly <userlib>:"Header or Footer polymorphic.vi"("PDF Report IN"=w81, "H/F Line"="Footer Line", "error in (no error)"=w84, "Position"=w99) -> ("PDF Report OUT"=w95:refnum<class "PDF Report Class.lvclass">, "error out"=w94:errorcluster)  [unwired: 1 in, 9 out]
        n43 = call <userlib>:"Header or Footer vertical margin.vi"("PDF Report IN"=w95, "Vertical margin"=w102, "error in (no error)"=w94, "Position"=w99) -> ("PDF Report OUT"=w98:refnum<class "PDF Report Class.lvclass">, "error out"=w97:errorcluster)  [unwired: 10 out]
        n44 = case shown="\"Image\"" "Watermark" {
          tunnel: w97 -> [w107 w113 w118]
          tunnel: w98 -> [w108 w112 w117]
          tunnel: [w108 w111 w116] -> w103
          tunnel: [w107 w110 w115] -> w104
          tunnel: "Watermark Text" -> [_ _ w114]
          tunnel: "Watermark Image" -> [_ w109 _]
          frame "none", Default {
          }
          frame "Image" {
            n45 = call-poly <userlib>:"Append Watermark polymorphic.vi"("PDF Report IN"=w112, "Watermark Image"=w109, "error in (no error)"=w113) -> ("PDF Report OUT"=w111:refnum<class "PDF Report Class.lvclass">, "error out"=w110:errorcluster)  [unwired: 1 in, 10 out]
          }
          frame "Text" {
            n46 = call-poly <userlib>:"Append Watermark polymorphic.vi"("PDF Report IN"=w117, "Watermark Text"=w114, "error in (no error)"=w118) -> ("PDF Report OUT"=w116:refnum<class "PDF Report Class.lvclass">, "error out"=w115:errorcluster)  [unwired: 1 in, 10 out]
          }
        }
      }
      frame 2 {
        # "生成目录"
        # "再此还添加了 LOGO"
        # "这个图我添加了10个换行符"
        # "添加文本"
        # "Title page"
        n47 = call-poly <userlib>:"Append Text polymorphic.vi"("PDF Report"=w132, "Text [ ]"="Text FP1 [ ]", "error in (no error)"=w133) -> ("PDF Report duplicate"=w134:refnum<class "PDF Report Class.lvclass">, "error out"=w127:errorcluster)  [unwired: 1 in, 10 out]
        n48 = call <userlib>:"Append LF.vi"("PDF Report IN"=w134, "Number of LF (default 1)"=u8 10, "error in (no error)"=w127, "One LF (pts)"=sgl -1.0) -> ("PDF Report duplicate"=w128:refnum<class "PDF Report Class.lvclass">, "error out"=w126:errorcluster)  [unwired: 10 in]
        n49 = call <userlib>:"Update path.vi"("Path IN"="Image FP1") -> ("Path OUT"=w130:path)  [unwired: 1 in, 2 out]
        n50 = call <userlib>:"Append Image File.vi"("PDF Report IN"=w128, "Scale (%)"=sgl 25.0, "Image path"=w130, "error in (no error)"=w126) -> ("PDF Report OUT"=w122:refnum<class "PDF Report Class.lvclass">, "error out"=w121:errorcluster)  [unwired: 8 in, 2 out]
        n51 = case shown="真" TRUE {
          tunnel: [w136 w144] -> w124
          tunnel: [w137 w143] -> w123
          tunnel: w122 -> [w137 w142]
          tunnel: w121 -> [w136 w141]
          frame False {
          }
          frame True {
            # "目录"
            n52 = call <userlib>:"Append a Table of Contents.vi"("PDF Report IN"=w142, "Title Font"="TOC Title Font", "Title"="TOC Title", "error in (no error)"=w141, "Chapter and section Font"="TOC Chapter and section Font") -> ("PDF Report OUT"=w143:refnum<class "PDF Report Class.lvclass">, "error out"=w144:errorcluster)  [unwired: 9 in]
          }
        }
      }
      frame 3 {
        w145 = T11 {"Name"="Microsoft JhengHei UI", "Size"=15.0, "Color"=16711680, "Style"={"Bold"=FALSE, "Italic"=FALSE, "Underline"=FALSE, "Strikeout"=FALSE}, "Type"={"Type&direction"=enum."ASCII", "Embedded"=FALSE, "Encoding"="Identity-H"}} ("Font")
        w150 = Chapter."Chapter - level 1" ("Chapter or section")
        w188 = sgl 60.0  # Scale (%)
        w193 = sgl 60.0  # Scale (%)
        w197 = sgl 60.0  # Scale (%)
        # "创建分页"
        # "段落和链接.vi"
        # "添加图片和图片标签"
        # "自定义一个标题字体颜色和大小等。"
        # "C) Chapters 1 and 2"
        n53 = call <userlib>:"Append Chapter bookmark.vi"("PDF Report"=w205, "Chapter or section"=w150, "Title"="Text C1", "TriggerNewPage (Chapter)"=TRUE, "error in (no error)"=w158, "Font"=w145) -> ("PDF Report duplicate"=w160:refnum<class "PDF Report Class.lvclass">, "error out"=w159:errorcluster)  [unwired: 8 in]
        n54 = call-poly <userlib>:"Append Text polymorphic.vi"("PDF Report"=w160, "Text [ ]"="Texte C2 [ ]", "error in (no error)"=w159) -> ("PDF Report duplicate"=w156:refnum<class "PDF Report Class.lvclass">, "error out"=w155:errorcluster)  [unwired: 1 in, 10 out]
        n55 = call <userlib>:"Append Chapter bookmark.vi"("PDF Report"=w156, "Chapter or section"=w150, "Title"="Text C3", "TriggerNewPage (Chapter)"=TRUE, "error in (no error)"=w155, "Font"=w145) -> ("PDF Report duplicate"=w151:refnum<class "PDF Report Class.lvclass">, "error out"=w154:errorcluster)  [unwired: 8 in]
        n56 = call-poly <userlib>:"Append Text polymorphic.vi"("PDF Report"=w151, "Text [ ]"="Texte C4 [ ]", "error in (no error)"=w154) -> ("PDF Report duplicate"=w152:refnum<class "PDF Report Class.lvclass">, "error out"=w153:errorcluster)  [unwired: 1 in, 10 out]
        n57 = Unbundle("Image C1") -> ("Nom"=w180:path, "Légende"=w179:string)
        n58 = call <userlib>:"Update path.vi"("Path IN"=w180) -> ("Path OUT"=w181:path)  [unwired: 1 in, 2 out]
        n59 = call <userlib>:"Append Image File.vi"("PDF Report IN"=w152, "Image path"=w181, "error in (no error)"=w153, "Caption"=w179) -> ("PDF Report OUT"=w174:refnum<class "PDF Report Class.lvclass">, "error out"=w177:errorcluster)  [unwired: 3 in, 7 out]
        n60 = Unbundle("Image C2") -> ("Nom"=w195:path, "Légende"=w198:string)
        n61 = call-poly <userlib>:"Append Text polymorphic.vi"("PDF Report"=w174, "Text"="Text C5", "error in (no error)"=w177) -> ("PDF Report duplicate"=w175:refnum<class "PDF Report Class.lvclass">, "error out"=w176:errorcluster)  [unwired: 5 in, 6 out]
        n62 = call <userlib>:"Update path.vi"("Path IN"=w195) -> ("Path OUT"=w194:path)  [unwired: 1 in, 2 out]
        n63 = call <userlib>:"Append Image File.vi"("PDF Report IN"=w175, "Scale (%)"=w197, "Image path"=w194, "error in (no error)"=w176, "Caption"=w198) -> ("PDF Report OUT"=w170:refnum<class "PDF Report Class.lvclass">, "error out"=w171:errorcluster)  [unwired: 2 in, 7 out]
        n64 = Unbundle("Image C3") -> ("Nom"=w192:path, "Légende"=w189:string)
        n65 = call-poly <userlib>:"Append Text polymorphic.vi"("PDF Report"=w170, "Text"="Text C7", "error in (no error)"=w171) -> ("PDF Report duplicate"=w168:refnum<class "PDF Report Class.lvclass">, "error out"=w169:errorcluster)  [unwired: 5 in, 6 out]
        n66 = call <userlib>:"Update path.vi"("Path IN"=w192) -> ("Path OUT"=w190:path)  [unwired: 1 in, 2 out]
        n67 = call <userlib>:"Append Image File.vi"("PDF Report IN"=w168, "Scale (%)"=w193, "Image path"=w190, "error in (no error)"=w169, "Caption"=w189) -> ("PDF Report OUT"=w161:refnum<class "PDF Report Class.lvclass">, "error out"=w162:errorcluster)  [unwired: 2 in, 7 out]
        n68 = call <userlib>:"Append New Page.vi"("PDF Report"=w161, "error in (no error)"=w162) -> ("PDF Report duplicate"=w164:refnum<class "PDF Report Class.lvclass">, "error OUT"=w163:errorcluster)  [unwired: 12 out]
        n69 = Unbundle("Image C4") -> ("Nom"=w184:path, "Légende"=w182:string)
        n70 = call-poly <userlib>:"Append Text polymorphic.vi"("PDF Report"=w164, "Text"="Text C6", "error in (no error)"=w163) -> ("PDF Report duplicate"=w165:refnum<class "PDF Report Class.lvclass">, "error out"=w166:errorcluster)  [unwired: 5 in, 6 out]
        n71 = call <userlib>:"Update path.vi"("Path IN"=w184) -> ("Path OUT"=w183:path)  [unwired: 1 in, 2 out]
        n72 = call <userlib>:"Append Image File.vi"("PDF Report IN"=w165, "Scale (%)"=w188, "Image path"=w183, "error in (no error)"=w166, "Caption"=w182) -> ("PDF Report OUT"=w187:refnum<class "PDF Report Class.lvclass">, "error out"=w186:errorcluster)  [unwired: 2 in, 7 out]
        n73 = call-poly <userlib>:"Append Text polymorphic.vi"("PDF Report"=w187, "Text"="Text C8", "error in (no error)"=w186) -> ("PDF Report duplicate"=w199:refnum<class "PDF Report Class.lvclass">, "error out"=w200:errorcluster)  [unwired: 5 in, 6 out]
        n74 = call <userlib>:"Append New Page.vi"("PDF Report"=w199, "error in (no error)"=w200) -> ("PDF Report duplicate"=w204:refnum<class "PDF Report Class.lvclass">, "error OUT"=w203:errorcluster)  [unwired: 12 out]
      }
      frame 4 {
        w206 = T11 {"Name"="STSONG", "Size"=-1.0, "Color"=0, "Style"={"Bold"=TRUE, "Italic"=FALSE, "Underline"=FALSE, "Strikeout"=FALSE}, "Type"={"Type&direction"=enum."Select", "Embedded"=FALSE, "Encoding"=""}} ("Font")
        w255 = sgl 48.0  # Scale (%)
        # "D et E) Chapters 3 and 4 and beginning of F"
        n75 = call <userlib>:"Append Chapter bookmark.vi"("PDF Report"=w244, "Chapter or section"=Chapter."Chapter - level 1", "Title"="Text D1", "error in (no error)"=w243, "Font"=w206) -> ("PDF Report duplicate"=w245:refnum<class "PDF Report Class.lvclass">, "error out"=w242:errorcluster)  [unwired: 9 in]
        n76 = Unbundle("Image D1") -> ("Nom"=w252:path, "Légende"=w257:string)
        n77 = call-poly <userlib>:"Append Text polymorphic.vi"("PDF Report"=w245, "Text [ ]"="Texte D2 [ ]", "error in (no error)"=w242) -> ("PDF Report duplicate"=w263:refnum<class "PDF Report Class.lvclass">, "error out"=w262:errorcluster)  [unwired: 1 in, 10 out]
        n78 = call <userlib>:"Update path.vi"("Path IN"=w252) -> ("Path OUT"=w253:path)  [unwired: 1 in, 2 out]
        n79 = call <userlib>:"Append Image File.vi"("PDF Report IN"=w263, "Image path"=w253, "error in (no error)"=w262, "Caption"=w257) -> ("PDF Report OUT"=w246:refnum<class "PDF Report Class.lvclass">, "error out"=w249:errorcluster)  [unwired: 3 in, 7 out]
        n80 = call <userlib>:"Append Chapter bookmark.vi"("PDF Report"=w246, "Chapter or section"=Chapter."Chapter - level 1", "Title"="Text E1", "error in (no error)"=w249, "Font"=w206) -> ("PDF Report duplicate"=w247:refnum<class "PDF Report Class.lvclass">, "error out"=w248:errorcluster)  [unwired: 9 in]
        n81 = call-poly <userlib>:"Append Text polymorphic.vi"("PDF Report"=w247, "Text [ ]"="Texte E2 [ ]", "error in (no error)"=w248) -> ("PDF Report duplicate"=w260:refnum<class "PDF Report Class.lvclass">, "error out"=w259:errorcluster)  [unwired: 2 in, 9 out]
        n82 = Unbundle("Image E1") -> ("Nom"=w251:path, "Légende"=w256:string)
        n83 = call <userlib>:"Update path.vi"("Path IN"=w251) -> ("Path OUT"=w250:path)  [unwired: 1 in, 2 out]
        n84 = call <userlib>:"Append Image File.vi"("PDF Report IN"=w260, "Scale (%)"=w255, "Image path"=w250, "error in (no error)"=w259, "Caption"=w256) -> ("PDF Report OUT"=w234:refnum<class "PDF Report Class.lvclass">, "error out"=w235:errorcluster)  [unwired: 2 in, 7 out]
        n85 = call <userlib>:"Append Chapter bookmark.vi"("PDF Report"=w234, "Chapter or section"=Chapter."Chapter - level 1", "Title"="Text F1", "error in (no error)"=w235, "Font"=w206, "Title properties"=T7 {" Aligment"=enum."LEFT", "Line spacing"=enum."1.5"}) -> ("PDF Report duplicate"=w233:refnum<class "PDF Report Class.lvclass">, "error out"=w232:errorcluster)  [unwired: 8 in]
        n86 = call <userlib>:"Append Chapter bookmark.vi"("PDF Report"=w233, "Chapter or section"=Chapter."Chapter - level 2", "Title"="Text F2", "error in (no error)"=w232, "Font"=w206) -> ("PDF Report duplicate"=w212:refnum<class "PDF Report Class.lvclass">, "error out"=w211:errorcluster)  [unwired: 9 in]
        n87 = call-poly <userlib>:"Append Text polymorphic.vi"("PDF Report"=w212, "Text [ ]"="Texte F3 [ ]", "error in (no error)"=w211) -> ("PDF Report duplicate"=w218:refnum<class "PDF Report Class.lvclass">, "error out"=w217:errorcluster)  [unwired: 2 in, 9 out]
        n88 = call <userlib>:"Update path [ ].vi"("Image to Add IN [ ]"="Image to Add [ ]") -> ("Image to Add OUT [ ]"=w223:T44)  [unwired: 1 in, 2 out]
        n89 = call <userlib>:"Create Table.vi"("PDF Report IN"=w218, "Table columnWidth [ ]"="Table columnWidth [ ] - Table 1", "Column Headers 2D [ ]"="Column Headers 2D [ ] - Table 1", "Text Data 2D [ ]"="Text Data 2D [ ] - Table 1", "error in (no error)"=w217, "Image to Add [ ]"=w223) -> ("PDF Report duplicate"=w226:refnum<class "PDF Report Class.lvclass">, "PDF Table"=w224:refnum<class "Pdfp Table Class.lvclass">, "error out"=w225:errorcluster)  [unwired: 7 in]
        n90 = call <userlib>:"Append Table.vi"("PDF Report IN"=w226, "Predefined Borders"="Predefined Borders Table 1", "Table properties"="Table properties 1)", "PDF Table"=w224, "Caption"="Caption 1", "error in (no error)"=w225, "Row Header format"="Datas properties 1", "Custom Table Borders"="Custom Table Borders 1") -> ("PDF Report OUT"=w209:refnum<class "PDF Report Class.lvclass">, "error out"=w210:errorcluster)  [unwired: 3 in, 3 out]
        n91 = call <userlib>:"Append New Page.vi"("PDF Report"=w209, "error in (no error)"=w210) -> ("PDF Report duplicate"=w208:refnum<class "PDF Report Class.lvclass">, "error OUT"=w207:errorcluster)  [unwired: 12 out]
      }
      frame 5 {
        w277 = sgl 40.0  # Scale (%)
        w289 = sgl 50.0  # Scale (%)
        w303 = sgl 55.0  # Scale (%)
        # "F) Chapter 5, section 5.1 - Text palette"
        n92 = Unbundle("Image F1") -> ("Nom"=w272:path, "Légende"=w271:string)
        n93 = call-poly <userlib>:"Append Text polymorphic.vi"("PDF Report"=w267, "Text"="Text F4", "error in (no error)"=w266) -> ("PDF Report duplicate"=w276:refnum<class "PDF Report Class.lvclass">, "error out"=w275:errorcluster)  [unwired: 5 in, 6 out]
        n94 = call <userlib>:"Update path.vi"("Path IN"=w272) -> ("Path OUT"=w273:path)  [unwired: 1 in, 2 out]
        n95 = call <userlib>:"Append Image File.vi"("PDF Report IN"=w276, "Scale (%)"=w277, "Image path"=w273, "error in (no error)"=w275, "Caption"=w271) -> ("PDF Report OUT"=w268:refnum<class "PDF Report Class.lvclass">, "error out"=w269:errorcluster)  [unwired: 2 in, 7 out]
        n96 = Unbundle("Image F2") -> ("Nom"=w294:path, "Légende"=w295:string)
        n97 = Unbundle("Image F3") -> ("Nom"=w283:path, "Légende"=w286:string)
        n98 = call-poly <userlib>:"Append Text polymorphic.vi"("PDF Report"=w268, "Text"="Text F5", "error in (no error)"=w269) -> ("PDF Report duplicate"=w290:refnum<class "PDF Report Class.lvclass">, "error out"=w291:errorcluster)  [unwired: 5 in, 6 out]
        n99 = call <userlib>:"Update path.vi"("Path IN"=w294) -> ("Path OUT"=w293:path)  [unwired: 1 in, 2 out]
        n100 = call <userlib>:"Update path.vi"("Path IN"=w283) -> ("Path OUT"=w282:path)  [unwired: 1 in, 2 out]
        n101 = call <userlib>:"Append Image File.vi"("PDF Report IN"=w290, "Scale (%)"=w289, "Image path"=w293, "error in (no error)"=w291, "Caption"=w295) -> ("PDF Report OUT"=w281:refnum<class "PDF Report Class.lvclass">, "error out"=w280:errorcluster)  [unwired: 2 in, 7 out]
        n102 = call-poly <userlib>:"Append Text polymorphic.vi"("PDF Report"=w281, "Text"="Text F6", "error in (no error)"=w280) -> ("PDF Report duplicate"=w284:refnum<class "PDF Report Class.lvclass">, "error out"=w285:errorcluster)  [unwired: 5 in, 6 out]
        n103 = Unbundle("Image F4") -> ("Nom"=w307:path, "Légende"=w304:string)
        n104 = call <userlib>:"Update path.vi"("Path IN"=w307) -> ("Path OUT"=w305:path)  [unwired: 1 in, 2 out]
        n105 = call <userlib>:"Append Image File.vi"("PDF Report IN"=w284, "Scale (%)"=sgl 60.0, "Image path"=w282, "error in (no error)"=w285, "Caption"=w286) -> ("PDF Report OUT"=w278:refnum<class "PDF Report Class.lvclass">, "error out"=w279:errorcluster)  [unwired: 2 in, 7 out]
        n106 = call <userlib>:"Append Image File.vi"("PDF Report IN"=w278, "Scale (%)"=w303, "Image path"=w305, "error in (no error)"=w279, "Caption"=w304) -> ("PDF Report OUT"=w308:refnum<class "PDF Report Class.lvclass">, "error out"=w309:errorcluster)  [unwired: 2 in, 7 out]
        n107 = local read "Image to Add [ ]"() -> (w316:T44)
        n108 = call-poly <userlib>:"Append Text polymorphic.vi"("PDF Report"=w308, "Text"="Text F7", "error in (no error)"=w309) -> ("PDF Report duplicate"=w298:refnum<class "PDF Report Class.lvclass">, "error out"=w297:errorcluster)  [unwired: 5 in, 6 out]
        n109 = call <userlib>:"Update path [ ].vi"("Image to Add IN [ ]"=w316) -> ("Image to Add OUT [ ]"=w315:T44)  [unwired: 1 in, 2 out]
        n110 = call-poly <userlib>:"Append Text polymorphic.vi"("PDF Report"=w298, "Text [ ]"="Text F8 [ ]", "error in (no error)"=w297, "Image to Add [ ]"=w315) -> ("PDF Report duplicate"=w299:refnum<class "PDF Report Class.lvclass">, "error out"=w302:errorcluster)  [unwired: 10 out]
        n111 = call <userlib>:"Set Page Size.vi"("PDF Report IN"=w299, "Page setup"=T2 {"Page Size"=1, "Orientation"=enum."Landscape", "Custom Size"={"Width"=0.0, "Height"=0.0}, "Margins"={"Left"=1.0, "Right"=1.0, "Top"=1.0, "Bottom"=1.0}} ("Page seup"), "error in (no error)"=w302) -> ("PDF Report OUT"=w300:refnum<class "PDF Report Class.lvclass">, "error OUT"=w301:errorcluster)  [unwired: 11 out]
        n112 = Unbundle("Image F5") -> ("Nom"=w313:path, "Légende"=w318:string)
        n113 = call <userlib>:"Update path.vi"("Path IN"=w313) -> ("Path OUT"=w312:path)  [unwired: 1 in, 2 out]
        n114 = call <userlib>:"Append Image File.vi"("PDF Report IN"=w300, "Image path"=w312, "error in (no error)"=w301, "Caption"=w318) -> ("PDF Report OUT"=w310:refnum<class "PDF Report Class.lvclass">, "error out"=w311:errorcluster)  [unwired: 3 in, 7 out]
        n115 = call <userlib>:"Set Page Size.vi"("PDF Report IN"=w310, "Page setup"=T2 {"Page Size"=1, "Orientation"=enum."Portrait", "Custom Size"={"Width"=0.0, "Height"=0.0}, "Margins"={"Left"=1.0, "Right"=1.0, "Top"=1.0, "Bottom"=1.0}} ("Page seup"), "error in (no error)"=w311) -> ("PDF Report OUT"=w323:refnum<class "PDF Report Class.lvclass">, "error OUT"=w322:errorcluster)  [unwired: 11 out]
      }
      frame 6 {
        w356 = sgl 55.0  # Scale (%)
        # "这个时把vi 前面版写入pdf"
        # "Append block diagram\nimage"
        # "Append front panel\nimage"
        # "G) Chapter 5, section 5.2 -  Image palette"
        n116 = call <userlib>:"Append Chapter bookmark.vi"("PDF Report"=w325, "Chapter or section"=Chapter."Chapter - level 2", "Title"="Text G1", "error in (no error)"=w324) -> ("PDF Report duplicate"=w326:refnum<class "PDF Report Class.lvclass">, "error out"=w327:errorcluster)  [unwired: 10 in]
        n117 = call-poly <userlib>:"Append Text polymorphic.vi"("PDF Report"=w326, "Text [ ]"="Texte G2 [ ]", "error in (no error)"=w327) -> ("PDF Report duplicate"=w343:refnum<class "PDF Report Class.lvclass">, "error out"=w342:errorcluster)  [unwired: 2 in, 9 out]
        n118 = Unbundle("Image G1") -> ("Nom"=w363:path, "Légende"=w357:string)
        n119 = call <userlib>:"Update path.vi"("Path IN"=w363) -> ("Path OUT"=w364:path)  [unwired: 1 in, 2 out]
        n120 = call <userlib>:"Append Image File.vi"("PDF Report IN"=w343, "Scale (%)"=w356, "Image path"=w364, "error in (no error)"=w342, "Caption"=w357) -> ("PDF Report OUT"=w344:refnum<class "PDF Report Class.lvclass">, "error out"=w345:errorcluster)  [unwired: 2 in, 7 out]
        n121 = Unbundle By Name("Cluster of images controls") -> ("Border"=w352:T39, "Scale (%)"=w353:sgl, "Position"=w355:T37)
        n122 = call-poly <userlib>:"Append Text polymorphic.vi"("PDF Report"=w344, "Text [ ]"="Texte G3 [ ]", "error in (no error)"=w345) -> ("PDF Report duplicate"=w350:refnum<class "PDF Report Class.lvclass">, "error out"=w346:errorcluster)  [unwired: 2 in, 9 out]
        n123 = control-ref of="Cluster of images controls"() -> (w354:refnum<vi>)
        n124 = call <userlib>:"Append Control Image.vi"("PDF Report IN"=w350, "Scale (%)"=w353, "Border"=w352, "Ctrl reference"=w354, "error in (no error)"=w346, "Position and indentation"=w355) -> ("PDF Report OUT"=w347:refnum<class "PDF Report Class.lvclass">, "error out"=w348:errorcluster)  [unwired: 1 in, 7 out]
        n125 = call-poly <userlib>:"Append Text polymorphic.vi"("PDF Report"=w347, "Text"="Text G4", "error in (no error)"=w348) -> ("PDF Report duplicate"=w362:refnum<class "PDF Report Class.lvclass">, "error out"=w361:errorcluster)  [unwired: 5 in, 6 out]
        n126 = call <userlib>:"Set Page Size.vi"("PDF Report IN"=w362, "Page setup"=T2 {"Page Size"=1, "Orientation"=enum."Landscape", "Custom Size"={"Width"=0.0, "Height"=0.0}, "Margins"={"Left"=1.0, "Right"=1.0, "Top"=1.0, "Bottom"=1.0}} ("Page seup"), "error in (no error)"=w361) -> ("PDF Report OUT"=w366:refnum<class "PDF Report Class.lvclass">, "error OUT"=w365:errorcluster)  [unwired: 11 out]
        n127 = control-ref of="This VI"() -> (w335:refnum<vi>)
        n128 = call <userlib>:"Append Front Panel Image.vi"("PDF Report IN"=w366, "VI reference"=w335, "error in (no error)"=w365, "Caption"="Image G2") -> ("PDF Report OUT"=w336:refnum<class "PDF Report Class.lvclass">, "error out"=w337:errorcluster)  [unwired: 4 in, 6 out]
        n129 = case shown="真" "Add block diagram" {
          tunnel: w336 -> [w368 w375]
          tunnel: w337 -> [w367 w374]
          tunnel: [w367 w371] -> w332
          tunnel: [w368 w370] -> w333
          tunnel: w335 -> [_ w373]
          tunnel: "Image G3" -> [_ w372]
          frame False {
          }
          frame True {
            w369 = T67 {"Maximum Width"=2500, "Maximum Height"=2500}  # Max Image size
            n130 = call <userlib>:"Append Block Diagram Image.vi"("PDF Report IN"=w375, "Image size"=w369, "VI reference"=w373, "error in (no error)"=w374, "Caption"=w372) -> ("PDF Report OUT"=w370:refnum<class "PDF Report Class.lvclass">, "error out"=w371:errorcluster)  [unwired: 9 in]
          }
        }
        n131 = call <userlib>:"Set Page Size.vi"("PDF Report IN"=w333, "Page setup"=T2 {"Page Size"=1, "Orientation"=enum."Portrait", "Custom Size"={"Width"=0.0, "Height"=0.0}, "Margins"={"Left"=1.0, "Right"=1.0, "Top"=1.0, "Bottom"=1.0}} ("Page seup"), "error in (no error)"=w332) -> ("PDF Report OUT"=w330:refnum<class "PDF Report Class.lvclass">, "error OUT"=w331:errorcluster)  [unwired: 11 out]
      }
      frame 7 {
        w404 = sgl 45.0  # Scale (%)
        w411 = sgl 28.0  # Scale (%)
        w412 = sgl 55.0  # Scale (%)
        w413 = sgl 45.0  # Scale (%)
        # "H) Chapter 5, section 5.3 - Table palette"
        n132 = call <userlib>:"Append Chapter bookmark.vi"("PDF Report"=w386, "Chapter or section"=Chapter."Chapter - level 2", "Title"="Text H1", "error in (no error)"=w387) -> ("PDF Report duplicate"=w389:refnum<class "PDF Report Class.lvclass">, "error out"=w388:errorcluster)  [unwired: 10 in]
        n133 = call-poly <userlib>:"Append Text polymorphic.vi"("PDF Report"=w389, "Text [ ]"="Texte H2 [ ]", "error in (no error)"=w388) -> ("PDF Report duplicate"=w421:refnum<class "PDF Report Class.lvclass">, "error out"=w422:errorcluster)  [unwired: 2 in, 9 out]
        n134 = Unbundle("Image H1") -> ("Nom"=w427:path, "Légende"=w424:string)
        n135 = call <userlib>:"Update path.vi"("Path IN"=w427) -> ("Path OUT"=w430:path)  [unwired: 1 in, 2 out]
        n136 = Unbundle("Image H2") -> ("Nom"=w403:path, "Légende"=w401:string)
        n137 = call <userlib>:"Update path.vi"("Path IN"=w403) -> ("Path OUT"=w402:path)  [unwired: 1 in, 2 out]
        n138 = call <userlib>:"Append Image File.vi"("PDF Report IN"=w421, "Scale (%)"=w412, "Image path"=w430, "error in (no error)"=w422, "Caption"=w424) -> ("PDF Report OUT"=w407:refnum<class "PDF Report Class.lvclass">, "error out"=w406:errorcluster)  [unwired: 2 in, 7 out]
        n139 = Unbundle("Image H3") -> ("Nom"=w410:path, "Légende"=w409:string)
        n140 = call <userlib>:"Append LF.vi"("PDF Report IN"=w407, "error in (no error)"=w406) -> ("PDF Report duplicate"=w399:refnum<class "PDF Report Class.lvclass">, "error out"=w398:errorcluster)  [unwired: 12 in]
        n141 = call <userlib>:"Update path.vi"("Path IN"=w410) -> ("Path OUT"=w405:path)  [unwired: 1 in, 2 out]
        n142 = call <userlib>:"Append Image File.vi"("PDF Report IN"=w399, "Image path"=w402, "error in (no error)"=w398, "Caption"=w401) -> ("PDF Report OUT"=w396:refnum<class "PDF Report Class.lvclass">, "error out"=w397:errorcluster)  [unwired: 3 in, 7 out]
        n143 = call <userlib>:"Append Image File.vi"("PDF Report IN"=w396, "Scale (%)"=w404, "Image path"=w405, "error in (no error)"=w397, "Caption"=w409) -> ("PDF Report OUT"=w392:refnum<class "PDF Report Class.lvclass">, "error out"=w393:errorcluster)  [unwired: 2 in, 7 out]
        n144 = call-poly <userlib>:"Append Text polymorphic.vi"("PDF Report"=w392, "Text"="Text H3", "error in (no error)"=w393) -> ("PDF Report duplicate"=w395:refnum<class "PDF Report Class.lvclass">, "error out"=w394:errorcluster)  [unwired: 5 in, 6 out]
        n145 = call-poly <userlib>:"Append Text polymorphic.vi"("PDF Report"=w395, "Text [ ]"="Texte H4 [ ]", "error in (no error)"=w394) -> ("PDF Report duplicate"=w379:refnum<class "PDF Report Class.lvclass">, "error out"=w378:errorcluster)  [unwired: 1 in, 10 out]
        n146 = Unbundle("Image H4") -> ("Nom"=w381:path, "Légende"=w382:string)
        n147 = call <userlib>:"Update path.vi"("Path IN"=w381) -> ("Path OUT"=w380:path)  [unwired: 1 in, 2 out]
        n148 = call <userlib>:"Append Image File.vi"("PDF Report IN"=w379, "Image path"=w380, "error in (no error)"=w378, "Caption"=w382) -> ("PDF Report OUT"=w376:refnum<class "PDF Report Class.lvclass">, "error out"=w377:errorcluster)  [unwired: 3 in, 7 out]
        n149 = Unbundle("Image H5") -> ("Nom"=w428:path, "Légende"=w425:string)
        n150 = call <userlib>:"Update path.vi"("Path IN"=w428) -> ("Path OUT"=w429:path)  [unwired: 1 in, 2 out]
        n151 = call <userlib>:"Append Image File.vi"("PDF Report IN"=w376, "Scale (%)"=w413, "Image path"=w429, "error in (no error)"=w377, "Caption"=w425) -> ("PDF Report OUT"=w418:refnum<class "PDF Report Class.lvclass">, "error out"=w417:errorcluster)  [unwired: 2 in, 7 out]
        n152 = Unbundle("Image H6") -> ("Nom"=w434:path, "Légende"=w432:string)
        n153 = call-poly <userlib>:"Append Text polymorphic.vi"("PDF Report"=w418, "Text"="Text H5", "error in (no error)"=w417) -> ("PDF Report duplicate"=w414:refnum<class "PDF Report Class.lvclass">, "error out"=w415:errorcluster)  [unwired: 5 in, 6 out]
        n154 = call <userlib>:"Update path.vi"("Path IN"=w434) -> ("Path OUT"=w435:path)  [unwired: 1 in, 2 out]
        n155 = call <userlib>:"Append Image File.vi"("PDF Report IN"=w414, "Scale (%)"=w411, "Image path"=w435, "error in (no error)"=w415, "Caption"=w432) -> ("PDF Report OUT"=w384:refnum<class "PDF Report Class.lvclass">, "error out"=w385:errorcluster)  [unwired: 2 in, 7 out]
      }
      frame 8 {
        w444 = sgl 50.0  # Scale (%)
        w454 = sgl 50.0  # Scale (%)
        w480 = sgl 60.0  # Scale (%)
        w484 = sgl 60.0  # Scale (%)
        # "H) Chapter 5, section 5.3 - Table palette"
        n156 = Unbundle("Image H7") -> ("Nom"=w437:path, "Légende"=w457:string)
        n157 = call <userlib>:"Update path.vi"("Path IN"=w437) -> ("Path OUT"=w436:path)  [unwired: 1 in, 2 out]
        n158 = call-poly <userlib>:"Append Text polymorphic.vi"("PDF Report"=w439, "Text"="Text H6", "error in (no error)"=w438) -> ("PDF Report duplicate"=w456:refnum<class "PDF Report Class.lvclass">, "error out"=w455:errorcluster)  [unwired: 5 in, 6 out]
        n159 = local read "Image to Add [ ]"() -> (w448:T44)
        n160 = call <userlib>:"Append Image File.vi"("PDF Report IN"=w456, "Scale (%)"=w454, "Image path"=w436, "error in (no error)"=w455, "Caption"=w457) -> ("PDF Report OUT"=w443:refnum<class "PDF Report Class.lvclass">, "error out"=w442:errorcluster)  [unwired: 2 in, 7 out]
        n161 = call <userlib>:"Update path [ ].vi"("Image to Add IN [ ]"=w448) -> ("Image to Add OUT [ ]"=w449:T44)  [unwired: 1 in, 2 out]
        n162 = call-poly <userlib>:"Append Text polymorphic.vi"("PDF Report"=w443, "Text [ ]"="Text H7 [ ]", "error in (no error)"=w442, "Image to Add [ ]"=w449) -> ("PDF Report duplicate"=w445:refnum<class "PDF Report Class.lvclass">, "error out"=w446:errorcluster)  [unwired: 10 out]
        n163 = Unbundle("Image H8") -> ("Nom"=w450:path, "Légende"=w452:string)
        n164 = call <userlib>:"Update path.vi"("Path IN"=w450) -> ("Path OUT"=w451:path)  [unwired: 1 in, 2 out]
        n165 = call <userlib>:"Append Image File.vi"("PDF Report IN"=w445, "Scale (%)"=w444, "Image path"=w451, "error in (no error)"=w446, "Caption"=w452) -> ("PDF Report OUT"=w440:refnum<class "PDF Report Class.lvclass">, "error out"=w441:errorcluster)  [unwired: 2 in, 7 out]
        n166 = call-poly <userlib>:"Append Text polymorphic.vi"("PDF Report"=w440, "Text"="Text H8", "error in (no error)"=w441) -> ("PDF Report duplicate"=w464:refnum<class "PDF Report Class.lvclass">, "error out"=w463:errorcluster)  [unwired: 5 in, 6 out]
        n167 = Unbundle("Image H9") -> ("Nom"=w477:path, "Légende"=w479:string)
        n168 = call <userlib>:"Update path.vi"("Path IN"=w477) -> ("Path OUT"=w478:path)  [unwired: 1 in, 2 out]
        n169 = Unbundle("Image H10") -> ("Nom"=w472:path, "Légende"=w474:string)
        n170 = call <userlib>:"Append Image File.vi"("PDF Report IN"=w464, "Scale (%)"=w480, "Image path"=w478, "error in (no error)"=w463, "Caption"=w479) -> ("PDF Report OUT"=w469:refnum<class "PDF Report Class.lvclass">, "error out"=w470:errorcluster)  [unwired: 2 in, 7 out]
        n171 = call <userlib>:"Update path.vi"("Path IN"=w472) -> ("Path OUT"=w473:path)  [unwired: 1 in, 2 out]
        n172 = call <userlib>:"Append Image File.vi"("PDF Report IN"=w469, "Image path"=w473, "error in (no error)"=w470, "Caption"=w474) -> ("PDF Report OUT"=w468:refnum<class "PDF Report Class.lvclass">, "error out"=w461:errorcluster)  [unwired: 3 in, 7 out]
        n173 = Unbundle("Image H11") -> ("Nom"=w481:path, "Légende"=w483:string)
        n174 = call <userlib>:"Update path.vi"("Path IN"=w481) -> ("Path OUT"=w482:path)  [unwired: 1 in, 2 out]
        n175 = call <userlib>:"Append New Page.vi"("PDF Report"=w468, "error in (no error)"=w461) -> ("PDF Report duplicate"=w462:refnum<class "PDF Report Class.lvclass">, "error OUT"=w460:errorcluster)  [unwired: 12 in]
        n176 = call <userlib>:"Append Image File.vi"("PDF Report IN"=w462, "Scale (%)"=w484, "Image path"=w482, "error in (no error)"=w460, "Caption"=w483) -> ("PDF Report OUT"=w467:refnum<class "PDF Report Class.lvclass">, "error out"=w466:errorcluster)  [unwired: 2 in, 7 out]
      }
      frame 9 {
        # "H) Chapter 5, section 5.3 - Table palette"
        # "Table 4"
        # "Table 3"
        # "Table 2"
        n177 = call <userlib>:"Create Table.vi"("PDF Report IN"=w488, "Column Headers 2D [ ]"="Column Headers 2D [ ] - Tables 2 to 4", "Text Data 2D [ ]"="Text Data 2D [ ]  - Tables 2 to 4", "error in (no error)"=w487) -> ("PDF Report duplicate"=w513:refnum<class "PDF Report Class.lvclass">, "PDF Table"=w514:refnum<class "Pdfp Table Class.lvclass">, "error out"=w515:errorcluster)  [unwired: 9 in]
        n178 = call <userlib>:"Append Table.vi"("PDF Report IN"=w513, "Table properties"="Table properties  - Tables 2 to 4", "PDF Table"=w514, "Caption"="Caption - Table 2", "error in (no error)"=w515) -> ("PDF Report OUT"=w520:refnum<class "PDF Report Class.lvclass">, "error out"=w521:errorcluster)  [unwired: 7 in, 2 out]
        n179 = call <userlib>:"Create Table.vi"("PDF Report IN"=w520, "Table columnWidth [ ]"="Table columnWidth [ ]  - Tables 3 and 4", "Column Headers 2D [ ]"="Column Headers 2D [ ] - Tables 2 to 4", "Text Data 2D [ ]"="Text Data 2D [ ]  - Tables 2 to 4", "error in (no error)"=w521) -> ("PDF Report duplicate"=w519:refnum<class "PDF Report Class.lvclass">, "PDF Table"=w516:refnum<class "Pdfp Table Class.lvclass">, "error out"=w518:errorcluster)  [unwired: 8 in]
        n180 = call <userlib>:"Append Table.vi"("PDF Report IN"=w519, "Table properties"="Table properties  - Tables 2 to 4", "PDF Table"=w516, "Caption"="Caption - Table 3", "error in (no error)"=w518) -> ("PDF Report OUT"=w523:refnum<class "PDF Report Class.lvclass">, "error out"=w522:errorcluster)  [unwired: 7 in, 2 out]
        n181 = call <userlib>:"Append New Page.vi"("PDF Report"=w523, "error in (no error)"=w522) -> ("PDF Report duplicate"=w498:refnum<class "PDF Report Class.lvclass">, "error OUT"=w497:errorcluster)  [unwired: 12 out]
        n182 = Unbundle("Image H12") -> ("Nom"=w505:path, "Légende"=w510:string)
        n183 = call <userlib>:"Update path.vi"("Path IN"=w505) -> ("Path OUT"=w509:path)  [unwired: 1 in, 2 out]
        n184 = call <userlib>:"Append Image File.vi"("PDF Report IN"=w498, "Scale (%)"=sgl 60.0, "Image path"=w509, "error in (no error)"=w497, "Caption"=w510) -> ("PDF Report OUT"=w508:refnum<class "PDF Report Class.lvclass">, "error out"=w511:errorcluster)  [unwired: 2 in, 7 out]
        n185 = call <userlib>:"Create Table.vi"("PDF Report IN"=w508, "Table columnWidth [ ]"="Table columnWidth [ ]  - Tables 3 and 4", "Column Headers 2D [ ]"="Column Headers 2D [ ] - Tables 2 to 4", "Text Data 2D [ ]"="Text Data 2D [ ]  - Tables 2 to 4", "error in (no error)"=w511) -> ("PDF Report duplicate"=w501:refnum<class "PDF Report Class.lvclass">, "PDF Table"=w500:refnum<class "Pdfp Table Class.lvclass">, "error out"=w499:errorcluster)  [unwired: 8 in]
        n186 = call <userlib>:"Append Table.vi"("PDF Report IN"=w501, "Column Header format"="Column Header format - Table 4", "Predefined Borders"="Predefined Borders - Table 4", "Row background color"="Row background color - Table 4", "Table properties"="Table properties  - Tables 2 to 4", "PDF Table"=w500, "Caption"="Caption - Table 4", "error in (no error)"=w499, "Datas format"="Datas format - Table 4") -> ("PDF Report OUT"=w489:refnum<class "PDF Report Class.lvclass">, "error out"=w490:errorcluster)  [unwired: 3 in, 2 out]
        n187 = call <userlib>:"Append New Page.vi"("PDF Report"=w489, "error in (no error)"=w490) -> ("PDF Report duplicate"=w486:refnum<class "PDF Report Class.lvclass">, "error OUT"=w485:errorcluster)  [unwired: 12 out]
      }
      frame 10 {
        # "H) Chapter 5, section 5.3 - Table palette"
        # "Table 5"
        n188 = Unbundle("Image H13") -> ("Nom"=w528:path, "Légende"=w532:string)
        n189 = call <userlib>:"Update path.vi"("Path IN"=w528) -> ("Path OUT"=w531:path)  [unwired: 1 in, 2 out]
        n190 = call <userlib>:"Append Image File.vi"("PDF Report IN"=w524, "Scale (%)"=sgl 60.0, "Image path"=w531, "error in (no error)"=w525, "Caption"=w532) -> ("PDF Report OUT"=w526:refnum<class "PDF Report Class.lvclass">, "error out"=w527:errorcluster)  [unwired: 2 in, 7 out]
        n191 = call <userlib>:"Create Table.vi"("PDF Report IN"=w526, "Table columnWidth [ ]"="Table columnWidth [ ] - Table 5", "Column Headers 2D [ ]"="Column Headers 2D [ ] - Table 5", "Row Headers 1D [ ]"="Row Headers 1D [ ] - Table 5", "Text Data 2D [ ]"="Text Data 2D [ ] - Table 5", "error in (no error)"=w527) -> ("PDF Report duplicate"=w543:refnum<class "PDF Report Class.lvclass">, "PDF Table"=w540:refnum<class "Pdfp Table Class.lvclass">, "error out"=w544:errorcluster)  [unwired: 7 in]
        n192 = call <userlib>:"Append Customized Table.vi"("PDF Report IN"=w543, "Table properties"="Table properties - Table 5", "PDF Table"=w540, "Caption"="Caption - Table 5", "error in (no error)"=w544, "Row  [ ]"="Row  [ ] - Table 5") -> ("PDF Report OUT"=w534:refnum<class "PDF Report Class.lvclass">, "error out"=w533:errorcluster)  [unwired: 8 in]
        n193 = call <userlib>:"Append New Page.vi"("PDF Report"=w534, "error in (no error)"=w533) -> ("PDF Report duplicate"=w546:refnum<class "PDF Report Class.lvclass">, "error OUT"=w545:errorcluster)  [unwired: 12 out]
      }
      frame 11 {
        w570 = sgl 100.0  # Scale (%)
        w595 = sgl 48.0  # Scale (%)
        # "Table 6"
        # "I) Chapter 5, section 5.4 Document palette"
        n194 = call <userlib>:"Append Chapter bookmark.vi"("PDF Report"=w547, "Chapter or section"=Chapter."Chapter - level 2", "Title"="Text I1", "error in (no error)"=w548) -> ("PDF Report duplicate"=w550:refnum<class "PDF Report Class.lvclass">, "error out"=w549:errorcluster)  [unwired: 10 in]
        n195 = call-poly <userlib>:"Append Text polymorphic.vi"("PDF Report"=w550, "Text [ ]"="Texte I2 [ ]", "error in (no error)"=w549) -> ("PDF Report duplicate"=w585:refnum<class "PDF Report Class.lvclass">, "error out"=w586:errorcluster)  [unwired: 2 in, 9 out]
        n196 = Unbundle("Image I1") -> ("Nom"=w601:path, "Légende"=w597:string)
        n197 = call <userlib>:"Update path.vi"("Path IN"=w601) -> ("Path OUT"=w604:path)  [unwired: 1 in, 2 out]
        n198 = call <userlib>:"Append Image File.vi"("PDF Report IN"=w585, "Scale (%)"=w595, "Image path"=w604, "error in (no error)"=w586, "Caption"=w597) -> ("PDF Report OUT"=w588:refnum<class "PDF Report Class.lvclass">, "error out"=w589:errorcluster)  [unwired: 2 in, 7 out]
        n199 = call-poly <userlib>:"Append Text polymorphic.vi"("PDF Report"=w588, "Text [ ]"="Texte I3 [ ]", "error in (no error)"=w589) -> ("PDF Report duplicate"=w591:refnum<class "PDF Report Class.lvclass">, "error out"=w590:errorcluster)  [unwired: 2 in, 9 out]
        n200 = Unbundle("Image I2") -> ("Nom"=w602:path, "Légende"=w596:string)
        n201 = Unbundle("Image I3") -> ("Nom"=w603:path, "Légende"=w598:string)
        n202 = call <userlib>:"Update path.vi"("Path IN"=w602) -> ("Path OUT"=w605:path)  [unwired: 1 in, 2 out]
        n203 = call <userlib>:"Update path.vi"("Path IN"=w603) -> ("Path OUT"=w606:path)  [unwired: 1 in, 2 out]
        n204 = call <userlib>:"Append Image File.vi"("PDF Report IN"=w591, "Scale (%)"=w595, "Image path"=w605, "error in (no error)"=w590, "Caption"=w596) -> ("PDF Report OUT"=w583:refnum<class "PDF Report Class.lvclass">, "error out"=w584:errorcluster)  [unwired: 2 in, 7 out]
        n205 = call <userlib>:"Append Image File.vi"("PDF Report IN"=w583, "Scale (%)"=w595, "Image path"=w606, "error in (no error)"=w584, "Caption"=w598) -> ("PDF Report OUT"=w562:refnum<class "PDF Report Class.lvclass">, "error out"=w561:errorcluster)  [unwired: 2 in, 7 out]
        n206 = Unbundle("Image I4") -> ("Nom"=w572:path, "Légende"=w571:string)
        n207 = call <userlib>:"Update path.vi"("Path IN"=w572) -> ("Path OUT"=w573:path)  [unwired: 1 in, 2 out]
        n208 = call-poly <userlib>:"Append Text polymorphic.vi"("PDF Report"=w562, "Text"="Texte I4", "error in (no error)"=w561) -> ("PDF Report duplicate"=w567:refnum<class "PDF Report Class.lvclass">, "error out"=w568:errorcluster)  [unwired: 5 in, 6 out]
        n209 = call <userlib>:"Append Image File.vi"("PDF Report IN"=w567, "Scale (%)"=w570, "Image path"=w573, "error in (no error)"=w568, "Caption"=w571) -> ("PDF Report OUT"=w565:refnum<class "PDF Report Class.lvclass">, "error out"=w564:errorcluster)  [unwired: 2 in, 7 out]
        n210 = call-poly <userlib>:"Append Text polymorphic.vi"("PDF Report"=w565, "Text"="Texte I5", "error in (no error)"=w564) -> ("PDF Report duplicate"=w563:refnum<class "PDF Report Class.lvclass">, "error out"=w556:errorcluster)  [unwired: 5 in, 6 out]
        n211 = call <userlib>:"Append New Page.vi"("PDF Report"=w563, "error in (no error)"=w556) -> ("PDF Report duplicate"=w557:refnum<class "PDF Report Class.lvclass">, "error OUT"=w555:errorcluster)  [unwired: 12 in]
        n212 = call <userlib>:"Create Table.vi"("PDF Report IN"=w557, "Table columnWidth [ ]"="Table columnWidth [ ] - table 6", "Column Headers 2D [ ]"="Column Headers 2D [ ] - table 6", "Row Headers 1D [ ]"="Row Headers 1D [ ] - table 6", "Text Data 2D [ ]"="Text Data 2D [ ] - table 6", "error in (no error)"=w555) -> ("PDF Report duplicate"=w581:refnum<class "PDF Report Class.lvclass">, "PDF Table"=w577:refnum<class "Pdfp Table Class.lvclass">, "error out"=w582:errorcluster)  [unwired: 7 in]
        n213 = call <userlib>:"Append Customized Table.vi"("PDF Report IN"=w581, "PDF Table"=w577, "Caption"="Caption - table 6", "error in (no error)"=w582, "Row  [ ]"="Row  [ ] - table 6") -> ("PDF Report OUT"=w559:refnum<class "PDF Report Class.lvclass">, "error out"=w558:errorcluster)  [unwired: 9 in]
        n214 = call-poly <userlib>:"Append Text polymorphic.vi"("PDF Report"=w559, "Text [ ]"="Texte I6 [ ]", "error in (no error)"=w558) -> ("PDF Report duplicate"=w553:refnum<class "PDF Report Class.lvclass">, "error out"=w554:errorcluster)  [unwired: 2 in, 9 out]
      }
      frame 12 {
        w638 = sgl 50.0  # Scale (%)
        # "J) Chapter 5, section 5.5 - Header, Footer and Watermark palette"
        n215 = call <userlib>:"Append Chapter bookmark.vi"("PDF Report"=w607, "Chapter or section"=Chapter."Chapter - level 2", "Title"="Text J1", "error in (no error)"=w608) -> ("PDF Report duplicate"=w610:refnum<class "PDF Report Class.lvclass">, "error out"=w609:errorcluster)  [unwired: 10 in]
        n216 = call-poly <userlib>:"Append Text polymorphic.vi"("PDF Report"=w610, "Text [ ]"="Texte J2 [ ]", "error in (no error)"=w609) -> ("PDF Report duplicate"=w637:refnum<class "PDF Report Class.lvclass">, "error out"=w636:errorcluster)  [unwired: 2 in, 9 out]
        n217 = Unbundle("Image J1") -> ("Nom"=w647:path, "Légende"=w639:string)
        n218 = Unbundle("Image J2") -> ("Nom"=w646:path, "Légende"=w640:string)
        n219 = Unbundle("Image J3") -> ("Nom"=w664:path, "Légende"=w641:string)
        n220 = Unbundle("Image J4") -> ("Nom"=w648:path, "Légende"=w642:string)
        n221 = call <userlib>:"Update path.vi"("Path IN"=w647) -> ("Path OUT"=w649:path)  [unwired: 1 in, 2 out]
        n222 = call <userlib>:"Update path.vi"("Path IN"=w646) -> ("Path OUT"=w650:path)  [unwired: 1 in, 2 out]
        n223 = call <userlib>:"Update path.vi"("Path IN"=w664) -> ("Path OUT"=w665:path)  [unwired: 1 in, 2 out]
        n224 = call <userlib>:"Update path.vi"("Path IN"=w648) -> ("Path OUT"=w651:path)  [unwired: 1 in, 2 out]
        n225 = call <userlib>:"Append Image File.vi"("PDF Report IN"=w637, "Scale (%)"=w638, "Image path"=w649, "error in (no error)"=w636, "Caption"=w639) -> ("PDF Report OUT"=w622:refnum<class "PDF Report Class.lvclass">, "error out"=w621:errorcluster)  [unwired: 2 in, 7 out]
        n226 = call-poly <userlib>:"Append Text polymorphic.vi"("PDF Report"=w622, "Text"="Texte J3", "error in (no error)"=w621) -> ("PDF Report duplicate"=w619:refnum<class "PDF Report Class.lvclass">, "error out"=w620:errorcluster)  [unwired: 5 in, 6 out]
        n227 = call <userlib>:"Append Image File.vi"("PDF Report IN"=w619, "Scale (%)"=w638, "Image path"=w650, "error in (no error)"=w620, "Caption"=w640) -> ("PDF Report OUT"=w675:refnum<class "PDF Report Class.lvclass">, "error out"=w674:errorcluster)  [unwired: 2 in, 7 out]
        n228 = call <userlib>:"Append Image File.vi"("PDF Report IN"=w675, "Scale (%)"=w638, "Image path"=w665, "error in (no error)"=w674, "Caption"=w641) -> ("PDF Report OUT"=w631:refnum<class "PDF Report Class.lvclass">, "error out"=w630:errorcluster)  [unwired: 2 in, 7 out]
        n229 = call-poly <userlib>:"Append Text polymorphic.vi"("PDF Report"=w631, "Text [ ]"="Texte J4 [ ]", "error in (no error)"=w630) -> ("PDF Report duplicate"=w625:refnum<class "PDF Report Class.lvclass">, "error out"=w624:errorcluster)  [unwired: 2 in, 9 out]
        n230 = call <userlib>:"Append Image File.vi"("PDF Report IN"=w625, "Image path"=w651, "error in (no error)"=w624, "Caption"=w642) -> ("PDF Report OUT"=w627:refnum<class "PDF Report Class.lvclass">, "error out"=w626:errorcluster)  [unwired: 3 in, 7 out]
        n231 = call-poly <userlib>:"Append Text polymorphic.vi"("PDF Report"=w627, "Text [ ]"="Texte J5 [ ]", "error in (no error)"=w626) -> ("PDF Report duplicate"=w628:refnum<class "PDF Report Class.lvclass">, "error out"=w629:errorcluster)  [unwired: 2 in, 9 out]
        n232 = Unbundle("Image J5") -> ("Nom"=w652:path, "Légende"=w661:string)
        n233 = Unbundle("Image J6") -> ("Nom"=w653:path, "Légende"=w662:string)
        n234 = Unbundle("Image J7") -> ("Nom"=w655:path, "Légende"=w663:string)
        n235 = Unbundle("Image J8") -> ("Nom"=w668:path, "Légende"=w671:string)
        n236 = call <userlib>:"Update path.vi"("Path IN"=w652) -> ("Path OUT"=w658:path)  [unwired: 1 in, 2 out]
        n237 = call <userlib>:"Update path.vi"("Path IN"=w653) -> ("Path OUT"=w659:path)  [unwired: 1 in, 2 out]
        n238 = call <userlib>:"Update path.vi"("Path IN"=w655) -> ("Path OUT"=w660:path)  [unwired: 1 in, 2 out]
        n239 = call <userlib>:"Update path.vi"("Path IN"=w668) -> ("Path OUT"=w670:path)  [unwired: 1 in, 2 out]
        n240 = call <userlib>:"Append Image File.vi"("PDF Report IN"=w628, "Image path"=w658, "error in (no error)"=w629, "Caption"=w661) -> ("PDF Report OUT"=w616:refnum<class "PDF Report Class.lvclass">, "error out"=w615:errorcluster)  [unwired: 3 in, 7 out]
        n241 = call <userlib>:"Append Image File.vi"("PDF Report IN"=w616, "Image path"=w659, "error in (no error)"=w615, "Caption"=w662) -> ("PDF Report OUT"=w618:refnum<class "PDF Report Class.lvclass">, "error out"=w617:errorcluster)  [unwired: 3 in, 7 out]
        n242 = call <userlib>:"Append Image File.vi"("PDF Report IN"=w618, "Image path"=w660, "error in (no error)"=w617, "Caption"=w663) -> ("PDF Report OUT"=w666:refnum<class "PDF Report Class.lvclass">, "error out"=w667:errorcluster)  [unwired: 3 in, 7 out]
        n243 = call <userlib>:"Append Image File.vi"("PDF Report IN"=w666, "Image path"=w670, "error in (no error)"=w667, "Caption"=w671) -> ("PDF Report OUT"=w672:refnum<class "PDF Report Class.lvclass">, "error out"=w673:errorcluster)  [unwired: 3 in, 7 out]
        n244 = call <userlib>:"Append New Page.vi"("PDF Report"=w672, "error in (no error)"=w673) -> ("PDF Report duplicate"=w614:refnum<class "PDF Report Class.lvclass">, "error OUT"=w613:errorcluster)  [unwired: 12 out]
      }
      frame 13 {
        w690 = sgl 50.0  # Scale (%)
        # "J) Chapter 5, section 5.5 - Header, Footer and Watermark palette"
        # "Ajout d'images provenant de contrôles."
        # "Gras et italique"
        n245 = call-poly <userlib>:"Append Text polymorphic.vi"("PDF Report"=w695, "Text [ ]"="Texte J6 [ ]", "error in (no error)"=w694) -> ("PDF Report duplicate"=w680:refnum<class "PDF Report Class.lvclass">, "error out"=w679:errorcluster)  [unwired: 2 in, 9 out]
        n246 = control-ref of="Watermark Image"() -> (w678:refnum<vi>)
        n247 = call <userlib>:"Append Control Image.vi"("PDF Report IN"=w680, "Scale (%)"=w690, "Ctrl reference"=w678, "error in (no error)"=w679, "Caption"="Image J9") -> ("PDF Report OUT"=w685:refnum<class "PDF Report Class.lvclass">, "error out"=w686:errorcluster)  [unwired: 2 in, 7 out]
        n248 = control-ref of="Watermark Text"() -> (w691:refnum<vi>)
        n249 = call <userlib>:"Append Control Image.vi"("PDF Report IN"=w685, "Scale (%)"=w690, "Ctrl reference"=w691, "error in (no error)"=w686, "Caption"="Image J10") -> ("PDF Report OUT"=w688:refnum<class "PDF Report Class.lvclass">, "error out"=w687:errorcluster)  [unwired: 2 in, 7 out]
        n250 = call-poly <userlib>:"Append Text polymorphic.vi"("PDF Report"=w688, "Text"="TexteJ7", "error in (no error)"=w687, "Font"=T11 {"Name"="", "Size"=-1.0, "Color"=0, "Style"={"Bold"=TRUE, "Italic"=TRUE, "Underline"=FALSE, "Strikeout"=FALSE}, "Type"={"Type&direction"=enum."Select", "Embedded"=FALSE, "Encoding"=""}} ("Font complete")) -> ("PDF Report duplicate"=w677:refnum<class "PDF Report Class.lvclass">, "error out"=w676:errorcluster)  [unwired: 4 in, 6 out]
        n251 = call <userlib>:"Append New Page.vi"("PDF Report"=w677, "error in (no error)"=w676) -> ("PDF Report duplicate"=w692:refnum<class "PDF Report Class.lvclass">, "error OUT"=w693:errorcluster)  [unwired: 12 in]
      }
      frame 14 {
        w710 = sgl 55.0  # Scale (%)
        # "K) Chapter 5, section 5.6 - Concatenate palette"
        n252 = call <userlib>:"Append Chapter bookmark.vi"("PDF Report"=w696, "Chapter or section"=Chapter."Chapter - level 2", "Title"="Text k1", "error in (no error)"=w697) -> ("PDF Report duplicate"=w698:refnum<class "PDF Report Class.lvclass">, "error out"=w699:errorcluster)  [unwired: 10 in]
        n253 = call-poly <userlib>:"Append Text polymorphic.vi"("PDF Report"=w698, "Text [ ]"="Texte K2 [ ]", "error in (no error)"=w699) -> ("PDF Report duplicate"=w716:refnum<class "PDF Report Class.lvclass">, "error out"=w715:errorcluster)  [unwired: 2 in, 9 out]
        n254 = Unbundle("Image K1") -> ("Nom"=w719:path, "Légende"=w717:string)
        n255 = call <userlib>:"Update path.vi"("Path IN"=w719) -> ("Path OUT"=w720:path)  [unwired: 1 in, 2 out]
        n256 = call <userlib>:"Append Image File.vi"("PDF Report IN"=w716, "Scale (%)"=w710, "Image path"=w720, "error in (no error)"=w715, "Caption"=w717) -> ("PDF Report OUT"=w712:refnum<class "PDF Report Class.lvclass">, "error out"=w713:errorcluster)  [unwired: 2 in, 7 out]
        n257 = control-ref of="PDF Files  to concatenate and pages"() -> (w711:refnum<vi>)
        n258 = call <userlib>:"Append Control Image.vi"("PDF Report IN"=w712, "Scale (%)"=w710, "Ctrl reference"=w711, "error in (no error)"=w713, "Caption"="Image K2") -> ("PDF Report OUT"=w703:refnum<class "PDF Report Class.lvclass">, "error out"=w704:errorcluster)  [unwired: 9 in]
        n259 = call-poly <userlib>:"Append Text polymorphic.vi"("PDF Report"=w703, "Text [ ]"="Texte K3 [ ]", "error in (no error)"=w704) -> ("PDF Report duplicate"=w706:refnum<class "PDF Report Class.lvclass">, "error out"=w705:errorcluster)  [unwired: 2 in, 9 out]
        n260 = call <userlib>:"Append New Page.vi"("PDF Report"=w706, "error in (no error)"=w705) -> ("PDF Report duplicate"=w709:refnum<class "PDF Report Class.lvclass">, "error OUT"=w708:errorcluster)  [unwired: 12 in]
      }
      frame 15 {
        w724 = sgl 45.0  # Scale (%)
        w735 = sgl 35.0  # Scale (%)
        w757 = sgl 55.0  # Scale (%)
        # "L) Chapter 5, section 5.7 - Table of Contents palette"
        n261 = call <userlib>:"Append Chapter bookmark.vi"("PDF Report"=w762, "Chapter or section"=Chapter."Chapter - level 2", "Title"="Text L1", "error in (no error)"=w761) -> ("PDF Report duplicate"=w756:refnum<class "PDF Report Class.lvclass">, "error out"=w746:errorcluster)  [unwired: 10 in]
        n262 = call-poly <userlib>:"Append Text polymorphic.vi"("PDF Report IN"=w756, "Text"="Text L2", "error in (no error)"=w746) -> ("PDF Report OUT"=w754:refnum<class "PDF Report Class.lvclass">, "error out"=w745:errorcluster)  [unwired: 11 in]
        n263 = Unbundle("Image L1") -> ("Nom"=w759:path, "Légende"=w758:string)
        n264 = Unbundle("Image L3") -> ("Nom"=w739:path, "Légende"=w736:string)
        n265 = Unbundle("Image L2") -> ("Nom"=w750:path, "Légende"=w751:string)
        n266 = Unbundle("Image L4") -> ("Nom"=w727:path, "Légende"=w725:string)
        n267 = call <userlib>:"Update path.vi"("Path IN"=w759) -> ("Path OUT"=w760:path)  [unwired: 1 in, 2 out]
        n268 = call <userlib>:"Update path.vi"("Path IN"=w739) -> ("Path OUT"=w737:path)  [unwired: 1 in, 2 out]
        n269 = call <userlib>:"Update path.vi"("Path IN"=w750) -> ("Path OUT"=w749:path)  [unwired: 1 in, 2 out]
        n270 = call <userlib>:"Update path.vi"("Path IN"=w727) -> ("Path OUT"=w726:path)  [unwired: 1 in, 2 out]
        n271 = call <userlib>:"Append Image File.vi"("PDF Report IN"=w754, "Scale (%)"=w757, "Image path"=w760, "error in (no error)"=w745, "Caption"=w758) -> ("PDF Report OUT"=w748:refnum<class "PDF Report Class.lvclass">, "error out"=w747:errorcluster)  [unwired: 2 in, 7 out]
        n272 = call <userlib>:"Append Image File.vi"("PDF Report IN"=w748, "Scale (%)"=w724, "Image path"=w749, "error in (no error)"=w747, "Caption"=w751) -> ("PDF Report OUT"=w743:refnum<class "PDF Report Class.lvclass">, "error out"=w742:errorcluster)  [unwired: 2 in, 7 out]
        n273 = call-poly <userlib>:"Append Text polymorphic.vi"("PDF Report IN"=w743, "Text"="Text L3", "error in (no error)"=w742) -> ("PDF Report OUT"=w740:refnum<class "PDF Report Class.lvclass">, "error out"=w741:errorcluster)  [unwired: 11 in]
        n274 = call <userlib>:"Append Image File.vi"("PDF Report IN"=w740, "Scale (%)"=w735, "Image path"=w737, "error in (no error)"=w741, "Caption"=w736) -> ("PDF Report OUT"=w732:refnum<class "PDF Report Class.lvclass">, "error out"=w733:errorcluster)  [unwired: 2 in, 7 out]
        n275 = call-poly <userlib>:"Append Text polymorphic.vi"("PDF Report IN"=w732, "Text"="Text L4", "error in (no error)"=w733) -> ("PDF Report OUT"=w730:refnum<class "PDF Report Class.lvclass">, "error out"=w731:errorcluster)  [unwired: 11 in]
        n276 = call <userlib>:"Append Image File.vi"("PDF Report IN"=w730, "Scale (%)"=w724, "Image path"=w726, "error in (no error)"=w731, "Caption"=w725) -> ("PDF Report OUT"=w729:refnum<class "PDF Report Class.lvclass">, "error out"=w722:errorcluster)  [unwired: 2 in, 7 out]
        n277 = call <userlib>:"Append New Page.vi"("PDF Report"=w729, "error in (no error)"=w722) -> ("PDF Report duplicate"=w723:refnum<class "PDF Report Class.lvclass">, "error OUT"=w721:errorcluster)  [unwired: 12 in]
      }
      frame 16 {
        w775 = sgl 55.0  # Scale (%)
        # "M) Chapter 5, section 5.8 - Tools palette"
        n278 = call <userlib>:"Append Chapter bookmark.vi"("PDF Report"=w770, "Chapter or section"=Chapter."Chapter - level 2", "Title"="Text M1", "error in (no error)"=w771) -> ("PDF Report duplicate"=w773:refnum<class "PDF Report Class.lvclass">, "error out"=w774:errorcluster)  [unwired: 10 in]
        n279 = Unbundle("Image M1") -> ("Nom"=w777:path, "Légende"=w776:string)
        n280 = call <userlib>:"Update path.vi"("Path IN"=w777) -> ("Path OUT"=w778:path)  [unwired: 1 in, 2 out]
        n281 = call <userlib>:"Append Image File.vi"("PDF Report IN"=w773, "Scale (%)"=w775, "Image path"=w778, "error in (no error)"=w774, "Caption"=w776) -> ("PDF Report OUT"=w769:refnum<class "PDF Report Class.lvclass">, "error out"=w767:errorcluster)  [unwired: 2 in, 7 out]
        n282 = call-poly <userlib>:"Append Text polymorphic.vi"("PDF Report"=w769, "Text"="Text M2", "error in (no error)"=w767) -> ("PDF Report duplicate"=w768:refnum<class "PDF Report Class.lvclass">, "error out"=w766:errorcluster)  [unwired: 11 in]
      }
      frame 17 {
        w801 = sgl 60.0  # Scale (%)
        w815 = sgl 35.0  # Scale (%)
        w827 = sgl 33.0  # Scale (%)
        w833 = sgl 23.0  # Scale (%)
        # "N) Chapter 6 - Unicode with PDF Report"
        n283 = call <userlib>:"Append Chapter bookmark.vi"("PDF Report"=w793, "Chapter or section"=Chapter."Chapter - level 1", "Title"="Text N1", "error in (no error)"=w792, "Font"="Font N1") -> ("PDF Report duplicate"=w787:refnum<class "PDF Report Class.lvclass">, "error out"=w786:errorcluster)  [unwired: 9 in]
        n284 = call-poly <userlib>:"Append Text polymorphic.vi"("PDF Report"=w787, "Text"="Text N2", "Font"="Font N1") -> ("PDF Report duplicate"=w783:refnum<class "PDF Report Class.lvclass">)  [unwired: 11 in, 1 out]
        n285 = call <userlib>:"Append Chapter bookmark.vi"("PDF Report"=w783, "Chapter or section"=Chapter."Chapter - level 2", "Title"="Text N3", "error in (no error)"=w786) -> ("PDF Report duplicate"=w788:refnum<class "PDF Report Class.lvclass">, "error out"=w789:errorcluster)  [unwired: 10 in]
        n286 = call-poly <userlib>:"Append Text polymorphic.vi"("PDF Report"=w788, "Text [ ]"="Texte N4 [ ]", "error in (no error)"=w789) -> ("PDF Report duplicate"=w830:refnum<class "PDF Report Class.lvclass">, "error out"=w831:errorcluster)  [unwired: 2 in, 9 out]
        n287 = Unbundle("Image N1") -> ("Nom"=w835:path, "Légende"=w834:string)
        n288 = call <userlib>:"Update path.vi"("Path IN"=w835) -> ("Path OUT"=w836:path)  [unwired: 1 in, 2 out]
        n289 = call <userlib>:"Append Image File.vi"("PDF Report IN"=w830, "Scale (%)"=w833, "Image path"=w836, "error in (no error)"=w831, "Caption"=w834) -> ("PDF Report OUT"=w821:refnum<class "PDF Report Class.lvclass">, "error out"=w822:errorcluster)  [unwired: 2 in, 7 out]
        n290 = Unbundle("Image N2") -> ("Nom"=w825:path, "Légende"=w826:string)
        n291 = call-poly <userlib>:"Append Text polymorphic.vi"("PDF Report"=w821, "Text"="Text N5", "error in (no error)"=w822) -> ("PDF Report duplicate"=w820:refnum<class "PDF Report Class.lvclass">, "error out"=w819:errorcluster)  [unwired: 5 in, 6 out]
        n292 = call <userlib>:"Update path.vi"("Path IN"=w825) -> ("Path OUT"=w824:path)  [unwired: 1 in, 2 out]
        n293 = call <userlib>:"Append Image File.vi"("PDF Report IN"=w820, "Scale (%)"=w827, "Image path"=w824, "error in (no error)"=w819, "Caption"=w826) -> ("PDF Report OUT"=w811:refnum<class "PDF Report Class.lvclass">, "error out"=w812:errorcluster)  [unwired: 2 in, 7 out]
        n294 = call-poly <userlib>:"Append Text polymorphic.vi"("PDF Report"=w811, "Text"="Text N6", "error in (no error)"=w812) -> ("PDF Report duplicate"=w809:refnum<class "PDF Report Class.lvclass">, "error out"=w810:errorcluster)  [unwired: 5 in, 6 out]
        n295 = Unbundle("Image N3") -> ("Nom"=w817:path, "Légende"=w816:string)
        n296 = call <userlib>:"Update path.vi"("Path IN"=w817) -> ("Path OUT"=w818:path)  [unwired: 1 in, 2 out]
        n297 = call <userlib>:"Append Image File.vi"("PDF Report IN"=w809, "Scale (%)"=w815, "Image path"=w818, "error in (no error)"=w810, "Caption"=w816) -> ("PDF Report OUT"=w807:refnum<class "PDF Report Class.lvclass">, "error out"=w808:errorcluster)  [unwired: 2 in, 7 out]
        n298 = call-poly <userlib>:"Append Text polymorphic.vi"("PDF Report"=w807, "Text"="Text N7", "error in (no error)"=w808) -> ("PDF Report duplicate"=w805:refnum<class "PDF Report Class.lvclass">, "error out"=w804:errorcluster)  [unwired: 5 in, 6 out]
        n299 = control-ref of="Text N9"() -> (w803:refnum<vi>)
        n300 = call <userlib>:"Append Control Image.vi"("PDF Report IN"=w805, "Scale (%)"=w801, "Ctrl reference"=w803, "error in (no error)"=w804, "Caption"="Image N4") -> ("PDF Report OUT"=w799:refnum<class "PDF Report Class.lvclass">, "error out"=w800:errorcluster)  [unwired: 9 in]
        n301 = call-poly <userlib>:"Append Text polymorphic.vi"("PDF Report"=w799, "Text"="Text N8", "error in (no error)"=w800) -> ("PDF Report duplicate"=w796:refnum<class "PDF Report Class.lvclass">, "error out"=w797:errorcluster)  [unwired: 5 in, 6 out]
        n302 = call-poly <userlib>:"Append Text polymorphic.vi"("PDF Report"=w796, "Text"="Text N9", "error in (no error)"=w797, "Font"="Font N1") -> ("PDF Report duplicate"=w790:refnum<class "PDF Report Class.lvclass">, "error out"=w791:errorcluster)  [unwired: 5 in, 5 out]
      }
      frame 18 {
        w875 = sgl 35.0  # Scale (%)
        n303 = Unbundle("Image N5") -> ("Nom"=w877:path, "Légende"=w876:string)
        n304 = call-poly <userlib>:"Append Text polymorphic.vi"("PDF Report"=w869, "Text"="Text N10", "error in (no error)"=w870) -> ("PDF Report duplicate"=w873:refnum<class "PDF Report Class.lvclass">, "error out"=w872:errorcluster)  [unwired: 5 in, 6 out]
        n305 = call <userlib>:"Update path.vi"("Path IN"=w877) -> ("Path OUT"=w871:path)  [unwired: 1 in, 2 out]
        n306 = call <userlib>:"Append Image File.vi"("PDF Report IN"=w873, "Scale (%)"=w875, "Image path"=w871, "error in (no error)"=w872, "Caption"=w876) -> ("PDF Report OUT"=w866:refnum<class "PDF Report Class.lvclass">, "error out"=w853:errorcluster)  [unwired: 2 in, 7 out]
        n307 = call <userlib>:"Append New Page.vi"("PDF Report"=w866, "error in (no error)"=w853) -> ("PDF Report duplicate"=w854:refnum<class "PDF Report Class.lvclass">, "error OUT"=w852:errorcluster)  [unwired: 12 in]
        n308 = call <userlib>:"Append Chapter bookmark.vi"("PDF Report"=w854, "Chapter or section"=Chapter."Chapter - level 2", "Title"="Text N11", "error in (no error)"=w852) -> ("PDF Report duplicate"=w856:refnum<class "PDF Report Class.lvclass">, "error out"=w855:errorcluster)  [unwired: 10 in]
        n309 = call <userlib>:"Create Table.vi"("PDF Report IN"=w856, "Table columnWidth [ ]"="Table columnWidth [ ] - Table 7", "Column Headers 2D [ ]"="Column Headers 2D [ ] - Table 7", "Row Headers 1D [ ]"="Row Headers 1D [ ] - Table 7", "Text Data 2D [ ]"="Text Data 2D [ ] - Table 7", "error in (no error)"=w855) -> ("PDF Report duplicate"=w864:refnum<class "PDF Report Class.lvclass">, "PDF Table"=w861:refnum<class "Pdfp Table Class.lvclass">, "error out"=w865:errorcluster)  [unwired: 7 in]
        n310 = call <userlib>:"Append Customized Table.vi"("PDF Report IN"=w864, "Table properties"="Table properties - Table 7", "PDF Table"=w861, "error in (no error)"=w865, "Row  [ ]"="Row  [ ] - Table 7") -> ("PDF Report OUT"=w843:refnum<class "PDF Report Class.lvclass">, "error out"=w842:errorcluster)  [unwired: 9 in]
        n311 = call <userlib>:"Append LF.vi"("PDF Report IN"=w843, "error in (no error)"=w842) -> ("PDF Report duplicate"=w840:refnum<class "PDF Report Class.lvclass">, "error out"=w841:errorcluster)  [unwired: 12 in]
        n312 = call <userlib>:"Create Table.vi"("PDF Report IN"=w840, "Table columnWidth [ ]"="Table columnWidth [ ] - Table 8", "Row Headers 1D [ ]"="Row Headers 1D [ ] - Table 8", "Text Data 2D [ ]"="Text Data 2D [ ] - Table 8", "error in (no error)"=w841) -> ("PDF Report duplicate"=w850:refnum<class "PDF Report Class.lvclass">, "PDF Table"=w848:refnum<class "Pdfp Table Class.lvclass">, "error out"=w851:errorcluster)  [unwired: 8 in]
        n313 = call <userlib>:"Append Customized Table.vi"("PDF Report IN"=w850, "Table properties"="Table properties - Table 8", "PDF Table"=w848, "error in (no error)"=w851, "Row  [ ]"="Row  [ ] - Table 8") -> ("PDF Report OUT"=w838:refnum<class "PDF Report Class.lvclass">, "error out"=w839:errorcluster)  [unwired: 9 in]
      }
      frame 19 {
        # "O) Chapter 7"
        n314 = call <userlib>:"Append Chapter bookmark.vi"("PDF Report"=w883, "Chapter or section"=Chapter."Chapter - level 1", "Title"="Text O1", "error in (no error)"=w882) -> ("PDF Report duplicate"=w884:refnum<class "PDF Report Class.lvclass">, "error out"=w885:errorcluster)  [unwired: 10 in]
        n315 = call-poly <userlib>:"Append Text polymorphic.vi"("PDF Report"=w884, "Text [ ]"="Text O2 [ ]", "error in (no error)"=w885) -> ("PDF Report duplicate"=w890:refnum<class "PDF Report Class.lvclass">, "error out"=w889:errorcluster)  [unwired: 2 in, 9 out]
        n316 = call <userlib>:"Append LF.vi"("PDF Report IN"=w890, "Number of LF (default 1)"=u8 3, "error in (no error)"=w889) -> ("PDF Report duplicate"=w886:refnum<class "PDF Report Class.lvclass">, "error out"=w887:errorcluster)  [unwired: 11 in]
        n317 = call <userlib>:"Append PDF file to PDF Report .vi"("PDF Report"=w886, "PDF Files  to concatenate and pages"="PDF Files  to concatenate and pages", "error in (no error)"=w887) -> ("PDF Report duplicate"=w893:refnum<class "PDF Report Class.lvclass">, "error out"=w892:errorcluster)  [unwired: 11 in]
      }
      frame 20 {
        w899 = "\"" ("string")
        # "It is here that are added the the Table of Contents, the headers, footers and watermark. Furthermore, it is here that are concatenated the PDF files.\n在这里添加了目录、页眉、页脚和水印。此外，正是在这里连接了PDF文件。"
        # "L) Closing PDF Report"
        n318 = call <userlib>:"Close PDF.vi"("PDF Report"=w903, "error in (no error)"=w904) -> ("Path"=w896:path, "error out"=w895:errorcluster)  [unwired: 12 out]
        "PDF 输出路径" <- w896
        n319 = Path To String(path=w896) -> (string=w901:string)
        n320 = Concatenate Strings("cmd /c " ("string"), w899, w901, w899) -> (w902:string)
        n321 = call <vilib>:"System Exec.vi"("run minimized? (F)"=TRUE, "wait until completion? (T)"=FALSE, "error in (no error)"=w895, "command line"=w902) -> ("error out"=w894:errorcluster)  [unwired: 2 in, 5 out]
      }
    }
    n322 = Subtract(x=w8, y=w7) -> (x-y=w9:u32)
    n323 = expression code="x/1000"(w9) -> (→"秒":u32)
    "Progress" <- w10
  }
  "error out" <- w5
